vi "GainCurveMeasurement.vi"() -> ()   [LabVIEW 2020]
doc: "Main VI for FLS imaging system."
uses:
  <userlib>/_OpenG.lib/file/file.llb/openg_file.lvlib
  <vilib>/event_ctls.llb/usereventprio.ctl
  <instrlib>/niScope/Acquire/Fetch/niScope Multi Fetch Binary 16.vi
  <instrlib>/niScope/Controls/niScope trigger source.ctl
  <userlib>/_OpenG.lib/time/time.llb/openg_time.lvlib
  <vilib>/Utility/file.llb/Write Delimited Spreadsheet (DBL).vi
  LaguerreDeconLib/DeconEngineClass/LaguerreDeconEngineClass.lvclass
  SubVI/GlobalVariables.vi
  SubVI/LabJack/LJ Pin Setting.ctl
  <vilib>/Utility/error.llb/DialogType.ctl
  <vilib>/Analysis/NI_AALBase.lvlib
  <vilib>/Utility/miscctls.llb/LVMinMaxIncTypeDef.ctl
  <vilib>/Analysis/baseanly.llb/Mean (DBL).vi
  <vilib>/Utility/miscctls.llb/LVPointTypeDef.ctl
  <vilib>/Instr/_visa.llb/VISA Configure Serial Port (Instr).vi
  SubVI/DigitizerConfiguration/FLImDAQ.ctl
panel:
  out "Record Backlog":i32
  out "Fetch Record #":i32
  out "error out 2":errorcluster caption="error out"
  out "error out":errorcluster
  out "Sync Success?":bool
  out "Disclamer":picture
  out "Calibration #":i8
  out "BG #":i8
  in  "TCP Connect":bool
  out "Help":string
  in  "355nm Laser toggle":bool caption="355nm 750Hz"
  in  "Cali&iRF alignment":bool
  in  "Background":bool
  in  "Aiming beam toggle":bool caption="445nm 15Hz 20mA"
  out "Lifetime 3":dbl
  out "Lifetime 2":dbl
  in  "Auto gain ch3":bool=TRUE
  in  "Auto gain ch2":bool=TRUE
  in  "Auto gain ch1":bool=TRUE
  out "Run #":i8
  in  "StopButton":bool caption="Stop"
  out "Aquisition Status:":bool
  in  "StartButton":bool caption="Start"
  in  "Gain 3":dbl min=0.0 max=4.6 step=0.1
  in  "Gain 2":dbl min=0.0 max=4.6 step=0.1
  out "Lifetime 1":dbl
  in  "Gain 1":dbl min=0.0 max=4.6 step=0.1 format="%#_4g"
  in  "Video Source":enum32{"Camera", "FrameGrabber"}(radio)
  out "Case #":string
  out "System Hardware Connection Status":T1
  out "Channel 3":dbl[][](graph)
  out "Channel 2":dbl[][](graph)
  out "Channel 1":dbl[][](graph)
  in  "Tab Control":T2(tab)
  out "Aq L?":bool
  out "ML?":bool
  out "display loop timing(ms)":u32
  out "Aquisition loop timing(ms)":u32
  in  "sine offset":dbl min=0.0 max=4.8 step=0.01
  in  "sine amplitude":dbl
  out "DisplayLoop":i32
  out "processing loop":i32
  out "processing loop timing(ms)":dbl
  in  "V target(1.5)":dbl=1.3 format="%#_13g"
  out "comm loop(ms)":u32
  out "laser EM lamp V":dbl format="%0.6f"
  in  "Show BG":bool
  in  "start Idx":i32
  in  "length":i32=50
  out "SysConfigCluster":T3
  out "LJ Pinout":T4={"Ch1 Bias"="DAC0", "Ch2 Bias"="DAC1", "Ch3 Bias"="DAC2", "Ch4 Bias"="DAC0", "355 PWM"="FIO0", "AimingBeam PWM"="FIO2", "Laser Ready"="FIO3", "Interlock"="FIO1", "Laser Start/Stop"="FIO1", "Red LED"="FIO1", "Green LED"="DIO3", "Foot Pedal"="DIO15"}
  out "FLImDAQ":T5={"Digitizer 1"="", "Digitizer 2"="", "Channel"=enum."Channel 0", "trigger source"="VAL_EXTERNAL", "trigger level"=0.5, "trigger delay"=1.35e-07, "min sample rate"=12500000000.0, "min record length"=2500, "vertical range"=1.0, "vertical offset"=-0.25, "Waveform to Avg"=2000} caption="FLIm DAQ Configuration" {"trigger delay" format="%^#.4e"; "trigger level" min=0.0 max=3.5 step=0.5 format="%.2f"; "vertical offset" format="%.4f"; "vertical range" format="%.2f"; "min sample rate" format="%#.2p"}
  out "Dig1 Temp":dbl
  out "Dig2 Temp":dbl
  in  "Sys Reconfig":bool
  out "data out(communcation loop)":string
  out "syctimer data out":string
  out "processing Error Out":errorcluster
  out "aquisition loop Error Out":errorcluster
  out "decon error out":errorcluster
  out "V1":dbl[](array[numeric])
  out "V2":dbl[](array[numeric])
  out "V3":dbl[](array[numeric])
  out "V1 Size":i32
  out "V2 Size":i32
  out "V3 Size":i32
  out "data Size":i32[](array[numeric])
  out "State log":string
  in  "Quit":bool
  in  "Radio Buttons":enum32{"No Selection", "Ch1", "Ch2", "Ch3"}(radio)=enum."Ch1" caption="DeCon Chan"
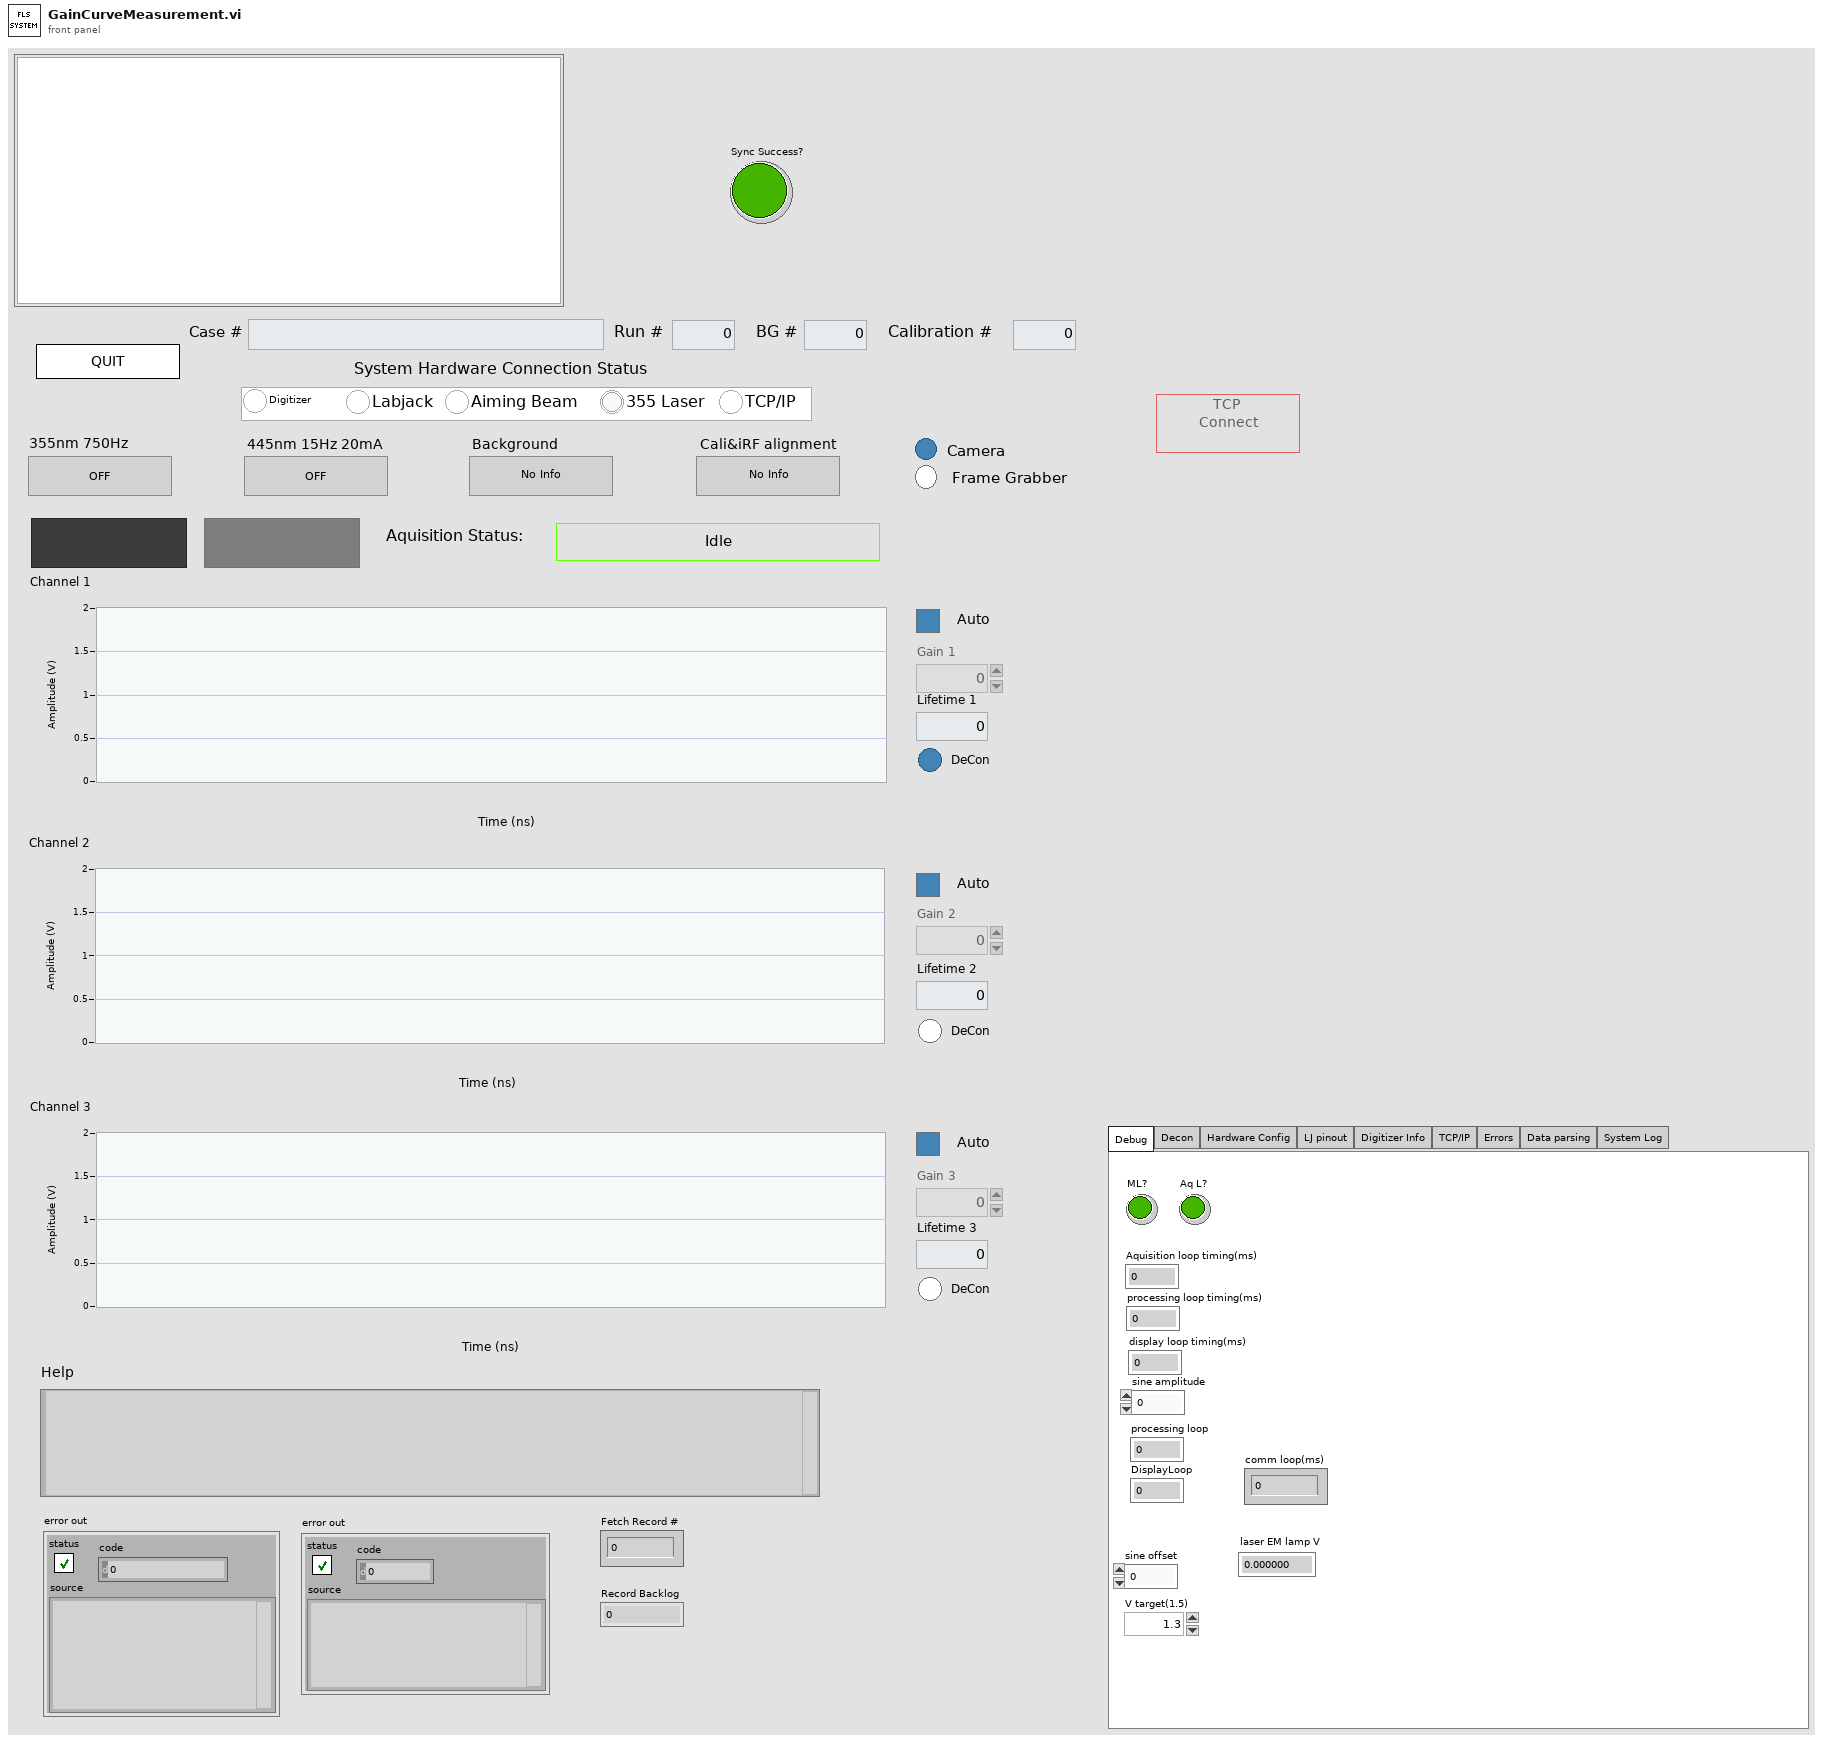
[diagram p1: front panel]
types:
  T1 = cluster{"Digitizer":bool, "Labjack":bool, "Aiming Beam":bool, "355 Laser":bool, "TCP/IP":bool}
  T2 = enum32{"Debug", "Decon", "Hardware Config", "LJ pinout", "Digitizer Info", "TCP/IP", "Errors", "Data parsing", "System Log"}
  T3 = cluster{"Ch1Enable?":bool, "Ch2Enable?":bool, "Ch3Enable?":bool, "Ch1AutoGain?":bool, "Ch2AutoGain?":bool, "Ch3AutoGain?":bool, "AimingBeamEnable?":bool}
  T4 = typedef "LJ Pin Setting.ctl" = cluster{"Ch1 Bias":string, "Ch2 Bias":string, "Ch3 Bias":string, "Ch4 Bias":string, "355 PWM":string, "AimingBeam PWM":string, "Laser Ready":string, "Interlock":string, "Laser Start/Stop":string, "Red LED":string, "Green LED":string, "Foot Pedal":string}
  T5 = typedef "FLImDAQ.ctl" = cluster{"Digitizer 1":refnum<k15>, "Digitizer 2":refnum<k15>, "Channel":enum16{"Channel 0", "Channel 1", "Channel 0&1"}, "trigger source":T6, "trigger level":dbl, "trigger delay":dbl, "min sample rate":dbl, "min record length":i32, "vertical range":dbl, "vertical offset":dbl, "Waveform to Avg":i16}
  T6 = typedef "niScope trigger source.ctl" = string
  T7 = typedef "LVPointTypeDef.ctl" = cluster{"Horizontal":i16, "Vertical":i16}
  T8 = cluster{"CH1":dbl[][], "CH2":dbl[][], "CH3":dbl[][]}
  T9 = cluster{"idx":i32, "CH1&2":dbl[][], "CH3":dbl[][]}
  T10 = enum8{"Enabled", "Disabled", "Disabled and Grayed Out"}
  T11 = enum16{"open", "open or create", "create or replace", "create", "open (read-only)"}
  T12 = enum32{"Invalid", "Standard", "Closed", "Hidden", "Minimized", "Maximized"}
  T13 = enum32{"invalid app kind", "Development System", "Run Time System", "Student Edition", "Embedded LabVIEW", "Evaluation", "Custom"}
  T14 = typedef "usereventprio.ctl" = enum32{"high priority", "normal priority"}
  T15 = enum16{"Standard", "Buffered", "CRLF", "Immediate"}
  T16 = cluster{"Core":cluster{"Current VI Reference":refnum<vi>, "Close Panel on Exit?":bool}, "SysConfigCluster":cluster{"Ch1Enable?":bool, "Ch2Enable?":bool, "Ch3Enable?":bool, "Ch1AutoGain?":bool, "Ch2AutoGain?":bool, "Ch3AutoGain?":bool, "AimingBeamEnable?":bool}, "System Status":cluster{"Digitizer":bool, "Labjack":bool, "Aiming Beam":bool, "355 Laser":bool, "TCP/IP":bool}, "IDs":cluster{"RunID":i8, "BG ID":i8, "Cali ID":i8}, "CaseID":string, "DefaultPath":path, "Pathes":cluster{"DataPath":path, "BG Path":path, "iRFPath":path, "CaliPath":path}, "FLImDAQ":cluster{"resource name":refnum<k15>, "resource name 2":refnum<k15>, "Channel":enum16{"Channel 0", "Channel 1", "Channel 0&1"}, "trigger source":T6, "trigger level":dbl, "trigger delay":dbl, "min sample rate":dbl, "min record length":i32, "vertical range":dbl, "vertical offset":dbl, "Waveform to Avg":i32}, "SysRunning?":bool, "AB Cluster":cluster{"Aiming Beam COM Port":refnum<visa-resource-name>, "Min Current":dbl, "Max Current":dbl, "Default Current":dbl, i32}, "LJ Pinout":T4, "355 PWM setting":cluster{"DIO_EF_CLOCK1_DIVISOR":i16, "DIO_EF_CLOCK1_ROLL_VALUE":i32, "DIO#_EF_INDEX":i16, "DIO#_EF_OPTIONS":i16, "DIO#_EF_CONFIG_A":i32}, "AB PWM setting":cluster{"DIO_EF_CLOCK1_DIVISOR":i16, "DIO_EF_CLOCK1_ROLL_VALUE":i32, "DIO#_EF_INDEX":i16, "DIO#_EF_OPTIONS":i16, "DIO#_EF_CONFIG_A":i32}, "Last Trigger":u32, "niTClk sessions":refnum<k20>[], "Laser start tic":u32, "TCP attempt count":i32, "Ch1Data":dbl[][], "Ch2Data":dbl[][], "Ch3Data":dbl[][], "V1":dbl[], "V2":dbl[], "V3":dbl[], "SlowTimer":u32, "FastTimer":u32, "listener ID":refnum<k5>, "TempPath":path, "LED vi reference":refnum<vi>}
  T17 = typedef "LVCursorListTypeDef.ctl" = cluster{"Name":string, "Color":u32, "Style":u8, "Point Style":u8, "Name Visible":bool, "Allow Drag":bool, "Cursor Mode":u32, "Plot":i32, "Index":i32, "Position":cluster{"X":dbl, "Y":dbl}, "X Scale":u32, "Y Scale":u32, "Watch Plots":i32[], "Watch All Plots":bool, "Plot Area":i32, "Label Offset":cluster{"X":dbl, "Y":dbl}}[]
  T18 = cluster{"Name":string, "Color":u32, "Style":u8, "Point Style":u8, "Name Visible":bool, "Allow Drag":bool, "Cursor Mode":u32, "Plot":i32, "Index":i32, "Position":cluster{"X":dbl, "Y":dbl}, "X Scale":u32, "Y Scale":u32, "Watch Plots":i32[], "Watch All Plots":bool, "Plot Area":i32, "Label Offset":cluster{"X":dbl, "Y":dbl}}
  T19 = cluster{"DataPath":path, "BG Path":path, "iRFPath":path, "CaliPath":path}
  T20 = cluster{"DIO_EF_CLOCK1_DIVISOR":i16, "DIO_EF_CLOCK1_ROLL_VALUE":i32, "DIO#_EF_INDEX":i16, "DIO#_EF_OPTIONS":i16, "DIO#_EF_CONFIG_A":i32}
  T21 = cluster{"Aiming Beam COM Port":refnum<visa-resource-name>, "Min Current":dbl, "Max Current":dbl, "Default Current":dbl, i32}
  T22 = cluster{"resource name":refnum<k15>, "resource name 2":refnum<k15>, "Channel":enum16{"Channel 0", "Channel 1", "Channel 0&1"}, "trigger source":T6, "trigger level":dbl, "trigger delay":dbl, "min sample rate":dbl, "min record length":i32, "vertical range":dbl, "vertical offset":dbl, "Waveform to Avg":i32}
  T23 = cluster{"Current VI Reference":refnum<vi>, "Close Panel on Exit?":bool}
  T24 = cluster{"1D Avg out":dbl[], "1D Avg out":dbl[], "1D Avg out":dbl[]}
  T25 = typedef "DialogType.ctl" = u16
  T26 = cluster{"Ch1 iRF":dbl[], "Ch2 iRF":dbl[], "Ch3 iRF":dbl[], "Ch4 iRF":dbl[]}
  T27 = typedef "LJ PWM Setting.ctl" = cluster{"DIO_EF_CLOCK1_DIVISOR":i16, "DIO_EF_CLOCK1_ROLL_VALUE":i32, "DIO#_EF_INDEX":i16, "DIO#_EF_OPTIONS":i16, "DIO#_EF_CONFIG_A":i32}
  T28 = typedef "AimingBeam.ctl" = cluster{"Aiming Beam COM Port":refnum<visa-resource-name>, "Min Current":dbl, "Max Current":dbl, "Default Current":dbl, "Frequency(Hz)":u32}
  T29 = typedef "LVMinMaxIncTypeDef.ctl" = cluster{"Minimum":dbl, "Maximum":dbl, "Increment":dbl}
  T30 = typedef "LVBoundsTypeDef.ctl" = cluster{"Width":u32, "Height":u32}
  T31 = typedef "imagedata.ctl" = cluster{"image type":i32, "image depth":i32, "image":u8[], "mask":u8[], "colors":u32[], "Rectangle":cluster{"left":i16, "top":i16, "right":i16, "bottom":i16}}
  T32 = enum32{"No Selection", "Ch1", "Ch2", "Ch3", "Ch4"}
  T33 = cluster{"V1 out":dbl, "V2 out":dbl, "V3 out":dbl}
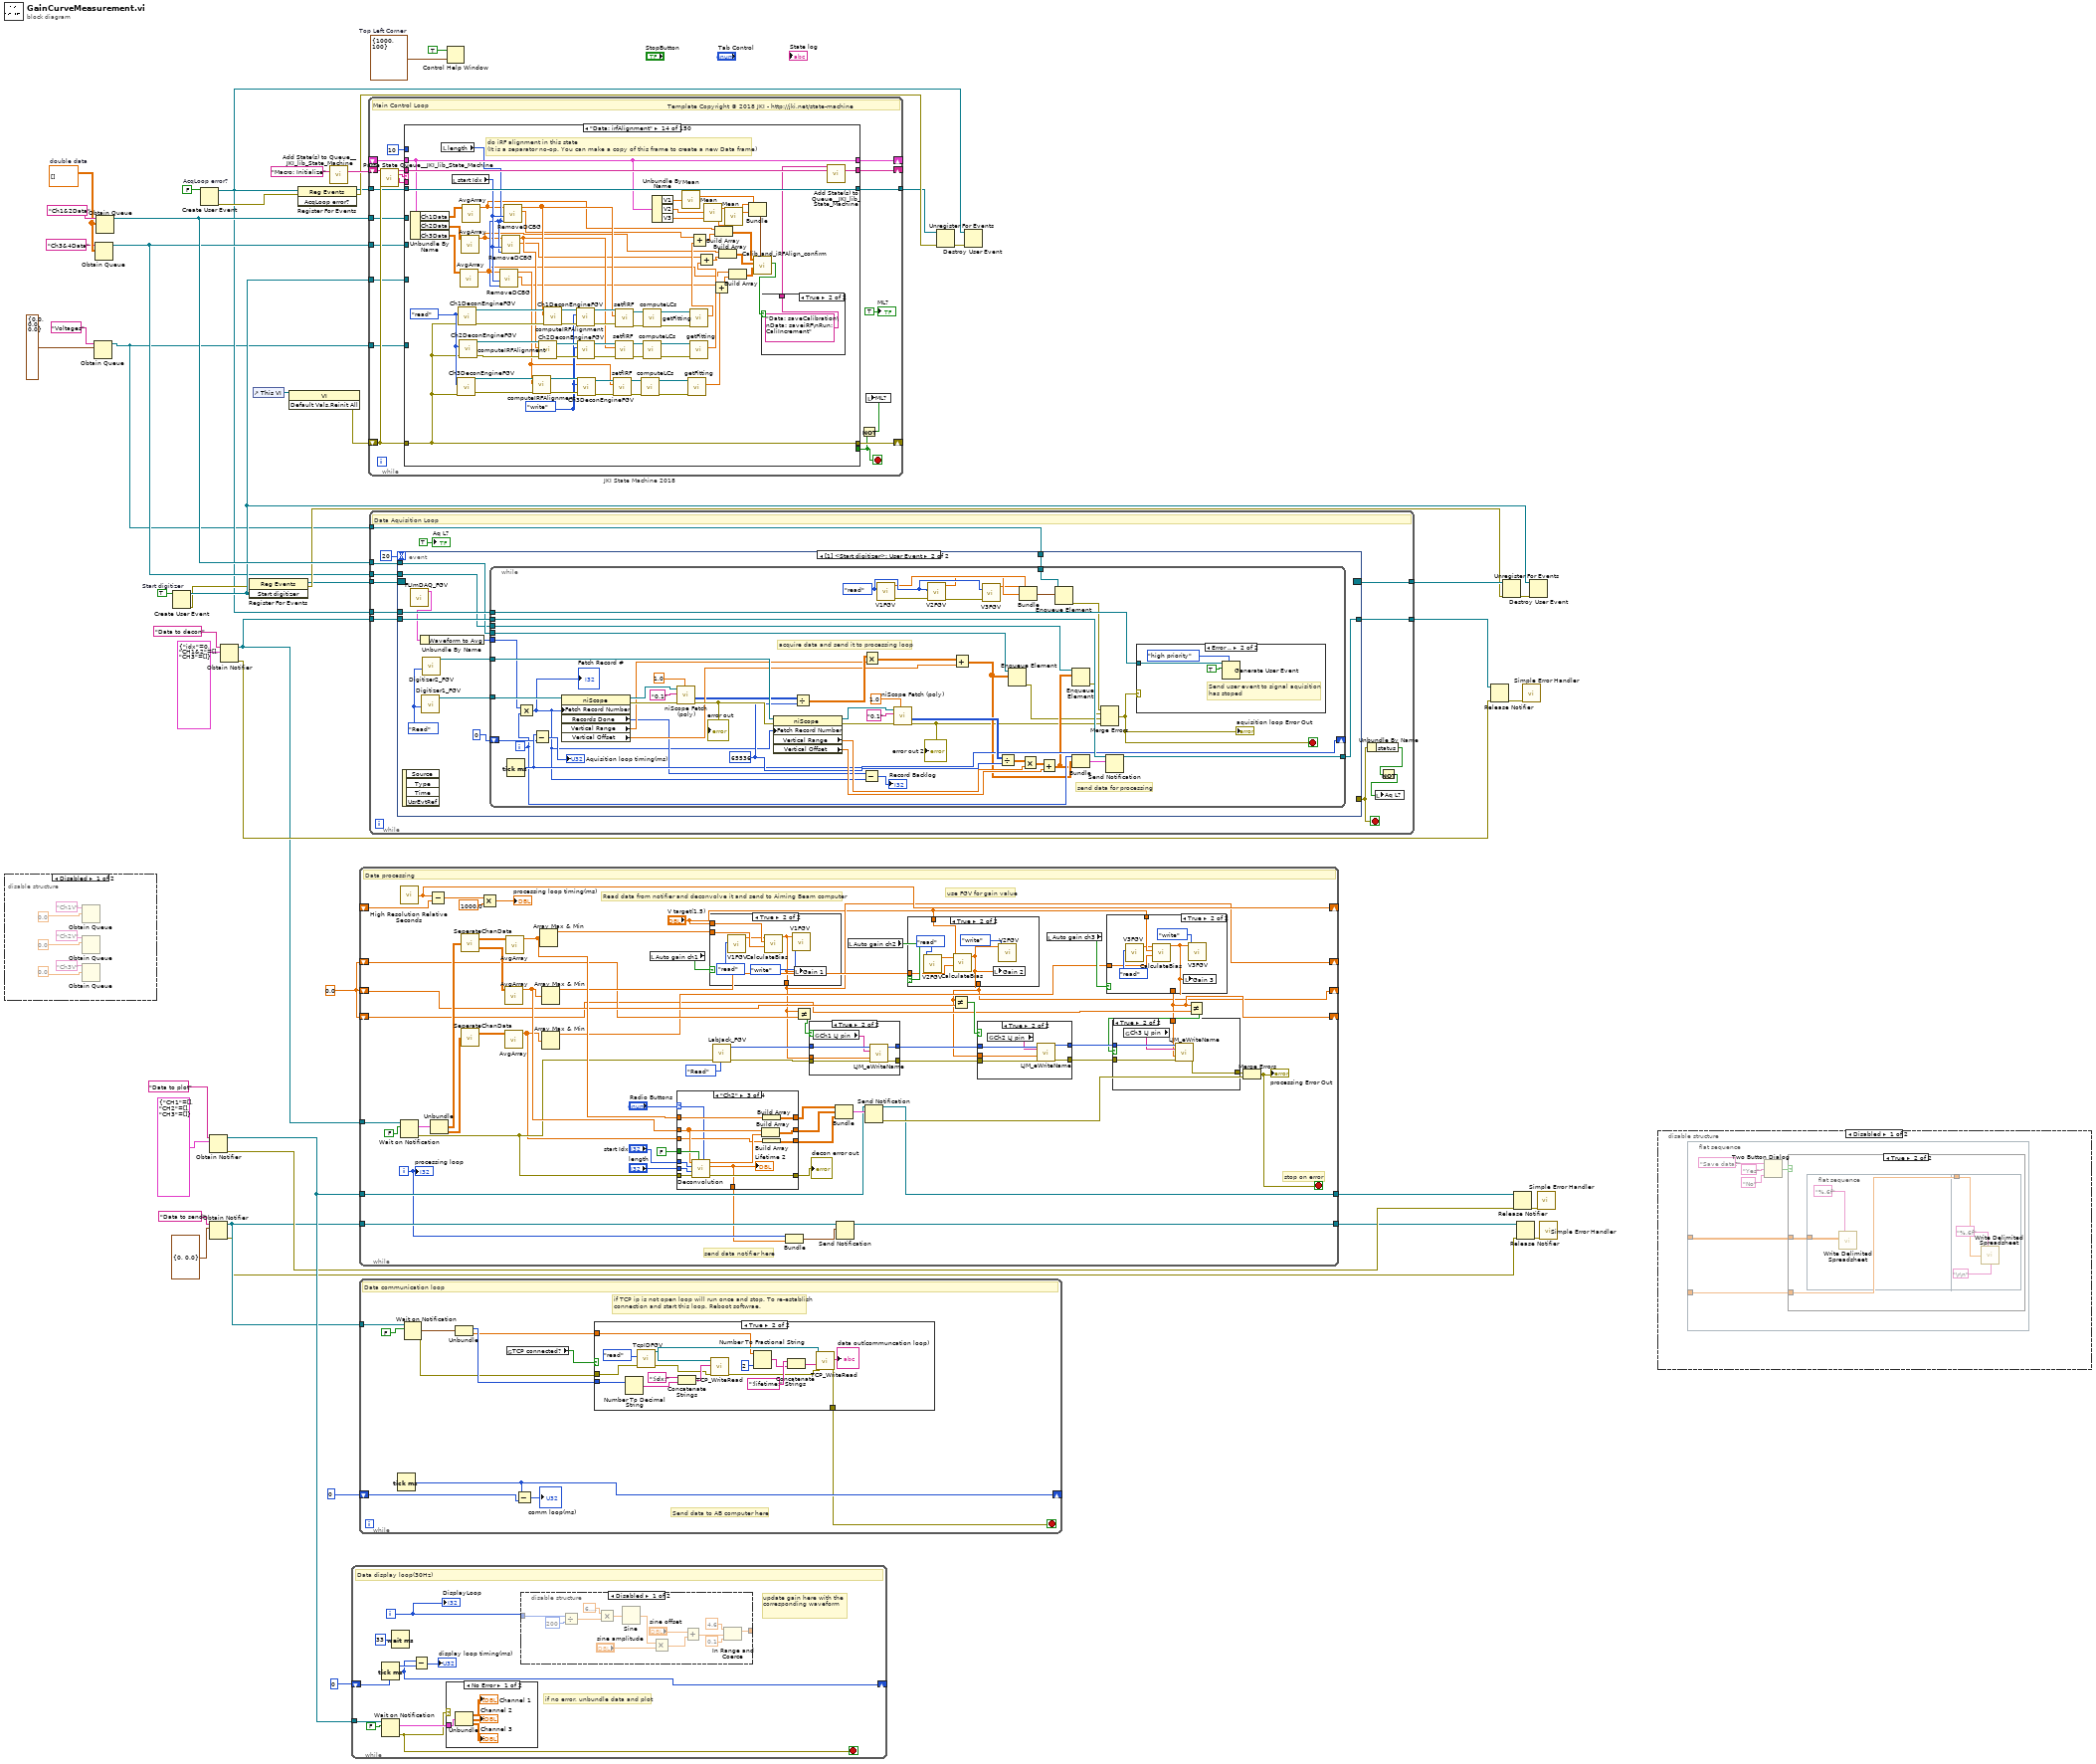
[diagram p0: block diagram]
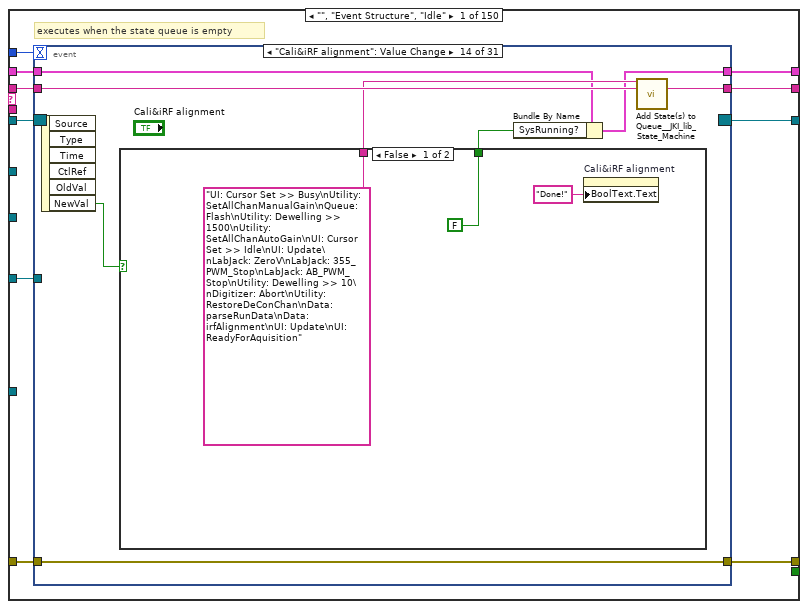
[diagram p3: hidden frame]
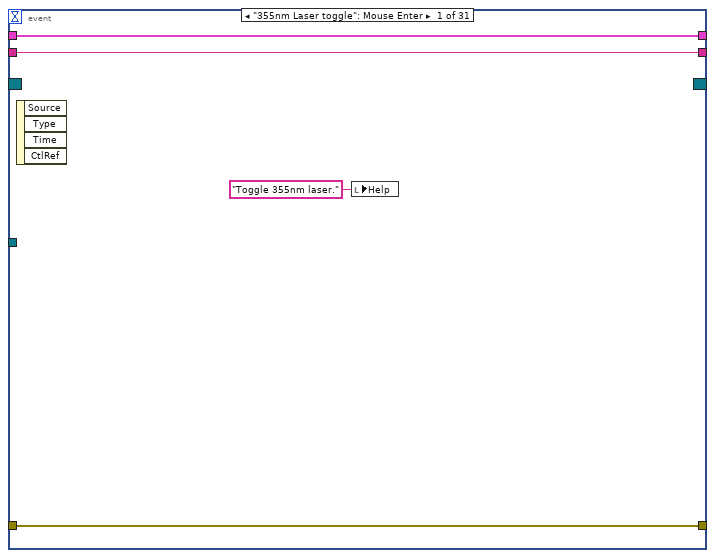
[diagram p4: hidden frame]
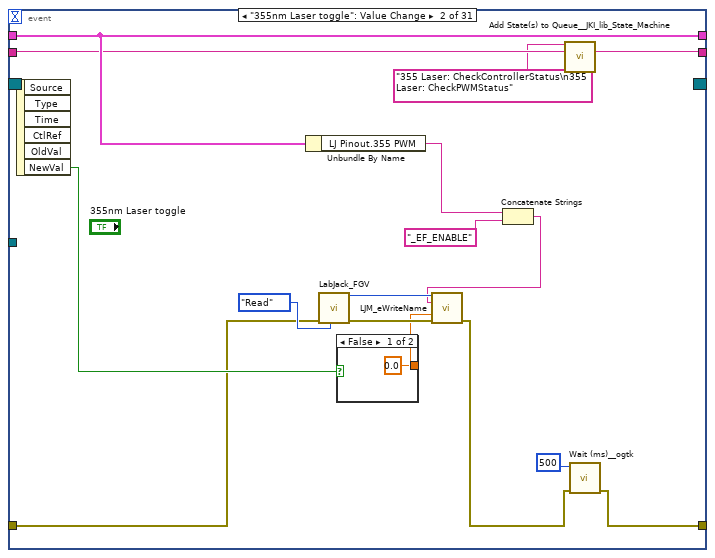
[diagram p5: hidden frame]
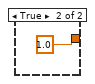
[diagram p6: hidden frame]
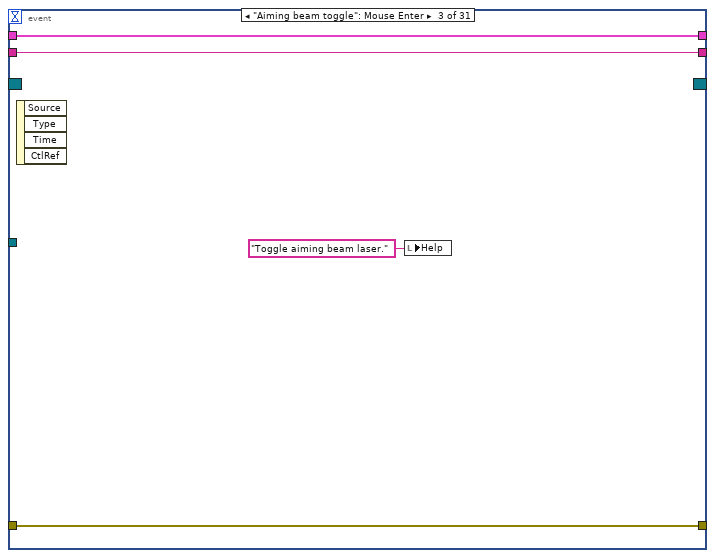
[diagram p7: hidden frame]
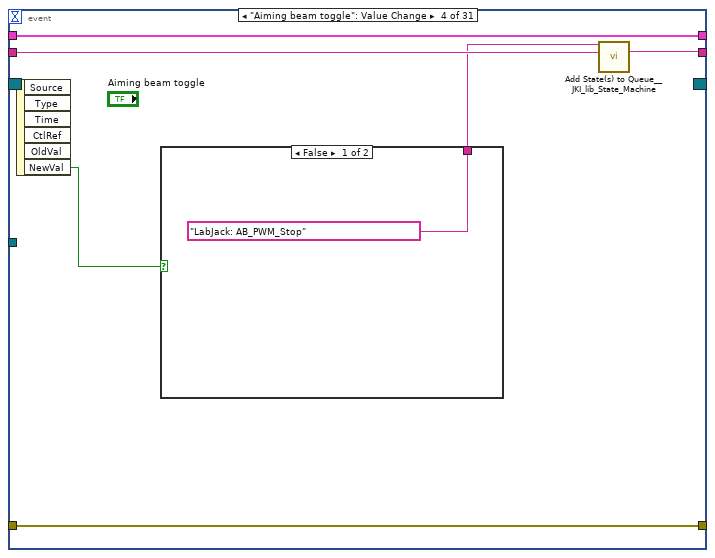
[diagram p8: hidden frame]
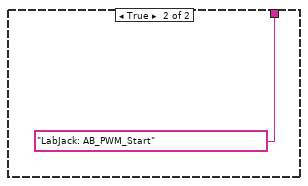
[diagram p9: hidden frame]
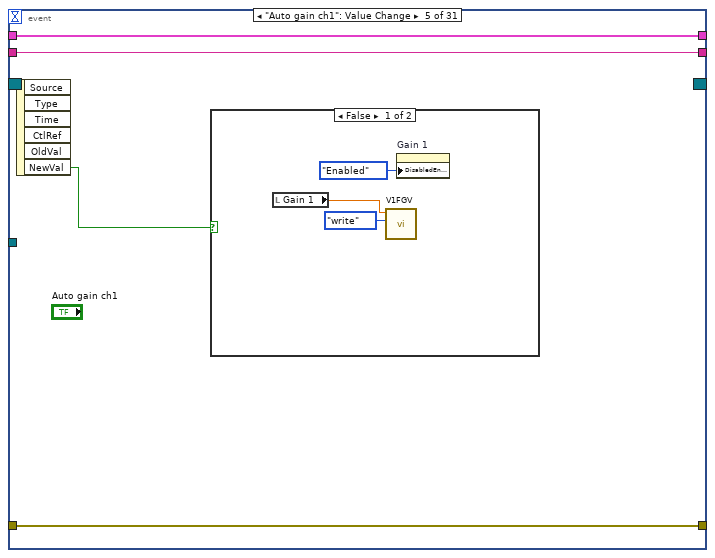
[diagram p10: hidden frame]
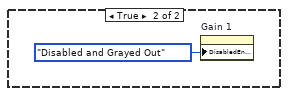
[diagram p11: hidden frame]
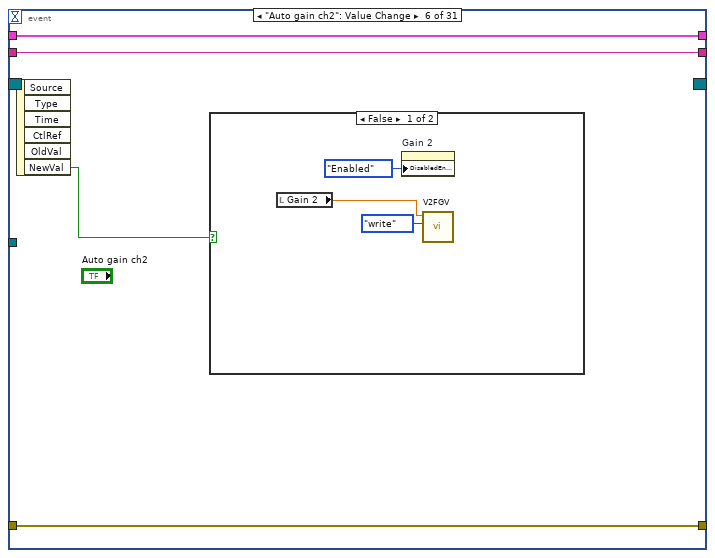
[diagram p12: hidden frame]
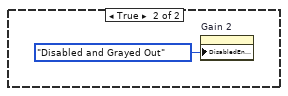
[diagram p13: hidden frame]
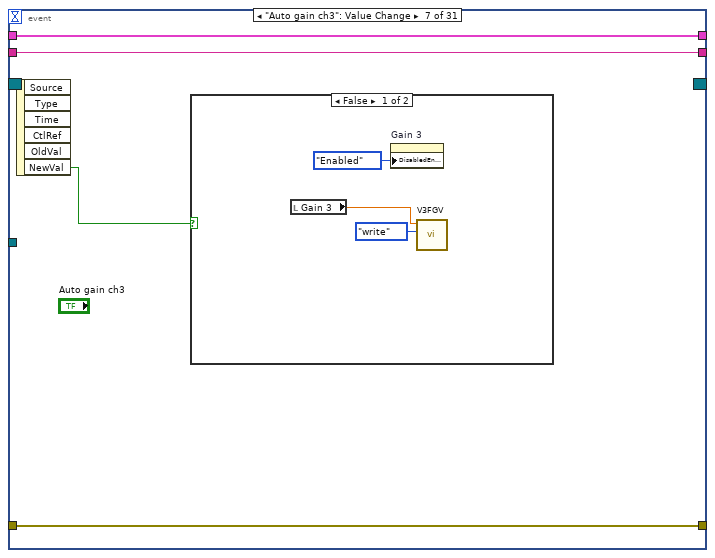
[diagram p14: hidden frame]
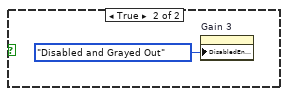
[diagram p15: hidden frame]
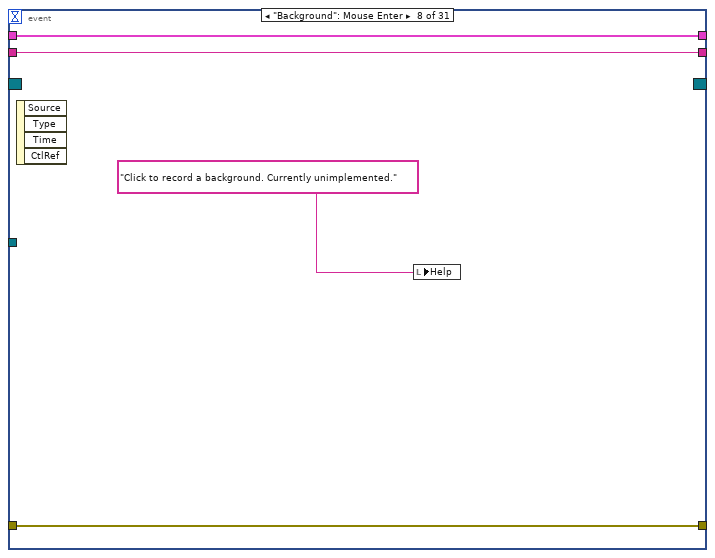
[diagram p16: hidden frame]
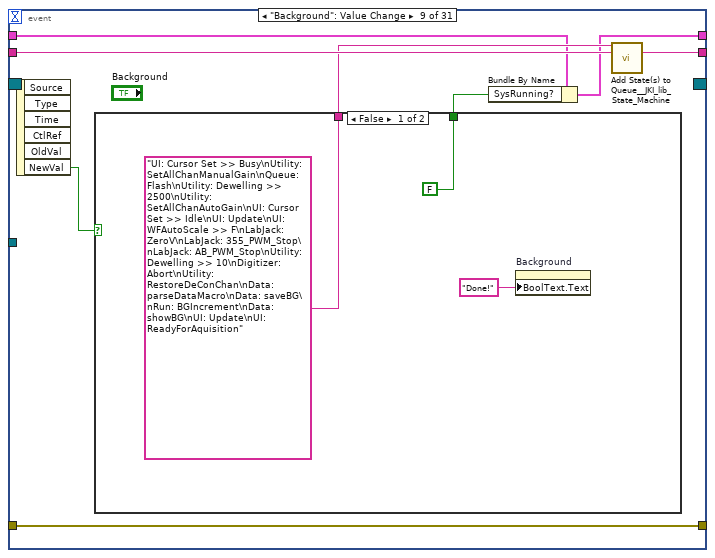
[diagram p17: hidden frame]
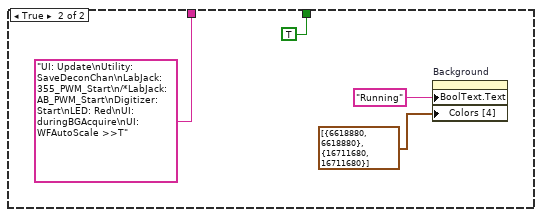
[diagram p18: hidden frame]
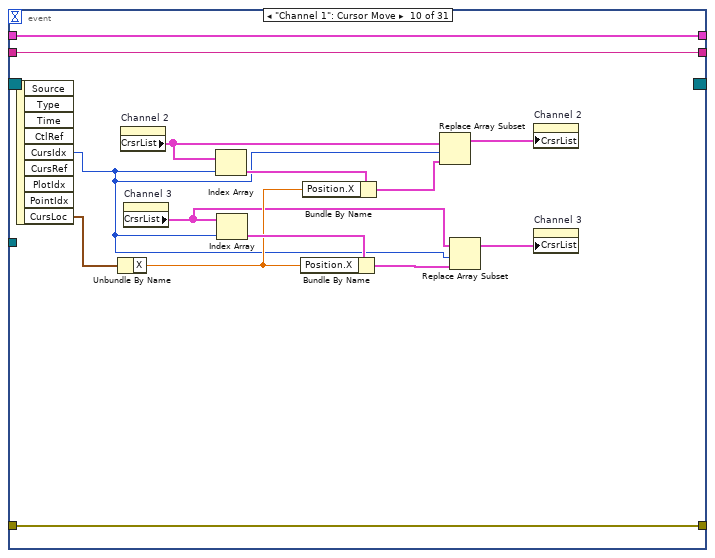
[diagram p19: hidden frame]
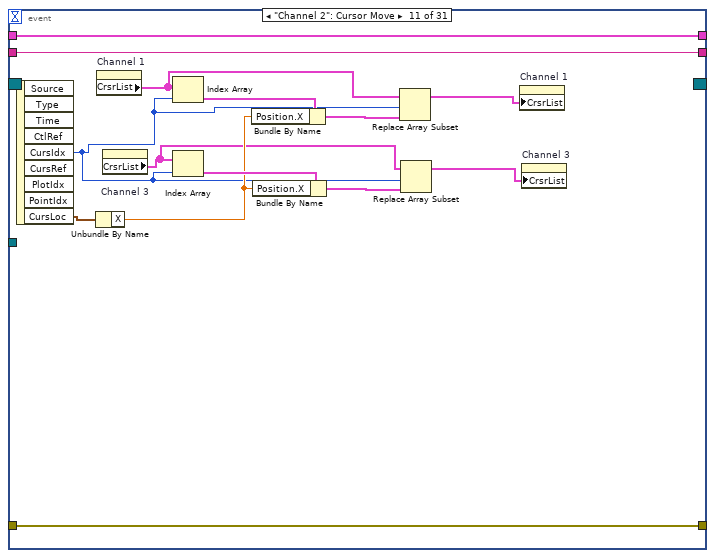
[diagram p20: hidden frame]
diagram:
  w1 = T7 {"Horizontal"=1000, "Vertical"=100}  # Top Left Corner
  w6 = 0.0
  w31 = FALSE  # AcqLoop error?
  w42 = TRUE  # Start digitizer
  w45 = dbl[][] []  # double data
  n1 = disable-structure shown="Disabled" {
    frame Disabled {
      n2 = Obtain Queue(name (unnamed)="Ch1V", element data type=0.0) -> ()  [unwired: 3 in, 3 out]
      n3 = Obtain Queue(name (unnamed)="Ch2V", element data type=0.0) -> ()  [unwired: 3 in, 3 out]
      n4 = Obtain Queue(name (unnamed)="Ch3V", element data type=0.0) -> ()  [unwired: 3 in, 3 out]
    }
    frame Enabled {
    }
  }
  n5 = Obtain Queue(name (unnamed)="Voltages", element data type=cluster{"V1":dbl, "V2":dbl, "V3":dbl} {"V1"=0.0, "V2"=0.0, "V3"=0.0}) -> (queue out=w3:refnum<queue>)  [unwired: 3 in, 2 out]
  n6 = Obtain Queue(name (unnamed)="Ch3&4Data", element data type=w45) -> (queue out=w19:refnum<queue>)  [unwired: 3 in, 2 out]
  n7 = Obtain Queue(name (unnamed)="Ch1&2Data", element data type=w45) -> (queue out=w43:refnum<queue>)  [unwired: 3 in, 2 out]
  n8 = Create User Event(user event datatype=w42) -> (user event=w30:refnum<user-event>, error out=w9:errorcluster)  [unwired: 1 in]
  n9 = Create User Event(user event datatype=w31) -> (user event=w8:refnum<user-event>, error out=w10:errorcluster)  [unwired: 1 in]
  n10 = Obtain Notifier(name (unnamed)="Data to plot", notification data type=T8 {"CH1"=[], "CH2"=[], "CH3"=[]}) -> (notifier out=w23:refnum<notifier>, error out=w20:errorcluster)  [unwired: 2 in, 1 out]
  n11 = Obtain Notifier(name (unnamed)="Data to send", notification data type=cluster{"idx":i32, "lifetime":dbl} {"idx"=0, "lifetime"=0.0}) -> (notifier out=w14:refnum<notifier>, error out=w7:errorcluster)  [unwired: 2 in, 1 out]
  n12 = Obtain Notifier(name (unnamed)="Data to decon", notification data type=T9 {"idx"=0, "CH1&2"=[], "CH3"=[]}) -> (notifier out=w26:refnum<notifier>, error out=w36:errorcluster)  [unwired: 2 in, 1 out]
  n13 = register-events(error in=w9, w30) -> (reference out=w32:refnum<event-registration>, error out=w39:errorcluster)  [unwired: 1 in]
  n14 = control-ref of="This VI"() -> (w47:refnum<vi>)
  n15 = invoke class="VI" method="Default Vals.Reinit All"(reference=w47) -> (error out=w33:errorcluster)  [unwired: 2 in, 2 out]
  n16 = register-events(error in=w10, w8) -> (reference out=w18:refnum<event-registration>, error out=w28:errorcluster)  [unwired: 1 in]
  n17 = call <vilib>:"Add State(s) to Queue__JKI_lib_State_Machine.vi"("State(s) in (\"\")"="Macro: Initialize") -> ("States Out"=w49:string)  [unwired: 14 in]
  n18 = while {
    tunnel: w23 -> [w64]
    shift-right: [w57] -> _
    shift-left: u32 0 ("millisecond timer value") -> [w62]
    i -> [w60]
    stop <- w56 stop-if-true
    # "if no error, unbundle data and plot"
    # "update gain here with the corresponding waveform"
    # "Data display loop(30Hz)"
    n19 = Tick Count (ms)() -> (millisecond timer value=w57:u32)
    n20 = Wait on Notification(notifier=w64, ignore previous (F)=FALSE) -> (notification=w58:T8, error out=w56:errorcluster)  [unwired: 2 in, 2 out]
    n21 = Wait (ms)(milliseconds to wait=u32 33) -> ()  [unwired: 1 out]
    n22 = Subtract(x=w57, y=w62) -> (x-y=→"display loop timing(ms)":u32)
    n23 = case shown="No Error" w56 {
      tunnel: w58 -> [w68 _]
      frame No Error {
        n24 = Unbundle(w68) -> ("CH1"=→"Channel 1":dbl[][], "CH2"=→"Channel 2":dbl[][], "CH3"=→"Channel 3":dbl[][])
      }
      frame Error {
      }
    }
    n25 = disable-structure shown="Disabled" {
      disable-tunnel: w60 -> [w70 _]
      disable-tunnel: [w69 _] -> _
      frame Disabled {
        n26 = Divide(x=w70, y=200) -> (x/y=w80:dbl)
        n27 = Multiply(x=6.283185307179586, y=w80) -> (x*y=w78:dbl)
        n28 = Sine(x=w78) -> (sin(x)=w76:dbl)
        n29 = Multiply(x=w76, y="sine amplitude") -> (x*y=w77:dbl)
        n30 = Add(x="sine offset", y=w77) -> (x+y=w75:dbl)
        n31 = In Range and Coerce(upper limit=4.6, x=w75, lower limit=0.1) -> (coerced(x)=w69:dbl)  [unwired: 1 out]
      }
      frame Enabled {
      }
    }
    "DisplayLoop" <- w60
  }
  n32 = while {
    tunnel: w14 -> [w92]
    shift-right: [w85] -> _
    shift-left: u32 0 -> [w86]
    stop <- w83 stop-if-true
    # "Send data to AB computer here"
    # "if TCP ip is not open loop will run once and stop. To re-establish connection and start this loop. Reboot softwrae."
    # "Data communication loop"
    n33 = Tick Count (ms)() -> (millisecond timer value=w85:u32)
    n34 = Wait on Notification(notifier=w92, ignore previous (F)=FALSE) -> (notification=w90:cluster{"idx":i32, "lifetime":dbl}, error out=w84:errorcluster)  [unwired: 2 in, 2 out]
    n35 = Unbundle(w90) -> ("idx"=w89:i32, "lifetime"=w88:dbl)
    n36 = global read "GlobalVariables.vi" "TCP connected?"() -> (w82:bool)
    n37 = Subtract(x=w85, y=w86) -> (x-y=→"comm loop(ms)":u32)
    n38 = case shown="True" w82 {
      tunnel: w89 -> [_ w101]
      tunnel: w88 -> [_ w100]
      tunnel: w84 -> [w93 w97]
      tunnel: [w93 w94] -> w83
      frame False {
      }
      frame True {
        n39 = Number To Decimal String(number=w101) -> (decimal integer string=w109:string)  [unwired: 1 in]
        n40 = call "TcpIDFGV.vi"("Error In"=w97, "action"=enum16{"write", "read"}."read") -> ("Error Out"=w96:errorcluster, "connection ID out"=w107:refnum<k5>)  [unwired: 8 in]
        n41 = Concatenate Strings("!idx:", w109) -> (w110:string)
        n42 = call "TCP_WriteRead.vi"("error in (no error)"=w96, "data in"=w110, "connectin ID in"=w107) -> ("error out"=w95:errorcluster, "connectin ID out"=w108:refnum<k5>)  [unwired: 4 in, 1 out]
        n43 = Number To Fractional String(number=w100, precision (6)=i16 2) -> (F-format string=w99:string)  [unwired: 2 in]
        n44 = Concatenate Strings("!lifetime:", w99) -> (w106:string)
        n45 = call "TCP_WriteRead.vi"("error in (no error)"=w95, "data in"=w106, "connectin ID in"=w108) -> ("error out"=w94:errorcluster, "data out"=→"data out(communcation loop)":string)  [unwired: 4 in, 1 out]
      }
    }
  }
  n46 = while {
    tunnel: w26 -> [w169]
    shift-right: [w114] -> _
    shift-left: w6 -> [w121]
    tunnel: w23 -> [w161]
    tunnel: [w158] -> w22
    shift-right: [w157] -> _
    shift-left: _ -> [w156]
    shift-right: [w115] -> _
    shift-left: w6 -> [w122]
    shift-right: [w116] -> _
    shift-left: w6 -> [w118]
    tunnel: w14 -> [w134]
    tunnel: [w130] -> w13
    i -> [w133]
    stop <- w129 stop-if-true
    # "use FGV for gain value"
    # "send data notifier here"
    # "stop on error"
    # "Read data from notifier and deconvolve it and send to Aiming Beam computer"
    # "Data processing"
    n47 = call <vilib>:"High Resolution Relative Seconds.vi"() -> ("relative seconds"=w157:dbl)
    n48 = Wait on Notification(notifier=w169, ignore previous (F)=FALSE) -> (notification=w167:T9, error out=w146:errorcluster)  [unwired: 2 in, 2 out]
    n49 = Subtract(x=w157, y=w156) -> (x-y=w155:dbl)
    n50 = Unbundle(w167) -> ("CH1&2"=w136:dbl[][], "CH3"=w135:dbl[][])  [unwired: 1 out]
    n51 = call "SeperateChanData.vi"("Input (Ch1&2)"=w136) -> ("Ch1"=w138:dbl[][], "Ch2"=w143:dbl[][])
    n52 = call "SeperateChanData.vi"("Input (Ch1&2)"=w135) -> ("Ch1"=w166:dbl[][])  [unwired: 1 out]
    n53 = Multiply(x=w155, y=1000.0) -> (x*y=→"processing loop timing(ms)":dbl)
    n54 = call "AvgArray.vi"("2D array in"=w143) -> ("1D Avg out"=w152:dbl[])  [unwired: 10 in]
    n55 = call "AvgArray.vi"("2D array in"=w166) -> ("1D Avg out"=w142:dbl[])  [unwired: 10 in]
    n56 = call "AvgArray.vi"("2D array in"=w138) -> ("1D Avg out"=w159:dbl[])  [unwired: 10 in]
    n57 = Array Max & Min(array=w159) -> (max value=w125:dbl)  [unwired: 3 out]
    n58 = Array Max & Min(array=w152) -> (max value=w123:dbl)  [unwired: 3 out]
    n59 = Array Max & Min(array=w142) -> (max value=w119:dbl)  [unwired: 3 out]
    n60 = local read "Auto gain ch1"() -> (w128:bool)
    n61 = case shown="\"Ch2\"" "Radio Buttons" {
      selector: "Radio Buttons" -> [_ w224 w238 w252]
      tunnel: w159 -> [w223 w232 w244 w257]
      tunnel: w152 -> [w221 w229 w246 w255]
      tunnel: w142 -> [w219 w227 w241 w260]
      tunnel: FALSE -> [_ w237 w251 w265]
      tunnel: w146 -> [w217 w236 w248 w262]
      tunnel: "length" -> [_ w235 w249 w263]
      tunnel: "start Idx" -> [_ w234 w250 w264]
      tunnel: [w217 w233 w247 w261] -> w137
      tunnel: [w222 w230 w242 w256] -> w141
      tunnel: [w220 w228 w243 w254] -> w140
      tunnel: [w218 w226 w240 w258] -> w139
      tunnel: [0.0 ("lifetime (ns)") w225 w239 w253] -> w132
      frame "No Selection", Default {
        n62 = Build Array(w223) -> (w222:dbl[][])
        n63 = Build Array(w221) -> (w220:dbl[][])
        n64 = Build Array(w219) -> (w218:dbl[][])
      }
      frame "Ch1" {
        n65 = call "Deconvolution.vi"("DeconChannel"=w224, "iRF align"=w237, "error in (no error)"=w236, 9:w235, 10:w234, "Waveform"=w232) -> ("error out"=w233:errorcluster, "lifetime (ns)"=w225:dbl, "Fitting"=w231:dbl[])  [unwired: 3 in]
        "Lifetime 1" <- w225
        n66 = Build Array(w232, w231) -> (w230:dbl[][])
        n67 = Build Array(w229) -> (w228:dbl[][])
        n68 = Build Array(w227) -> (w226:dbl[][])
      }
      frame "Ch2" {
        n69 = call "Deconvolution.vi"("DeconChannel"=w238, "iRF align"=w251, "error in (no error)"=w248, 9:w249, 10:w250, "Waveform"=w246) -> ("error out"=w247:errorcluster, "lifetime (ns)"=w239:dbl, "Fitting"=w245:dbl[])  [unwired: 3 in]
        "Lifetime 2" <- w239
        n70 = Build Array(w246, w245) -> (w243:dbl[][])
        n71 = Build Array(w244) -> (w242:dbl[][])
        n72 = Build Array(w241) -> (w240:dbl[][])
      }
      frame "Ch3" {
        n73 = call "Deconvolution.vi"("DeconChannel"=w252, "iRF align"=w265, "error in (no error)"=w262, 9:w263, 10:w264, "Waveform"=w260) -> ("error out"=w261:errorcluster, "lifetime (ns)"=w253:dbl, "Fitting"=w259:dbl[])  [unwired: 3 in]
        "Lifetime 3" <- w253
        n74 = Build Array(w260, w259) -> (w258:dbl[][])
        n75 = Build Array(w257) -> (w256:dbl[][])
        n76 = Build Array(w255) -> (w254:dbl[][])
      }
    }
    "decon error out" <- w137
    n77 = case shown="True" w128 {
      tunnel: [w208 w212] -> w114
      tunnel: w125 -> [_ w214]
      tunnel: "V target(1.5)" -> [_ w213]
      frame False {
        n78 = call "V1FGV.vi"("action (write)"=enum16{"write", "read"}."read" ("action")) -> ("V1 out"=w208:dbl)  [unwired: 9 in, 1 out]
      }
      frame True {
        n79 = call "V1FGV.vi"("action (write)"=enum16{"write", "read"}."read" ("action")) -> ("V1 out"=w210:dbl)  [unwired: 9 in, 1 out]
        n80 = call "CalculateBias.vi"("GainV Last"=w214, "Sig Current(V)"=w213, "GainV current"=w210) -> ("V new"=w212:dbl)  [unwired: 8 in]
        n81 = call "V1FGV.vi"("action (write)"=enum16{"write", "read"}."write" ("action"), "V1 in"=w212) -> ()  [unwired: 8 in, 2 out]
        n82 = local write "Gain 1"(w212) -> ()
      }
    }
    n83 = call "LabJack_FGV.vi"("Operation(Read)"=enum16{"Write", "Read"}."Read" ("Operation"), "error in (no error)"=w146) -> ("error out"=w165:errorcluster, "Read data"=w164:i32)  [unwired: 8 in]
    n84 = Bundle(w133, "lifetime (ns)"=w132) -> (w131:cluster{i32, "lifetime (ns)":dbl})  [unwired: 1 in]
    n85 = Not Equal?(x=w114, y=w121) -> (x != y?=w124:bool)
    n86 = case shown="True" w124 {
      tunnel: w165 -> [w185 w191]
      tunnel: w164 -> [w184 w190]
      tunnel: [w185 w189] -> w151
      tunnel: [w184 w188] -> w148
      tunnel: w114 -> [_ w186]
      frame False {
      }
      frame True {
        n87 = global read "GlobalVariables.vi" "Ch1 LJ pin"() -> (w187:string)
        n88 = call "LJM_eWriteName.vi"("Handle In"=w190, "Name"=w187, "Value"=w186, "error in"=w191) -> ("Handle Out"=w188:i32, "error out"=w189:errorcluster)  [unwired: 10 in]
      }
    }
    n89 = Bundle(w141, w140, w139) -> (w162:cluster{dbl[][], dbl[][], dbl[][]})  [unwired: 1 in]
    n90 = Send Notification(notification=w131, notifier=w134) -> (notifier out=w130:refnum<notifier>)  [unwired: 1 in, 1 out]
    n91 = local read "Auto gain ch2"() -> (w127:bool)
    n92 = Send Notification(notification=w162, notifier=w161) -> (notifier out=w158:refnum<notifier>, error out=w160:errorcluster)  [unwired: 1 in]
    n93 = case shown="True" w127 {
      tunnel: [w200 w202] -> w115
      tunnel: w123 -> [_ w207]
      tunnel: "V target(1.5)" -> [_ w206]
      frame False {
        n94 = call "V2FGV.vi"("action(write)"=enum16{"write", "read"}."read" ("action")) -> ("V2 out"=w200:dbl)  [unwired: 9 in, 1 out]
      }
      frame True {
        n95 = call "V2FGV.vi"("action(write)"=enum16{"write", "read"}."read" ("action")) -> ("V2 out"=w204:dbl)  [unwired: 9 in, 1 out]
        n96 = call "CalculateBias.vi"("GainV Last"=w207, "Sig Current(V)"=w206, "GainV current"=w204) -> ("V new"=w202:dbl)  [unwired: 8 in]
        n97 = local write "Gain 2"(w202) -> ()
        n98 = call "V2FGV.vi"("action(write)"=enum16{"write", "read"}."write" ("action"), "V2 in"=w202) -> ()  [unwired: 8 in, 2 out]
      }
    }
    n99 = Not Equal?(x=w115, y=w122) -> (x != y?=w120:bool)
    n100 = case shown="True" w120 {
      tunnel: w151 -> [w176 w183]
      tunnel: [w176 w182] -> w150
      tunnel: w148 -> [w177 w181]
      tunnel: [w177 w180] -> w147
      tunnel: w115 -> [_ w178]
      frame False {
      }
      frame True {
        n101 = global read "GlobalVariables.vi" "Ch2 LJ pin"() -> (w179:string)
        n102 = call "LJM_eWriteName.vi"("Handle In"=w181, "Name"=w179, "Value"=w178, "error in"=w183) -> ("Handle Out"=w180:i32, "error out"=w182:errorcluster)  [unwired: 10 in]
      }
    }
    n103 = local read "Auto gain ch3"() -> (w126:bool)
    n104 = case shown="True" w126 {
      tunnel: w119 -> [_ w198]
      tunnel: "V target(1.5)" -> [_ w197]
      tunnel: [w192 w194] -> w116
      frame False {
        n105 = call "V3FGV.vi"("action(write)"=enum16{"write", "read"}."read" ("action")) -> ("V3 out"=w192:dbl)  [unwired: 9 in, 1 out]
      }
      frame True {
        n106 = call "V3FGV.vi"("action(write)"=enum16{"write", "read"}."read" ("action")) -> ("V3 out"=w196:dbl)  [unwired: 9 in, 1 out]
        n107 = call "CalculateBias.vi"("GainV Last"=w198, "Sig Current(V)"=w197, "GainV current"=w196) -> ("V new"=w194:dbl)  [unwired: 8 in]
        n108 = local write "Gain 3"(w194) -> ()
        n109 = call "V3FGV.vi"("action(write)"=enum16{"write", "read"}."write" ("action"), "V3 in"=w194) -> ()  [unwired: 8 in, 2 out]
      }
    }
    n110 = Not Equal?(x=w116, y=w118) -> (x != y?=w117:bool)
    n111 = case shown="True" w117 {
      tunnel: w150 -> [w170 w175]
      tunnel: [w170 w174] -> w149
      tunnel: w147 -> [_ w173]
      tunnel: w116 -> [_ w171]
      frame False {
      }
      frame True {
        n112 = global read "GlobalVariables.vi" "Ch3 LJ pin"() -> (w172:string)
        n113 = call "LJM_eWriteName.vi"("Handle In"=w173, "Name"=w172, "Value"=w171, "error in"=w175) -> ("error out"=w174:errorcluster)  [unwired: 10 in, 1 out]
      }
    }
    n114 = Merge Errors(w149, w160) -> (w129:errorcluster)
    "processing Error Out" <- w129
    "processing loop" <- w133
  }
  n115 = while "JKI State Machine 2018" {
    shift-right: [w279] -> _
    shift-left: _ -> [w278]
    shift-right: [w281] -> _
    shift-left: w33 -> [w276]
    shift-right: [w280] -> _
    shift-left: w49 -> [w282]
    tunnel: w43 -> [w275]
    tunnel: w19 -> [w274]
    tunnel: w30 -> [w273]
    tunnel: w18 -> [w272]
    tunnel: [w271] -> w17
    tunnel: w3 -> [w267]
    stop <- w270 stop-if-true
    # "Template Copyright © 2018 JKI - http://jki.net/state-machine"
    # "Main Control Loop"
    n116 = call <vilib>:"Parse State Queue__JKI_lib_State_Machine.vi"("State Queue"=w282, "Error In (no error)"=w276) -> ("Remaining States"=w284:string, "Current State"=w266:string, "Arguments"=w283:string)  [unwired: 11 in]
    n117 = case shown="\"Data: irfAlignment\"" w266 {
      selector: w266 -> [_ _ _ _ _ _ _ _ _ _ _ _ _ _ _ _ _ w954 _ _ _ _ _ _ _ _ _ _ _ _ _ _ _ _ _ _ _ _ _ _ _ _ _ _ _ _ _ _ _ _ _ _ _ _ _ _ _ _ _ _ _ _ _ _ _ _ _ _ _ _ _ _ _ _ _ _ _ _ _ _ _ _ _ _ _ _ _ _ _ _ _ _ _ _ _ _ _ _ _ _ _ _ _ _ _ _ _ _ _ _ _ _ _ _ _ _ _ _ _ _ _ _ _ _ _ _ _ _ _ _ _ _ _ _ _ _ _ _ _ _ _ _ _ _ _ _ _ _ _ _]
      tunnel: w284 -> [w294 w570 w603 w609 w635 w661 w685 w708 w724 w759 w787 w822 w827 w896 w938 w947 w952 w958 w983 w991 w1014 w1019 w1028 w1034 w1057 w1072 w1084 w1093 w1115 w1124 w1146 w1153 w1167 w1187 w1210 w1236 w1274 w1279 w1285 w1311 w1337 w1363 w1368 w1373 w1390 w1439 w1461 w1477 w1489 w1505 w1510 w1522 w1564 w1575 w1613 w1624 w1630 w1641 w1653 w1684 w1715 w1728 w1741 w1755 w1769 w1774 w1783 w1790 w1798 w1823 w1838 w1853 w1868 w1873 w1878 w1887 w1899 w1904 w1912 w1920 w1928 w1936 w1941 w1950 w1967 w1983 w2003 w2024 w2032 w2037 w2045 w2053 w2058 w2084 w2117 w2157 w2173 w2187 w2199 w2209 w2222 w2242 w2252 w2268 w2278 w2288 w2302 w2312 w2322 w2332 w2342 w2352 w2357 w2364 w2371 w2381 w2399 w2417 w2425 w2432 w2440 w2445 w2452 w2458 w2464 w2472 w2485 w2492 w2504 w2574 w2585 w2606 w2614 w2620 w2626 w2641 w2686 w2694 w2700 w2705 w2711 w2716 w2726 w2734 w2742 w2747 w2752 w2757 w2770 w2783]
      tunnel: w283 -> [_ _ _ _ _ _ _ _ _ _ _ _ _ _ _ _ _ _ _ _ _ _ _ _ _ _ _ _ _ w1121 _ _ _ _ _ _ _ _ _ _ _ _ _ _ _ _ _ _ _ _ _ _ _ _ _ _ _ _ w1651 _ _ _ _ _ _ _ _ _ w1791 _ _ _ _ _ _ _ _ _ _ _ _ _ _ _ _ _ _ _ _ _ _ _ _ _ _ _ _ _ _ _ _ _ _ _ _ _ _ _ _ _ _ _ _ _ _ w2372 _ _ _ _ _ _ _ _ _ _ _ w2487 w2498 _ _ _ w2610 _ _ _ _ _ _ _ _ _ w2721 _ _ _ _ _ _ _]
      tunnel: w278 -> [w292 w567 _ w606 w627 w651 w676 w700 w720 w756 w777 w819 w824 w854 w935 w942 w949 w956 w976 w988 w1012 w1016 w1024 w1031 w1054 w1069 w1074 w1087 w1113 w1122 w1133 w1150 w1155 w1174 w1199 w1228 w1270 w1276 w1282 w1289 w1316 w1341 w1365 w1370 w1383 w1429 w1458 w1462 w1486 w1502 w1507 w1511 w1553 w1568 w1592 w1622 w1627 w1634 w1649 w1667 w1698 w1723 w1736 w1747 w1760 w1771 w1778 w1784 w1795 w1811 w1826 w1842 w1857 w1870 w1875 w1885 w1897 w1901 w1906 w1913 w1923 w1931 w1938 w1947 w1952 w1970 w1998 w2006 w2029 w2034 w2038 w2046 w2055 w2064 w2115 w2153 w2163 w2185 w2197 w2207 w2220 w2238 w2244 w2264 w2276 w2286 w2300 w2310 w2320 w2330 w2340 w2350 w2354 w2361 w2368 w2378 w2397 w2414 w2422 w2429 w2437 w2442 w2450 w2456 w2461 w2470 w2482 w2490 w2500 w2571 w2582 w2590 w2611 w2617 w2623 w2634 w2682 w2691 w2697 w2702 w2708 w2713 w2723 w2731 w2739 w2744 w2749 w2754 w2767 w2780]
      tunnel: [w291 w568 w601 w607 w624 w659 w674 w697 w722 w737 w764 w800 w825 w889 w904 w943 w950 w960 w980 errorcluster {"status"=FALSE, "code"=0, "source"=""} ("error out") w1011 w1017 w1026 w1032 w1055 w1070 w1078 w1090 w1105 w1118 w1134 w1151 w1165 w1185 w1208 w1227 w1272 w1277 w1283 w1290 w1317 w1342 w1366 w1371 w1380 w1421 w1452 w1466 w1487 w1493 w1508 w1514 w1544 w1566 w1580 w1616 w1628 w1639 w1643 w1658 w1689 w1718 w1731 w1746 w1759 w1772 w1776 w1786 w1793 w1813 w1828 w1843 w1858 w1871 w1876 w1879 w1894 w1902 w1910 w1918 w1926 w1934 w1939 w1943 w1955 w1978 w1997 w2018 w2027 w2035 w2043 w2051 w2056 w2066 w2112 w2155 w2161 w2175 w2191 w2201 w2210 w2240 w2243 w2258 w2270 w2281 w2293 w2304 w2315 w2324 w2334 w2344 w2355 w2362 w2369 w2379 w2396 w2415 w2423 w2430 w2438 w2443 w2448 w2455 w2462 w2468 w2483 w2488 w2501 w2572 w2581 w2592 w2612 w2618 w2624 w2630 w2676 w2692 w2698 w2703 w2709 w2714 w2724 w2732 w2740 w2745 w2750 w2755 w2768 w2781] -> w281
      tunnel: w276 -> [w290 w568 w601 w607 w625 w659 w674 w697 w722 w725 w773 w789 w825 w889 w906 w944 w950 w959 w980 w984 w1011 w1017 w1026 w1032 w1055 w1070 w1079 w1089 w1101 w1117 w1135 w1151 w1165 w1185 w1208 w1226 w1272 w1277 w1283 w1294 w1321 w1346 w1366 w1371 w1379 w1424 w1451 w1465 w1487 w1495 w1508 w1513 w1547 w1573 w1585 w1615 w1628 w1636 w1646 w1657 w1688 w1717 w1730 w1745 w1758 w1772 w1775 w1787 w1792 w1812 w1827 w1844 w1859 w1871 w1876 w1881 w1889 w1902 w1910 w1918 w1926 w1934 w1939 w1944 w1962 w1977 w1996 w2017 w2026 w2035 w2043 w2051 w2056 w2082 w2112 w2155 w2160 w2174 w2190 w2200 w2215 w2240 w2247 w2257 w2269 w2280 w2292 w2303 w2314 w2323 w2333 w2343 w2355 w2362 w2369 w2379 w2396 w2415 w2423 w2430 w2438 w2443 w2448 w2455 w2462 w2468 w2483 w2489 w2502 w2572 w2581 w2604 w2612 w2618 w2624 w2636 w2675 w2692 w2698 w2703 w2709 w2714 w2724 w2732 w2740 w2745 w2750 w2755 w2768 w2781]
      tunnel: [w293 w569 w602 w608 w634 w660 w684 w707 w723 w758 w786 w821 w826 w895 w937 w946 w951 w957 w982 w990 w1013 w1018 w1027 w1033 w1056 w1071 w1083 w1092 w1114 w1123 w1145 w1152 w1166 w1186 w1209 w1235 w1273 w1278 w1284 w1310 w1336 w1362 w1367 w1372 w1389 w1438 w1460 w1476 w1488 w1504 w1509 w1521 w1563 w1574 w1612 w1623 w1629 w1640 w1652 w1683 w1714 w1727 w1740 w1754 w1768 w1773 w1782 w1789 w1797 w1822 w1837 w1852 w1867 w1872 w1877 w1886 w1898 w1903 w1911 w1919 w1927 w1935 w1940 w1949 w1966 w1982 w2002 w2023 w2031 w2036 w2044 w2052 w2057 w2083 w2116 w2156 w2172 w2186 w2198 w2208 w2221 w2241 w2251 w2267 w2277 w2287 w2301 w2311 w2321 w2331 w2341 w2351 w2356 w2363 w2370 w2380 w2398 w2416 w2424 w2431 w2439 w2444 w2451 w2457 w2463 w2471 w2484 w2491 w2503 w2573 w2584 w2605 w2613 w2619 w2625 w2640 w2685 w2693 w2699 w2704 w2710 w2715 w2725 w2733 w2741 w2746 w2751 w2756 w2769 w2782] -> w280
      tunnel: [_ _ _ _ _ _ _ _ _ _ _ _ _ _ _ _ _ _ _ _ TRUE _ _ _ _ _ _ _ _ _ _ _ _ _ _ _ _ _ _ _ _ _ _ _ _ _ _ _ _ _ _ _ _ _ _ _ _ _ _ _ _ _ _ _ _ _ _ _ _ _ _ _ _ _ _ _ _ _ _ _ _ _ _ _ _ _ _ _ _ _ _ _ _ _ _ _ _ _ _ _ _ _ _ _ _ _ _ _ _ _ _ _ _ _ _ _ _ _ _ _ _ _ _ _ _ _ _ _ _ _ _ _ _ _ _ _ _ _ _ _ _ _ _ _ _ _ _ _ _ _] -> w270
      tunnel: [w289 w567 w575 w606 w628 w651 w676 w700 w720 w756 w777 w819 w824 w854 w935 w942 w949 w956 w981 w988 w1012 w1016 w1024 w1031 w1054 w1069 w1075 w1088 w1113 w1122 w1133 w1150 w1156 w1175 w1200 w1229 w1271 w1276 w1282 w1289 w1316 w1341 w1365 w1370 w1383 w1430 w1458 w1463 w1486 w1503 w1507 w1512 w1553 w1572 w1592 w1622 w1627 w1637 w1649 w1667 w1698 w1723 w1736 w1747 w1760 w1771 w1779 w1784 w1795 w1811 w1826 w1842 w1857 w1870 w1875 w1885 w1897 w1901 w1907 w1914 w1924 w1932 w1938 w1948 w1953 w1976 w1985 w2019 w2030 w2034 w2039 w2047 w2055 w2065 w2115 w2153 w2163 w2185 w2197 w2207 w2220 w2238 w2245 w2264 w2276 w2286 w2300 w2310 w2320 w2330 w2340 w2350 w2354 w2361 w2368 w2378 w2397 w2414 w2422 w2429 w2437 w2442 w2450 w2456 w2461 w2470 w2482 w2490 w2500 w2571 w2582 w2591 w2611 w2617 w2623 w2635 w2682 w2691 w2697 w2702 w2708 w2713 w2723 w2731 w2739 w2744 w2749 w2754 w2767 w2780] -> w279
      tunnel: 10 ("Timeout") -> [w288 _ _ _ _ _ _ _ _ _ _ _ _ _ _ _ _ _ _ _ _ _ _ _ _ _ _ _ _ _ _ _ _ _ _ _ _ _ _ _ _ _ _ _ _ _ _ _ _ _ _ _ _ _ _ _ _ _ _ _ _ _ _ _ _ _ _ _ _ _ _ _ _ _ _ _ _ _ _ _ _ _ _ _ _ _ _ _ _ _ _ _ _ _ _ _ _ _ _ _ _ _ _ _ _ _ _ _ _ _ _ _ _ _ _ _ _ _ _ _ _ _ _ _ _ _ _ _ _ _ _ _ _ _ _ _ _ _ _ _ _ _ _ _ _ _ _ _ _ _]
      tunnel: w275 -> [_ _ _ _ w632 _ _ _ _ _ _ _ _ _ _ _ _ _ _ _ _ _ _ _ _ _ _ _ _ _ _ _ _ _ _ _ _ _ _ _ _ _ _ _ _ _ _ _ _ _ _ _ _ _ _ _ _ _ _ _ _ _ _ _ _ _ _ _ _ _ _ _ _ _ _ w1882 w1893 _ _ _ _ _ _ _ _ _ _ _ _ _ _ _ _ _ _ _ _ _ _ _ _ _ _ _ _ _ _ _ _ _ _ _ _ _ _ _ _ _ _ _ _ _ _ _ _ _ _ _ _ _ _ _ _ _ _ _ _ _ _ _ _ _ _ _ _ _ _ _ _ _]
      tunnel: w274 -> [_ _ _ _ w631 _ _ _ _ _ _ _ _ _ _ _ _ _ _ _ _ _ _ _ _ _ _ _ _ _ _ _ _ _ _ _ _ _ _ _ _ _ _ _ _ _ _ _ _ _ _ _ _ _ _ _ _ _ _ _ _ _ _ _ _ _ _ _ _ _ _ _ _ _ _ w1883 w1892 _ _ _ _ _ _ _ _ _ _ _ _ _ _ _ _ _ _ _ _ _ _ _ _ _ _ _ _ _ _ _ _ _ _ _ _ _ _ _ _ _ _ _ _ _ _ _ _ _ _ _ _ _ _ _ _ _ _ _ _ _ _ _ _ _ _ _ _ _ _ _ _ _]
      tunnel: w273 -> [w287 _ _ _ _ _ _ _ _ _ _ _ _ _ _ _ _ _ _ _ _ _ _ _ _ _ _ _ _ _ _ _ _ _ _ _ _ _ _ _ _ _ _ _ _ _ w1454 _ _ _ _ _ _ _ _ _ _ _ _ _ _ _ _ _ _ _ _ _ _ _ _ _ _ _ _ _ _ _ _ _ _ _ _ _ _ _ _ _ _ _ _ _ _ _ _ _ _ _ _ _ _ _ _ _ _ _ _ _ _ _ _ _ _ _ _ _ _ _ _ _ _ _ _ _ _ _ _ _ _ _ _ _ _ _ _ _ _ _ _ _ _ _ _ _ _ _ _ _ _ _]
      tunnel: w272 -> [w286 w566 w586 w605 w633 w658 w683 w706 w721 w757 w785 w820 w823 w894 w936 w941 w948 w953 w968 w987 w1010 w1015 w1025 w1030 w1046 w1068 w1073 w1085 w1100 w1116 w1144 w1149 w1164 w1184 w1207 w1225 w1269 w1275 w1281 w1288 w1315 w1340 w1364 w1369 w1374 w1401 w1459 w1475 w1485 w1490 w1506 w1520 w1562 w1565 w1611 w1614 w1626 w1633 w1642 w1654 w1685 w1716 w1729 w1744 w1757 w1770 w1781 w1788 w1796 w1821 w1836 w1839 w1854 w1869 w1874 w1884 w1891 w1900 w1909 w1917 w1921 w1929 w1937 w1942 w1951 w1971 w1986 w2007 w2025 w2033 w2041 w2049 w2054 w2062 w2114 w2154 w2171 w2184 w2196 w2206 w2219 w2239 w2246 w2266 w2275 w2285 w2299 w2309 w2319 w2329 w2339 w2349 w2353 w2360 w2367 w2377 w2395 w2413 w2421 w2428 w2433 w2441 w2447 w2454 w2460 w2466 w2477 w2486 w2497 w2570 w2583 w2594 w2607 w2615 w2621 w2633 w2684 w2689 w2695 w2701 w2707 w2712 w2722 w2730 w2738 w2743 w2748 w2753 w2766 w2779]
      tunnel: [w285 w566 w586 w605 w633 w658 w683 w706 w721 w757 w785 w820 w823 w894 w936 w941 w948 w953 w968 w987 w1010 w1015 w1025 w1030 w1046 w1068 w1073 w1085 w1100 w1116 w1144 w1149 w1164 w1184 w1207 w1225 w1269 w1275 w1281 w1288 w1315 w1340 w1364 w1369 w1374 w1401 w1459 w1475 w1485 w1490 w1506 w1520 w1562 w1565 w1611 w1614 w1626 w1633 w1642 w1654 w1685 w1716 w1729 w1744 w1757 w1770 w1781 w1788 w1796 w1821 w1836 w1839 w1854 w1869 w1874 w1884 w1891 w1900 w1909 w1917 w1921 w1929 w1937 w1942 w1951 w1971 w1986 w2007 w2025 w2033 w2041 w2049 w2054 w2062 w2114 w2154 w2171 w2184 w2196 w2206 w2219 w2239 w2246 w2266 w2275 w2285 w2299 w2309 w2319 w2329 w2339 w2349 w2353 w2360 w2367 w2377 w2395 w2413 w2421 w2428 w2433 w2441 w2447 w2454 w2460 w2466 w2477 w2486 w2497 w2570 w2583 w2594 w2607 w2615 w2621 w2633 w2684 w2689 w2695 w2701 w2707 w2712 w2722 w2730 w2738 w2743 w2748 w2753 w2766 w2779] -> w271
      tunnel: w267 -> [_ _ _ _ w626 _ _ _ _ _ _ _ _ _ _ _ _ _ _ _ _ _ _ _ _ _ _ _ _ _ _ _ _ _ _ _ _ _ _ _ _ _ _ _ _ _ _ _ _ _ _ _ _ _ _ _ _ _ _ _ _ _ _ _ _ _ _ _ _ _ _ _ _ _ _ _ w1890 _ _ _ _ _ _ _ _ _ _ _ _ _ _ _ _ _ _ _ _ _ _ _ _ _ _ _ _ _ _ _ _ _ _ _ _ _ _ _ _ _ _ _ _ _ _ _ _ _ _ _ _ _ _ _ _ _ _ _ _ _ _ _ _ _ _ _ _ _ _ _ _ _]
      frame "", "Event Structure", "Idle" {
        # "executes when the state queue is empty"
        n118 = event shown="[13] \"Cali&iRF alignment\": Value Change" {
          selector: w286 -> [_ _ _ _ _ _ _ _ _ _ _ _ _ _ _ _ _ _ _ _ _ _ _ _ _ _ _ _ _ _ _]
          dyn-events: [_ _ _ _ _ _ _ _ _ _ _ _ _ _ _ _ _ _ _ _ _ _ _ _ _ _ _ _ _ _ _] -> w285
          timeout: w288 -> [_ _ _ _ _ _ _ _ _ _ _ _ _ _ _ _ _ _ _ _ _ _ _ _ _ _ _ _ _ _ _]
          tunnel: w294 -> [w298 w304 w320 w323 w332 w338 w346 w356 w363 w385 w399 w413 w417 w424 w437 w442 w447 w452 w455 w461 w471 w478 w486 w502 w514 w521 w525 w529 w536 w544 w560]
          tunnel: [w298 w303 w320 w322 w332 w338 w346 w356 w362 w385 w399 w413 w417 w423 w437 w442 w447 w451 w454 w461 w472 w478 w487 w502 w515 w521 w525 w528 w537 w543 w561] -> w293
          tunnel: w292 -> [w296 w307 w318 w325 w331 w339 w347 w354 w358 w383 w397 w411 w415 w419 w435 w440 w445 w448 w456 w459 w467 w476 w479 w500 w509 w519 w523 w530 w535 w541 w558]
          tunnel: [w297 w300 w319 w326 w330 w337 w345 w355 w364 w384 w398 w412 w416 w425 w436 w441 w446 w450 w457 w460 w468 w477 w485 w501 w510 w520 w524 w531 w538 w542 w559] -> w291
          tunnel: w290 -> [w297 w305 w319 w326 w330 w337 w345 w355 w364 w384 w398 w412 w416 w425 w436 w441 w446 w450 w457 w460 w468 w477 w485 w501 w513 w520 w524 w531 w538 w542 w559]
          tunnel: [w296 w307 w318 w325 w331 w339 w347 w354 w359 w383 w397 w411 w415 w420 w435 w440 w445 w448 w456 w459 w469 w476 w480 w500 w516 w519 w523 w530 w535 w541 w558] -> w289
          tunnel: w287 -> [_ _ _ _ _ _ _ _ _ _ _ _ _ _ _ _ _ _ _ _ _ _ _ _ _ _ _ _ _ _ _]
          event "355nm Laser toggle": Mouse Enter {
            n119 = event-data() -> ()  [unwired: 1 in, 4 out]
            n120 = local write "Help"("Toggle 355nm laser." ("Help")) -> ()
          }
          event "355nm Laser toggle": Value Change {
            n121 = event-data() -> ("NewVal"=w306:bool)  [unwired: 1 in, 5 out]
            n122 = Unbundle By Name(w307) -> ("LJ Pinout.355 PWM"=w311:string)
            n123 = call "LabJack_FGV.vi"("Operation(Read)"=enum16{"Write", "Read"}."Read" ("Operation"), "error in (no error)"=w305) -> ("error out"=w312:errorcluster, "Read data"=w313:i32)  [unwired: 8 in]
            n124 = case shown="False" w306 {
              tunnel: [0.0 ("Value") 1.0 ("Value")] -> w309
              frame False {
              }
              frame True {
              }
            }
            n125 = Concatenate Strings(w311, "_EF_ENABLE" ("string")) -> (w308:string)
            n126 = call "LJM_eWriteName.vi"("Handle In"=w313, "Name"=w308, "Value"=w309, "error in"=w312) -> ("error out"=w301:errorcluster)  [unwired: 10 in, 1 out]
            n127 = call <vilib>:"Add State(s) to Queue__JKI_lib_State_Machine.vi"("State(s) in Front (\"\")"="355 Laser: CheckControllerStatus\n355 Laser: CheckPWMStatus" ("State(s) in Front (\"\")"), "State(s) in (\"\")"=w304) -> ("States Out"=w303:string)  [unwired: 13 in]
            n128 = call <userlib>:"Wait (ms)__ogtk.vi"("error in (no error)"=w301, "milliseconds to wait"=u32 500) -> ("error out"=w300:errorcluster)  [unwired: 8 in, 1 out]
          }
          event "Aiming beam toggle": Mouse Enter {
            n129 = event-data() -> ()  [unwired: 1 in, 4 out]
            n130 = local write "Help"("Toggle aiming beam laser." ("Help")) -> ()
          }
          event "Aiming beam toggle": Value Change {
            n131 = event-data() -> ("NewVal"=w324:bool)  [unwired: 1 in, 5 out]
            n132 = case shown="False" w324 {
              tunnel: ["LabJack: AB_PWM_Stop" ("State(s) in Front (\"\")") "LabJack: AB_PWM_Start" ("State(s) in Front (\"\")")] -> w321
              frame False {
              }
              frame True {
              }
            }
            n133 = call <vilib>:"Add State(s) to Queue__JKI_lib_State_Machine.vi"("State(s) in Front (\"\")"=w321, "State(s) in (\"\")"=w323) -> ("States Out"=w322:string)  [unwired: 13 in]
          }
          event "Auto gain ch1": Value Change {
            n134 = event-data() -> ("NewVal"=w329:bool)  [unwired: 1 in, 5 out]
            n135 = case shown="False" w329 {
              frame False {
                n136 = local read "Gain 1"() -> (w333:dbl)
                n137 = call "V1FGV.vi"("action (write)"=enum16{"write", "read"}."write" ("action"), "V1 in"=w333) -> ()  [unwired: 8 in, 2 out]
                n138 = property on="Gain 1" class="DigNum (strict)"("DisabledEnum"=T10."Enabled" ("Disabled")) -> ()  [unwired: 2 in, 2 out]
              }
              frame True {
                n139 = property on="Gain 1" class="DigNum (strict)"("DisabledEnum"=T10."Disabled and Grayed Out" ("Disabled")) -> ()  [unwired: 2 in, 2 out]
              }
            }
          }
          event "Auto gain ch2": Value Change {
            n140 = event-data() -> ("NewVal"=w340:bool)  [unwired: 1 in, 5 out]
            n141 = case shown="False" w340 {
              frame False {
                n142 = local read "Gain 2"() -> (w341:dbl)
                n143 = property on="Gain 2" class="DigNum (strict)"("DisabledEnum"=T10."Enabled" ("Disabled")) -> ()  [unwired: 2 in, 2 out]
                n144 = call "V2FGV.vi"("action(write)"=enum16{"write", "read"}."write" ("action"), "V2 in"=w341) -> ()  [unwired: 8 in, 2 out]
              }
              frame True {
                n145 = property on="Gain 2" class="DigNum (strict)"("DisabledEnum"=T10."Disabled and Grayed Out" ("Disabled")) -> ()  [unwired: 2 in, 2 out]
              }
            }
          }
          event "Auto gain ch3": Value Change {
            n146 = event-data() -> ("NewVal"=w348:bool)  [unwired: 1 in, 5 out]
            n147 = case shown="False" w348 {
              frame False {
                n148 = local read "Gain 3"() -> (w349:dbl)
                n149 = property on="Gain 3" class="DigNum (strict)"("DisabledEnum"=T10."Enabled" ("Disabled")) -> ()  [unwired: 2 in, 2 out]
                n150 = call "V3FGV.vi"("action(write)"=enum16{"write", "read"}."write" ("action"), "V3 in"=w349) -> ()  [unwired: 8 in, 2 out]
              }
              frame True {
                n151 = property on="Gain 3" class="DigNum (strict)"("DisabledEnum"=T10."Disabled and Grayed Out" ("Disabled")) -> ()  [unwired: 2 in, 2 out]
              }
            }
          }
          event "Background": Mouse Enter {
            n152 = event-data() -> ()  [unwired: 1 in, 4 out]
            n153 = local write "Help"("Click to record a background. Currently unimplemented." ("Help")) -> ()
          }
          event "Background": Value Change {
            n154 = event-data() -> ("NewVal"=w360:bool)  [unwired: 1 in, 5 out]
            n155 = case shown="False" w360 {
              tunnel: ["UI: Cursor Set >> Busy\nUtility: SetAllChanManualGain\nQueue: Flash\nUtility: Dewelling >> 2500\nUtility: SetAllChanAutoGain\nUI: Cursor Set >> Idle\nUI: Update\nUI: WFAutoScale >> F\nLabJack: ZeroV\nLabJack: 355_PWM_Stop\nLabJack: AB_PWM_Stop\nUtility: Dewelling >> 10\nDigitizer: Abort\nUtility: RestoreDeConChan\nData: parseDataMacro\nData: saveBG\nRun: BGIncrement\nData: showBG\nUI: Update\nUI: ReadyForAquisition" "UI: Update\nUtility: SaveDeconChan\nLabJack: 355_PWM_Start\n/*LabJack: AB_PWM_Start\nDigitizer: Start\nLED: Red\nUI: duringBGAcquire\nUI: WFAutoScale >>T"] -> w361
              tunnel: [FALSE TRUE] -> w357
              frame False {
                n156 = property on="Background" class="Bool (strict)"("BoolText.Text"="Done!" ("Boolean Text.Text")) -> ()  [unwired: 2 in, 2 out]
              }
              frame True {
                n157 = property on="Background" class="Bool (strict)"("BoolText.Text"="Running" ("Boolean Text.Text"), "Colors [4]"=cluster{u32, u32}[] [{6618880, 6618880}, {16711680, 16711680}]) -> ()  [unwired: 2 in, 2 out]
              }
            }
            n158 = Bundle By Name(cluster=w358, "SysRunning?"=w357) -> (w359:T16)
            n159 = call <vilib>:"Add State(s) to Queue__JKI_lib_State_Machine.vi"("State(s) in Front (\"\")"=w361, "State(s) in (\"\")"=w363) -> ("States Out"=w362:string)  [unwired: 13 in]
          }
          event "Channel 1": Cursor Move {
            n160 = event-data() -> ("CursIdx"=w374:i32, "CursLoc"=w381:cluster{"X":dbl, "Y":dbl})  [unwired: 1 in, 7 out]
            n161 = Unbundle By Name(w381) -> ("X"=w379:dbl)
            n162 = property on="Channel 2" class="WFGraph (strict)"() -> ("CrsrList"=w378:T17)  [unwired: 2 in, 2 out]
            n163 = property on="Channel 3" class="WFGraph (strict)"() -> ("CrsrList"=w375:T17)  [unwired: 2 in, 2 out]
            n164 = Index Array(array=w378, index=w374) -> (element=w382:T18)
            n165 = Index Array(array=w375, index=w374) -> (element=w380:T18)
            n166 = Bundle By Name(cluster=w380, "Position.X"=w379) -> (w373:T18)
            n167 = Bundle By Name(cluster=w382, "Position.X"=w379) -> (w377:T18)
            n168 = Replace Array Subset(array=w378, new element=w377, index=w374) -> (w376:T17)
            n169 = Replace Array Subset(array=w375, new element=w373, index=w374) -> (w372:T17)
            n170 = property on="Channel 2" class="WFGraph (strict)"("CrsrList"=w376) -> ()  [unwired: 2 in, 2 out]
            n171 = property on="Channel 3" class="WFGraph (strict)"("CrsrList"=w372) -> ()  [unwired: 2 in, 2 out]
          }
          event "Channel 2": Cursor Move {
            n172 = event-data() -> ("CursIdx"=w390:i32, "CursLoc"=w396:cluster{"X":dbl, "Y":dbl})  [unwired: 1 in, 7 out]
            n173 = Unbundle By Name(w396) -> ("X"=w393:dbl)
            n174 = property on="Channel 1" class="WFGraph (strict)"() -> ("CrsrList"=w388:T17)  [unwired: 2 in, 2 out]
            n175 = property on="Channel 3" class="WFGraph (strict)"() -> ("CrsrList"=w391:T17)  [unwired: 2 in, 2 out]
            n176 = Index Array(array=w388, index=w390) -> (element=w395:T18)
            n177 = Index Array(array=w391, index=w390) -> (element=w394:T18)
            n178 = Bundle By Name(cluster=w395, "Position.X"=w393) -> (w392:T18)
            n179 = Bundle By Name(cluster=w394, "Position.X"=w393) -> (w389:T18)
            n180 = Replace Array Subset(array=w388, new element=w392, index=w390) -> (w387:T17)
            n181 = Replace Array Subset(array=w391, new element=w389, index=w390) -> (w386:T17)
            n182 = property on="Channel 1" class="WFGraph (strict)"("CrsrList"=w387) -> ()  [unwired: 2 in, 2 out]
            n183 = property on="Channel 3" class="WFGraph (strict)"("CrsrList"=w386) -> ()  [unwired: 2 in, 2 out]
          }
          event "Channel 3": Cursor Move {
            n184 = event-data() -> ("CursIdx"=w403:i32, "CursLoc"=w410:cluster{"X":dbl, "Y":dbl})  [unwired: 1 in, 7 out]
            n185 = Unbundle By Name(w410) -> ("X"=w407:dbl)
            n186 = property on="Channel 1" class="WFGraph (strict)"() -> ("CrsrList"=w406:T17)  [unwired: 2 in, 2 out]
            n187 = property on="Channel 2" class="WFGraph (strict)"() -> ("CrsrList"=w404:T17)  [unwired: 2 in, 2 out]
            n188 = Index Array(array=w406, index=w403) -> (element=w409:T18)
            n189 = Index Array(array=w404, index=w403) -> (element=w408:T18)
            n190 = Bundle By Name(cluster=w409, "Position.X"=w407) -> (w405:T18)
            n191 = Bundle By Name(cluster=w408, "Position.X"=w407) -> (w402:T18)
            n192 = Replace Array Subset(array=w406, new element=w405, index=w403) -> (w401:T17)
            n193 = Replace Array Subset(array=w404, new element=w402, index=w403) -> (w400:T17)
            n194 = property on="Channel 1" class="WFGraph (strict)"("CrsrList"=w401) -> ()  [unwired: 2 in, 2 out]
            n195 = property on="Channel 2" class="WFGraph (strict)"("CrsrList"=w400) -> ()  [unwired: 2 in, 2 out]
          }
          event "Cali&iRF alignment": Mouse Enter {
            n196 = event-data() -> ()  [unwired: 1 in, 4 out]
            n197 = local write "Help"("Click to run system intensity calibration and irf alignment" ("Help")) -> ()
          }
          event "Cali&iRF alignment": Value Change {
            n198 = event-data() -> ("NewVal"=w421:bool)  [unwired: 1 in, 5 out]
            n199 = case shown="False" w421 {
              tunnel: ["UI: Cursor Set >> Busy\nUtility: SetAllChanManualGain\nQueue: Flash\nUtility: Dewelling >> 1500\nUtility: SetAllChanAutoGain\nUI: Cursor Set >> Idle\nUI: Update\nLabJack: ZeroV\nLabJack: 355_PWM_Stop\nLabJack: AB_PWM_Stop\nUtility: Dewelling >> 10\nDigitizer: Abort\nUtility: RestoreDeConChan\nData: parseRunData\nData: irfAlignment\nUI: Update\nUI: ReadyForAquisition" "UI: Update\nUtility: SaveDeconChan\nLabJack: 355_PWM_Start\n/*LabJack: AB_PWM_Start\nDigitizer: Start\nLED: Red\nUI: duringIRFAlign"] -> w422
              tunnel: [FALSE TRUE] -> w418
              frame False {
                n200 = property on="Cali&iRF alignment" class="Bool (strict)"("BoolText.Text"="Done!" ("Boolean Text.Text")) -> ()  [unwired: 2 in, 2 out]
              }
              frame True {
                n201 = property on="Cali&iRF alignment" class="Bool (strict)"("BoolText.Text"="Running" ("Boolean Text.Text"), "Colors [4]"=cluster{u32, u32}[] [{6618880, 6618880}, {16711680, 16711680}]) -> ()  [unwired: 2 in, 2 out]
              }
            }
            n202 = Bundle By Name(cluster=w419, "SysRunning?"=w418) -> (w420:T16)
            n203 = call <vilib>:"Add State(s) to Queue__JKI_lib_State_Machine.vi"("State(s) in Front (\"\")"=w422, "State(s) in (\"\")"=w424) -> ("States Out"=w423:string)  [unwired: 13 in]
          }
          event "Gain 1": Value Change {
            n204 = event-data() -> ()  [unwired: 1 in, 6 out]
            n205 = call "V1FGV.vi"("action (write)"=enum16{"write", "read"}."write" ("action"), "V1 in"="Gain 1") -> ()  [unwired: 8 in, 2 out]
          }
          event "Gain 2": Value Change {
            n206 = event-data() -> ()  [unwired: 1 in, 6 out]
            n207 = call "V2FGV.vi"("action(write)"=enum16{"write", "read"}."write" ("action"), "V2 in"="Gain 2") -> ()  [unwired: 8 in, 2 out]
          }
          event "Gain 3": Value Change {
            n208 = event-data() -> ()  [unwired: 1 in, 6 out]
            n209 = call "V3FGV.vi"("action(write)"=enum16{"write", "read"}."write" ("action"), "V3 in"="Gain 3") -> ()  [unwired: 8 in, 2 out]
          }
          event "Quit": Value Change {
            # "Exit Button Value Change (pressed) Event\n(when pressed.  quite)"
            n210 = event-data() -> ()  [unwired: 1 in, 1 out]
            n211 = call <vilib>:"Add State(s) to Queue__JKI_lib_State_Machine.vi"("State(s) in Front (\"\")"="LED: Off\nMacro: Exit", "State(s) in (\"\")"=w452) -> ("States Out"=w451:string)  [unwired: 13 in]
          }
          event "Show BG": Value Change {
            n212 = event-data() -> ()  [unwired: 1 in, 6 out]
            n213 = call <vilib>:"Add State(s) to Queue__JKI_lib_State_Machine.vi"("State(s) in Front (\"\")"="Data: showBG" ("State(s) in Front (\"\")"), "State(s) in (\"\")"=w455) -> ("States Out"=w454:string)  [unwired: 13 in]
          }
          event "StartButton": Mouse Enter {
            n214 = event-data() -> ()  [unwired: 1 in, 4 out]
            n215 = local write "Help"("Press to start aquisition." ("Help")) -> ()
          }
          event "StartButton": Value Change {
            # "start PWM before acquisition"
            # "Initialize both digitizer aquisition and\n send user event to trigger aquisition loop"
            n216 = event-data() -> ()  [unwired: 1 in, 6 out]
            n217 = Unbundle By Name(w467) -> ("System Status.TCP/IP"=w466:bool)
            n218 = case shown="True" w466 {
              tunnel: ["" "TCP: sendRunNum\nTCP: sendVideoSource\nTCP: startRun"] -> w464
              frame False {
              }
              frame True {
              }
            }
            n219 = local write "StartButton"(FALSE ("StartButton")) -> ()
            n220 = Bundle By Name(cluster=w467, "SysRunning?"=TRUE) -> (w469:T16)
            n221 = call <vilib>:"Add State(s) to Queue__JKI_lib_State_Machine.vi"("State(s) in Front (\"\")"="UI: Update\nLabJack: 355_PWM_Start\nLabJack: AB_PWM_Start\nDigitizer: Start\nUI: DuringAquisition\nLED: Red", "State(s) in (\"\")"=w464) -> ("States Out"=w463:string)  [unwired: 13 in]
            n222 = call <vilib>:"Add State(s) to Queue__JKI_lib_State_Machine.vi"("State(s) in Front (\"\")"=w463, "State(s) in (\"\")"=w471) -> ("States Out"=w472:string)  [unwired: 13 in]
          }
          event "StopButton": Mouse Enter {
            n223 = event-data() -> ()  [unwired: 1 in, 4 out]
            n224 = local write "Help"("Press to stop data aquisition." ("Help")) -> ()
          }
          event "StopButton": Value Change {
            # "if system is running, send stop command, if not do nothing."
            # "stop aquisition\nupdate UI"
            n225 = event-data() -> ()  [unwired: 1 in, 6 out]
            n226 = Unbundle By Name(w479) -> ("SysRunning?"=w481:bool, "System Status.TCP/IP"=w484:bool)
            n227 = case shown="True" w481 {
              tunnel: w484 -> [_ w496]
              tunnel: ["" w495] -> w483
              tunnel: w479 -> [w488 w492]
              tunnel: [w488 w491] -> w480
              frame False {
              }
              frame True {
                n228 = case shown="True" w496 {
                  tunnel: ["" "TCP: stopRun"] -> w494
                  frame False {
                  }
                  frame True {
                  }
                }
                n229 = Bundle By Name(cluster=w492, "SysRunning?"=FALSE) -> (w491:T16)
                n230 = call <vilib>:"Add State(s) to Queue__JKI_lib_State_Machine.vi"("State(s) in Front (\"\")"=w494, "State(s) in (\"\")"="UI: Cursor Set >> Busy\nUI: Update\nUI: ReadyForAquisition\nLabJack: 355_PWM_Stop\nLabJack: AB_PWM_Stop\nDigitizer: Abort\nData: parseDataMacro\nData: saveRunData\nUI: Cursor Set>>Idle") -> ("States Out"=w495:string)  [unwired: 13 in]
              }
            }
            n231 = local write "StopButton"(FALSE ("StopButton")) -> ()
            n232 = call <vilib>:"Add State(s) to Queue__JKI_lib_State_Machine.vi"("State(s) in Front (\"\")"=w483, "State(s) in (\"\")"=w486) -> ("States Out"=w487:string)  [unwired: 13 in]
          }
          event "Sys Reconfig": Mouse Enter {
            n233 = event-data() -> ()  [unwired: 1 in, 4 out]
            n234 = local write "Help"("Click to reconfig digitizer settings." ("Help")) -> ()
          }
          event "Sys Reconfig": Value Change {
            # "everytime the user change data aquisition setting, need to reinitilize decon engine and realign iRF.\ncheck whether data length has changed, if changed, reinitialize Decon engine\nreset BG ready, need a new BG"
            # "update DAQ FGV"
            n235 = event-data() -> ()  [unwired: 1 in, 6 out]
            n236 = call "SystemConfigEditorV6.vi"("error in"=w513) -> ("error out"=w511:errorcluster, "FLImDAQ out"=w506:T5)  [unwired: 1 in]
            n237 = Unbundle By Name(w509) -> ("FLImDAQ.min record length"=w508:i32)
            n238 = Unbundle By Name(w506) -> ("min record length"=w507:i32)
            n239 = call "FLImDAQ_FGV.vi"(6:enum16{"Write", "Read"}."Write" ("Operation"), "error in (no error)"=w511, "Write data"=w506) -> ("error out"=w510:errorcluster, "Read data"=w505:T5)  [unwired: 7 in]
            n240 = Equal?(x=w508, y=w507) -> (x = y?=w504:bool)
            n241 = case shown="False" w504 {
              tunnel: ["UI: Cursor Set >> Busy\nDigitizer: Config\nDeconEngine: InitializeCh1\nDeconEngine: InitializeCh2\nDeconEngine: InitializeCh3\nUI: CaliAndiRFNotReady\n/*UI iRF not ready\nUI: Update\nUI: Cursor Set >> Idle" "UI: Cursor Set >> Busy\nDigitizer: Config\nUI: Update\nUI: Cursor Set >> Idle"] -> w503
              frame False {
              }
              frame True {
              }
            }
            n242 = Bundle By Name(cluster=w509, "FLImDAQ"=w505) -> (w516:T16)
            n243 = call <vilib>:"Add State(s) to Queue__JKI_lib_State_Machine.vi"("State(s) in Front (\"\")"=w503, "State(s) in (\"\")"=w514) -> ("States Out"=w515:string)  [unwired: 13 in]
          }
          event "System Hardware Connection Status", "StartButton", "StopButton", "355nm Laser toggle", "Aiming beam toggle", "Cali&iRF alignment", "Background", "Sys Reconfig": Mouse Leave {
            n244 = event-data() -> ()  [unwired: 1 in, 4 out]
            n245 = invoke on="Help" class="Str" method="Reinit To Default"() -> ()  [unwired: 3 in, 3 out]
          }
          event "System Hardware Connection Status.Digitizer": Mouse Enter {
            n246 = event-data() -> ()  [unwired: 1 in, 4 out]
            n247 = local write "Help"("Status of hardware connections. TCP/IP is optional." ("Help")) -> ()
          }
          event "TCP Connect": Value Change {
            n248 = event-data() -> ("NewVal"=w526:bool)  [unwired: 1 in, 5 out]
            n249 = case shown="False" w526 {
              tunnel: ["TCP: Close\nUI: Update" ("State(s) in Front (\"\")") "TCP: Initialize\nTCP: SendSettingMacro\nUI: Update" ("State(s) in Front (\"\")")] -> w527
              frame False {
              }
              frame True {
              }
            }
            n250 = call <vilib>:"Add State(s) to Queue__JKI_lib_State_Machine.vi"("State(s) in Front (\"\")"=w527, "State(s) in (\"\")"=w529) -> ("States Out"=w528:string)  [unwired: 13 in]
          }
          event User Event {
            # "if aquisition loop is error out. Stop digitizer, update front panel indicator, stop both laser and parse and save data"
            n251 = event-data() -> ()  [unwired: 1 in, 5 out]
            n252 = property on="StopButton" class="Bool (strict)"("Val(Sgnl)"=TRUE ("Value (Signaling)")) -> ()  [unwired: 2 in, 2 out]
            n253 = call <vilib>:"Add State(s) to Queue__JKI_lib_State_Machine.vi"("State(s) in (\"\")"=w536) -> ("States Out"=w537:string)  [unwired: 14 in]
          }
          event Panel Close? {
            # "Discard the event because we'll close the front panel ourselves in Macro: Exit"
            # "Close Panel button (pressed) Event\n(this executes Macro: Exit to terminate the VI)"
            n254 = event-data() -> ()  [unwired: 1 in, 1 out]
            n255 = event-data("Discard?"=TRUE) -> ()  [unwired: 1 in, 1 out]
            n256 = call <vilib>:"Add State(s) to Queue__JKI_lib_State_Machine.vi"("State(s) in Front (\"\")"="Macro: Exit", "State(s) in (\"\")"=w544) -> ("States Out"=w543:string)  [unwired: 13 in]
          }
          event Timeout {
            # "check system status every 2s"
            n257 = event-data() -> ()  [unwired: 1 in, 1 out]
            n258 = Unbundle By Name(w558) -> ("SlowTimer"=w557:u32, "FastTimer"=w545:u32)
            n259 = Tick Count (ms)() -> (millisecond timer value=w546:u32)
            n260 = Subtract(x=w546, y=w557) -> (x-y=w551:u32)
            n261 = Subtract(x=w546, y=w545) -> (x-y=w547:u32)
            n262 = Greater?(x=w551, y=u32 2000) -> (0:w552:bool)
            n263 = Greater?(x=w547, y=u32 100) -> (0:w549:bool)
            n264 = case shown="True" w552 {
              tunnel: ["" "SystemStatus: SlowSysStatusMacro" ("State(s) in Front (\"\")")] -> w553
              frame False {
              }
              frame True {
              }
            }
            n265 = case shown="True" w549 {
              tunnel: ["" "SystemStatus: FastSysStatusMacro" ("State(s) in Front (\"\")")] -> w548
              frame False {
              }
              frame True {
              }
            }
            n266 = call <vilib>:"Add State(s) to Queue__JKI_lib_State_Machine.vi"("State(s) in Front (\"\")"="LabJack: checkPedal" ("State(s) in Front (\"\")"), "State(s) in (\"\")"=w553, "State(s) at Back (\"\")"=w548) -> ("States Out"=w555:string)  [unwired: 12 in]
            n267 = call <vilib>:"Add State(s) to Queue__JKI_lib_State_Machine.vi"("State(s) in Front (\"\")"=w555, "State(s) in (\"\")"=w560) -> ("States Out"=w561:string)  [unwired: 13 in]
          }
        }
      }
      frame "---------- Data ----------" {
        # "Do not put any code in this frame.\n(It is a separator no-op. You can make a copy of this frame to create a new Data frame)"
        n268 = call <vilib>:"Add State(s) to Queue__JKI_lib_State_Machine.vi"("State(s) in (\"\")"=w570) -> ("States Out"=w569:string)  [unwired: 14 in]
      }
      frame "Data: Initialize" {
        w571 = cluster{"RunID":i8, "BG ID":i8, "Cali ID":i8} {"RunID"=1, "BG ID"=1, "Cali ID"=1}  # IDs
        w572 = refnum<vi> refnum  # LED vi reference
        w573 = path ""  # TempPath
        w574 = T19 {"DataPath"=path "", "BG Path"=path "", "iRFPath"=path "", "CaliPath"=path ""}  # Pathes
        w576 = dbl[] []  # V3
        w577 = dbl[] []  # V2
        w578 = dbl[] []  # V1
        w580 = u32 0  # FastTimer
        w581 = u32 0  # SlowTimer
        w582 = dbl[][] []  # Ch3Data
        w583 = dbl[][] []  # Ch2Data
        w584 = dbl[][] []  # Ch1Data
        w587 = T1 {"Digitizer"=FALSE, "Labjack"=FALSE, "Aiming Beam"=FALSE, "355 Laser"=FALSE, "TCP/IP"=FALSE}  # System Status
        w588 = T20 {"DIO_EF_CLOCK1_DIVISOR"=16, "DIO_EF_CLOCK1_ROLL_VALUE"=25000, "DIO#_EF_INDEX"=0, "DIO#_EF_OPTIONS"=1, "DIO#_EF_CONFIG_A"=6250}  # AB PWM setting
        w589 = T4 {"Ch1 Bias"="TDA11", "Ch2 Bias"="DAC10", "Ch3 Bias"="DAC0", "Ch4 Bias"="DAC0", "355 PWM"="FIO0", "AimingBeam PWM"="FIO2", "Laser Ready"="FIO3", "Interlock"="FIO1", "Laser Start/Stop"="FIO1", "Red LED"="FIO1", "Green LED"="FIO1", "Foot Pedal"="DIO15"}  # LJ Pinout
        w590 = 0  # TCP attempt count
        w591 = u32 0  # Laser start tic
        w592 = refnum<k20>[] []  # niTClk sessions
        w593 = u32 0  # Last Trigger
        w594 = T20 {"DIO_EF_CLOCK1_DIVISOR"=16, "DIO_EF_CLOCK1_ROLL_VALUE"=25000, "DIO#_EF_INDEX"=0, "DIO#_EF_OPTIONS"=1, "DIO#_EF_CONFIG_A"=6250}  # 355 PWM setting
        w595 = T21 {"Aiming Beam COM Port"="COM3", "Min Current"=0.0, "Max Current"=63.0, "Default Current"=20.0, 0}  # AB Cluster
        w596 = T22 {"resource name"="", "resource name 2"="", "Channel"=enum."Channel 0", "trigger source"="VAL_EXTERNAL", "trigger level"=0.5, "trigger delay"=1.35e-07, "min sample rate"=12500000000.0, "min record length"=2500, "vertical range"=1.0, "vertical offset"=-0.25, "Waveform to Avg"=2000}  # FLImDAQ
        w597 = FALSE  # SysRunning?
        w585 = path ""  # DefaultPath
        w598 = ""  # CaseID
        w599 = T3 {"Ch1Enable?"=FALSE, "Ch2Enable?"=FALSE, "Ch3Enable?"=FALSE, "Ch1AutoGain?"=FALSE, "Ch2AutoGain?"=FALSE, "Ch3AutoGain?"=FALSE, "AimingBeamEnable?"=FALSE}  # SysConfigCluster
        w600 = T23 {"Current VI Reference"=refnum, "Close Panel on Exit?"=FALSE}  # Core
        # "Initialize the shift-register data, here.\n(data names are defined by what you wire into the bundle function)"
        n269 = Bundle("Core"=w600, "SysConfigCluster"=w599, "System Status"=w587, "IDs"=w571, "CaseID"=w598, "DefaultPath"=w585, "Pathes"=w574, "FLImDAQ"=w596, "SysRunning?"=w597, "AB Cluster"=w595, "LJ Pinout"=w589, "355 PWM setting"=w594, "AB PWM setting"=w588, "Last Trigger"=w593, "niTClk sessions"=w592, "Laser start tic"=w591, "TCP attempt count"=w590, "Ch1Data"=w584, "Ch2Data"=w583, "Ch3Data"=w582, "V1"=w578, "V2"=w577, "V3"=w576, "SlowTimer"=w581, "FastTimer"=w580, "listener ID"=refnum<k5> refnum, "TempPath"=w573, "LED vi reference"=w572) -> (w575:T16)  [unwired: 1 in]
        n270 = call <vilib>:"Add State(s) to Queue__JKI_lib_State_Machine.vi"("State(s) in (\"\")"=w603) -> ("States Out"=w602:string)  [unwired: 14 in]
      }
      frame "Data: parseDataMacro" {
        # "Sometimes it takes some time to parse run data"
        # "Parse data macro.\n(Set curse busy, parse data, then set cursor idle)"
        n271 = call <vilib>:"Add State(s) to Queue__JKI_lib_State_Machine.vi"("State(s) in Front (\"\")"="UI: Cursor Set >> Busy\nData: parseRunData\nUI: Cursor Set >> Idle" ("State(s) in Front (\"\")"), "State(s) in (\"\")"=w609) -> ("States Out"=w608:string)  [unwired: 13 in]
      }
      frame "Data: parseRunData" {
        # "flash queue"
        # "Ch3&4"
        # "Ch1&2"
        # "Flash data from queue and save it in structure\n()"
        n272 = Flush Queue(queue=w632, error in (no error)=w625) -> (remaining elements=w630:cluster{"double data":dbl[][]}[], error out=w623:errorcluster)  [unwired: 1 out]
        n273 = Flush Queue(queue=w626, error in (no error)=w625) -> (remaining elements=w620:cluster{"V1":dbl, "V2":dbl, "V3":dbl}[], error out=w621:errorcluster)  [unwired: 1 out]
        n274 = Flush Queue(queue=w631, error in (no error)=w625) -> (remaining elements=w629:cluster{"double data":dbl[][]}[], error out=w622:errorcluster)  [unwired: 1 out]
        n275 = for {
          tunnel: w629 -> [w642] mode=indexing
          tunnel: [w641] -> w610 mode=concatenating
          n276 = Unbundle By Name(w642) -> ("double data"=w640:dbl[][])
          n277 = call "SeperateChanData.vi"("Input (Ch1&2)"=w640) -> ("Ch1"=w641:dbl[][])  [unwired: 1 out]
        }
        n278 = for {
          tunnel: w620 -> [w639] mode=indexing
          tunnel: [w638] -> w615 mode=indexing
          tunnel: [w637] -> w614 mode=indexing
          tunnel: [w636] -> w613 mode=indexing
          n279 = Unbundle By Name(w639) -> ("V1"=w638:dbl, "V2"=w637:dbl, "V3"=w636:dbl)
        }
        "V1" <- w615
        "V2" <- w614
        "V3" <- w613
        n280 = for {
          tunnel: w630 -> [w646] mode=indexing
          tunnel: [w644] -> w612 mode=concatenating
          tunnel: [w643] -> w611 mode=concatenating
          n281 = Unbundle By Name(w646) -> ("double data"=w645:dbl[][])
          n282 = call "SeperateChanData.vi"("Input (Ch1&2)"=w645) -> ("Ch1"=w644:dbl[][], "Ch2"=w643:dbl[][])
        }
        n283 = Array Size(array=w615) -> (size(s)=→"V1 Size":i32)
        n284 = Array Size(array=w614) -> (size(s)=→"V2 Size":i32)
        n285 = Array Size(array=w613) -> (size(s)=→"V3 Size":i32)
        n286 = Bundle By Name(cluster=w627, "Ch1Data"=w612, "Ch2Data"=w611, "Ch3Data"=w610, "V1"=w615, "V2"=w614, "V3"=w613) -> (w628:T16)
        n287 = Array Size(array=w610) -> (size(s)=→"data Size":i32[])
        n288 = Merge Errors(w623, w622, w621) -> (w624:errorcluster)
        n289 = call <vilib>:"Add State(s) to Queue__JKI_lib_State_Machine.vi"("State(s) in (\"\")"=w635) -> ("States Out"=w634:string)  [unwired: 14 in]
      }
      frame "Data: loadLastUseiRF" {
        # "Load last use iRF.\n()"
        n290 = Unbundle By Name(w651) -> ("TempPath"=w650:path)
        n291 = Build Path(base path=w650, name or relative path="iRF.tdms") -> (appended path=w656:path)
        n292 = TDMS Open(11:w656) -> (0:w654:errorcluster, 3:w655:refnum<k34>)  [unwired: 6 in]
        n293 = TDMS Read(0:w655, 11:w654, 12:dbl[][] []) -> (4:w648:refnum<k34>, 10:w652:dbl[][], 15:w647:errorcluster)  [unwired: 5 in, 3 out]
        n294 = case shown="No Error" w647 {
          tunnel: w652 -> [w664 _]
          tunnel: ["UI: CaliAndiRFLoaded" ("State(s) in Front (\"\")") ""] -> w649
          frame No Error {
            n295 = Index Array(array=w664, index (row)=0) -> (element=w667:dbl[])  [unwired: 1 in]
            n296 = Index Array(array=w664, index (row)=1) -> (element=w666:dbl[])  [unwired: 1 in]
            n297 = Index Array(array=w664, index (row)=2) -> (element=w665:dbl[])  [unwired: 1 in]
            n298 = Bundle(w667, w666, w665) -> (w663:cluster{dbl[], dbl[], dbl[]})  [unwired: 1 in]
            n299 = global write "GlobalVariables.vi" "LastUseiRF"(w663) -> ()
          }
          frame Error {
          }
        }
        n300 = TDMS Close(8:w647, 11:w648) -> ()  [unwired: 2 out]
        n301 = call <vilib>:"Add State(s) to Queue__JKI_lib_State_Machine.vi"("State(s) in Front (\"\")"=w649, "State(s) in (\"\")"=w661) -> ("States Out"=w660:string)  [unwired: 13 in]
      }
      frame "Data: loadLastUseCali" {
        # "Load last use calibration.\n()"
        n302 = Unbundle By Name(w676) -> ("TempPath"=w675:path)
        n303 = Build Path(base path=w675, name or relative path="Calibration.tdms") -> (appended path=w681:path)
        n304 = TDMS Open(11:w681) -> (0:w679:errorcluster, 3:w680:refnum<k34>)  [unwired: 6 in]
        n305 = TDMS Read(0:w680, 11:w679, 12:dbl[][] []) -> (4:w672:refnum<k34>, 10:w677:dbl[][], 15:w673:errorcluster)  [unwired: 5 in, 3 out]
        n306 = TDMS Close(8:w673, 11:w672) -> ()  [unwired: 2 out]
        n307 = case shown="Error .." w673 {
          tunnel: w677 -> [w690 _]
          frame No Error {
            n308 = Index Array(array=w690, index (row)=0) -> (element=w689:dbl[])  [unwired: 1 in]
            n309 = Index Array(array=w690, index (row)=1) -> (element=w688:dbl[])  [unwired: 1 in]
            n310 = Index Array(array=w690, index (row)=2) -> (element=w686:dbl[])  [unwired: 1 in]
            n311 = Bundle(w689, w688, w686) -> (w687:cluster{dbl[], dbl[], dbl[]})  [unwired: 1 in]
            n312 = global write "GlobalVariables.vi" "LastUseCaliData"(w687) -> ()
          }
          frame Error {
          }
        }
        n313 = call <vilib>:"Add State(s) to Queue__JKI_lib_State_Machine.vi"("State(s) in (\"\")"=w685) -> ("States Out"=w684:string)  [unwired: 14 in]
      }
      frame "Data: loadLastUseBG" {
        # "check data size here. If not the same as current setting, return error."
        # "Load last use BG.\n()"
        n314 = Unbundle By Name(w700) -> ("TempPath"=w699:path)
        n315 = Build Path(base path=w699, name or relative path="Background.tdms") -> (appended path=w704:path)
        n316 = TDMS Open(11:w704) -> (0:w702:errorcluster, 3:w703:refnum<k34>)  [unwired: 6 in]
        n317 = TDMS Read(0:w703, 11:w702, 12:dbl[][] []) -> (4:w695:refnum<k34>, 10:w698:dbl[][], 15:w694:errorcluster)  [unwired: 5 in, 3 out]
        n318 = TDMS Close(8:w694, 11:w695) -> ()  [unwired: 2 out]
        n319 = case shown="Error .." w694 {
          tunnel: w698 -> [w710 _]
          tunnel: ["UI: BGLoaded" ("State(s) in Front (\"\")") ""] -> w696
          frame No Error {
            w711 = enum16{"write", "read"}."write" ("action")
            # "If no error, check size match"
            n320 = Index Array(array=w710, index (row)=0) -> (element=w714:dbl[])  [unwired: 1 in]
            n321 = Index Array(array=w710, index (row)=1) -> (element=w713:dbl[])  [unwired: 1 in]
            n322 = Index Array(array=w710, index (row)=2) -> (element=w712:dbl[])  [unwired: 1 in]
            n323 = call "BG3FGV.vi"("action"=w711, "BG3 in"=w712) -> ()  [unwired: 8 in, 2 out]
            n324 = call "BG1FGV.vi"("action"=w711, "BG1 in"=w714) -> ()  [unwired: 8 in, 2 out]
            n325 = call "BG2FGV.vi"("action"=w711, "BG2 in"=w713) -> ()  [unwired: 8 in, 2 out]
          }
          frame Error {
            # "If error set BG all 0, update UI"
          }
        }
        n326 = call <vilib>:"Add State(s) to Queue__JKI_lib_State_Machine.vi"("State(s) in Front (\"\")"=w696, "State(s) in (\"\")"=w708) -> ("States Out"=w707:string)  [unwired: 13 in]
      }
      frame "Data: loadLastUseMacro" {
        # "Load last use BG and Cali and iRF.\n(It is a separator no-op. You can make a copy of this frame to create a new Data frame)"
        n327 = call <vilib>:"Add State(s) to Queue__JKI_lib_State_Machine.vi"("State(s) in Front (\"\")"="Data: loadLastUseBG\nData: loadLastUseCali\nData: loadLastUseiRF" ("State(s) in Front (\"\")"), "State(s) in (\"\")"=w724) -> ("States Out"=w723:string)  [unwired: 13 in]
      }
      frame "Data: saveCalibration" {
        w736 = T11."create or replace" ("operation (0:open)")
        w741 = string[] ["Ch1", "Ch2", "Ch3"] ("channel name(s) in (Untitled)")
        w740 = "Calibration" ("group name in (Untitled)")
        w726 = "Calibration" ("default name")
        # "Average data and save calibration file\n(It is a separator no-op. You can make a copy of this frame to create a new Data frame)"
        n328 = Unbundle By Name(w756) -> ("Ch1Data"=w755:dbl[][], "Ch2Data"=w754:dbl[][], "Ch3Data"=w753:dbl[][], "Pathes.CaliPath"=w728:path, "TempPath"=w748:path, "IDs.Cali ID"=w727:i8)
        n329 = Build Path(base path=w748, name or relative path=w726) -> (appended path=w745:path)
        n330 = Format Value(string ("")=w726, format string="%02d", value (0)=w727) -> (output string=w731:string)
        n331 = call "AvgArray.vi"("2D array in"=w755) -> ("1D Avg out"=w735:dbl[])  [unwired: 10 in]
        n332 = call "AvgArray.vi"("2D array in"=w754) -> ("1D Avg out"=w734:dbl[])  [unwired: 10 in]
        n333 = call "AvgArray.vi"("2D array in"=w753) -> ("1D Avg out"=w733:dbl[])  [unwired: 10 in]
        n334 = Build Path(base path=w728, name or relative path=w731) -> (appended path=w729:path)
        n335 = TDMS Open(8:w725, 10:w736, 11:w745) -> (0:w747:errorcluster, 3:w744:refnum<k34>)  [unwired: 4 in]
        n336 = TDMS Open(8:w725, 10:w736, 11:w729) -> (0:w751:errorcluster, 3:w752:refnum<k34>)  [unwired: 4 in]
        n337 = Build Array(w735, w734, w733) -> (w742:dbl[][])
        n338 = Bundle("1D Avg out"=w735, "1D Avg out"=w734, "1D Avg out"=w733) -> (w732:T24)  [unwired: 1 in]
        n339 = TDMS Write(0:w744, 5:w740, 7:w741, 9:w742, 11:w747) -> (4:w743:refnum<k34>, 15:w746:errorcluster)  [unwired: 1 in, 2 out]
        n340 = TDMS Write(0:w752, 5:w740, 7:w741, 9:w742, 11:w751) -> (4:w750:refnum<k34>, 15:w749:errorcluster)  [unwired: 1 in, 2 out]
        n341 = global write "GlobalVariables.vi" "LastUseCaliData"(w732) -> ()
        n342 = TDMS Close(8:w746, 11:w743) -> (0:w738:errorcluster)  [unwired: 1 out]
        n343 = TDMS Close(8:w749, 11:w750) -> (0:w739:errorcluster)  [unwired: 1 out]
        n344 = Merge Errors(w739, w738) -> (w737:errorcluster)
        n345 = call <vilib>:"Add State(s) to Queue__JKI_lib_State_Machine.vi"("State(s) in (\"\")"=w759) -> ("States Out"=w758:string)  [unwired: 14 in]
      }
      frame "Data: saveiRF" {
        w784 = enum16{"write", "read"}."read" ("action")
        # "Get iRF from decon stracture and save it on disk.\n(It is a separator no-op. You can make a copy of this frame to create a new Data frame)"
        n346 = Unbundle By Name(w777) -> ("TempPath"=w776:path)
        n347 = call "Ch1DeconEngineFGV.vi"("action(read)"=w784) -> ("Error Out"=w782:errorcluster, "Ch1DeconEngine out"=w783:refnum<class "LaguerreDeconEngineClass.lvclass">)  [unwired: 9 in]
        n348 = call "Ch2DeconEngineFGV.vi"("action(read)"=w784) -> ("Error Out"=w780:errorcluster, "Ch2DeconEngine out"=w781:refnum<class "LaguerreDeconEngineClass.lvclass">)  [unwired: 9 in]
        n349 = call "Ch3DeconEngineFGV.vi"("action(read)"=w784) -> ("Error Out"=w778:errorcluster, "Ch3DeconEngine out"=w779:refnum<class "LaguerreDeconEngineClass.lvclass">)  [unwired: 9 in]
        n350 = Build Path(base path=w776, name or relative path="iRF" ("default name")) -> (appended path=w774:path)
        n351 = call "getIRF.vi"("error in (no error)"=w782, "LaguerreDeconEngineClass in"=w783) -> ("iRF"=w763:dbl[])  [unwired: 7 in, 2 out]
        n352 = call "getIRF.vi"("error in (no error)"=w780, "LaguerreDeconEngineClass in"=w781) -> ("iRF"=w762:dbl[])  [unwired: 7 in, 2 out]
        n353 = call "getIRF.vi"("error in (no error)"=w778, "LaguerreDeconEngineClass in"=w779) -> ("iRF"=w761:dbl[])  [unwired: 7 in, 2 out]
        n354 = Build Array(w763, w762, w761) -> (w769:dbl[][])
        n355 = TDMS Open(8:w773, 10:T11."create or replace" ("operation (0:open)"), 11:w774) -> (0:w770:errorcluster, 3:w771:refnum<k34>)  [unwired: 4 in]
        n356 = Bundle("iRF"=w763, "iRF"=w762, "iRF"=w761) -> (w760:cluster{"iRF":dbl[], "iRF":dbl[], "iRF":dbl[]})  [unwired: 1 in]
        n357 = global write "GlobalVariables.vi" "LastUseiRF"(w760) -> ()
        n358 = TDMS Write(0:w771, 5:"iRF" ("group name in (Untitled)"), 7:string[] ["Ch1", "Ch2", "Ch3"] ("channel name(s) in (Untitled)"), 9:w769, 11:w770) -> (4:w766:refnum<k34>, 15:w765:errorcluster)  [unwired: 1 in, 2 out]
        n359 = TDMS Close(8:w765, 11:w766) -> (0:w764:errorcluster)  [unwired: 1 out]
        n360 = call <vilib>:"Add State(s) to Queue__JKI_lib_State_Machine.vi"("State(s) in (\"\")"=w787) -> ("States Out"=w786:string)  [unwired: 14 in]
      }
      frame "Data: saveBG" {
        w793 = "Background" ("name or relative path")
        w803 = T11."create or replace" ("operation (0:open)")
        w798 = string[] ["Ch1", "Ch2", "Ch3"] ("channel name(s) in (Untitled)")
        w796 = "Background" ("group name in (Untitled)")
        w816 = enum16{"write", "read"}."write" ("action")
        # "Save BG and pass it to FGV.\n(save BG to disk and set it to FGV)"
        n361 = Unbundle By Name(w819) -> ("Ch1Data"=w818:dbl[][], "Ch2Data"=w817:dbl[][], "Ch3Data"=w815:dbl[][], "Pathes.BG Path"=w788:path, "TempPath"=w791:path, "IDs.BG ID"=w794:i8)
        n362 = Format Value(string ("")=w793, format string="%02d", value (0)=w794) -> (output string=w792:string)
        n363 = Build Path(base path=w788, name or relative path=w792) -> (appended path=w790:path)
        n364 = Build Path(base path=w791, name or relative path=w793) -> (appended path=w799:path)
        n365 = call "AvgArray.vi"("2D array in"=w818) -> ("1D Avg out"=w812:dbl[])  [unwired: 10 in]
        n366 = call "AvgArray.vi"("2D array in"=w817) -> ("1D Avg out"=w811:dbl[])  [unwired: 10 in]
        n367 = call "AvgArray.vi"("2D array in"=w815) -> ("1D Avg out"=w810:dbl[])  [unwired: 10 in]
        n368 = TDMS Open(8:w789, 10:w803, 11:w790) -> (0:w813:errorcluster, 3:w814:refnum<k34>)  [unwired: 4 in]
        n369 = call "BG1FGV.vi"("action"=w816, "BG1 in"=w812) -> ()  [unwired: 8 in, 2 out]
        n370 = call "BG2FGV.vi"("action"=w816, "BG2 in"=w811) -> ()  [unwired: 8 in, 2 out]
        n371 = call "BG3FGV.vi"("action"=w816, "BG3 in"=w810) -> ()  [unwired: 8 in, 2 out]
        n372 = TDMS Open(8:w789, 10:w803, 11:w799) -> (0:w806:errorcluster, 3:w807:refnum<k34>)  [unwired: 4 in]
        n373 = Build Array(w812, w811, w810) -> (w797:dbl[][])
        n374 = TDMS Write(0:w814, 5:w796, 7:w798, 9:w797, 11:w813) -> (4:w809:refnum<k34>, 15:w808:errorcluster)  [unwired: 1 in, 2 out]
        n375 = TDMS Write(0:w807, 5:w796, 7:w798, 9:w797, 11:w806) -> (4:w805:refnum<k34>, 15:w804:errorcluster)  [unwired: 1 in, 2 out]
        n376 = TDMS Close(8:w808, 11:w809) -> (0:w802:errorcluster)  [unwired: 1 out]
        n377 = TDMS Close(8:w804, 11:w805) -> (0:w801:errorcluster)  [unwired: 1 out]
        n378 = Merge Errors(w802, w801) -> (w800:errorcluster)
        n379 = call <vilib>:"Add State(s) to Queue__JKI_lib_State_Machine.vi"("State(s) in (\"\")"=w822) -> ("States Out"=w821:string)  [unwired: 14 in]
      }
      frame "Data: showBG" {
        # "Show BG in seperate window.\n()"
        n380 = call "showBG.vi"() -> ()  [unwired: 12 in]
        n381 = call <vilib>:"Add State(s) to Queue__JKI_lib_State_Machine.vi"("State(s) in (\"\")"=w827) -> ("States Out"=w826:string)  [unwired: 14 in]
      }
      frame "Data: irfAlignment" {
        w876 = enum16{"write", "read"}."write" ("action")
        w890 = enum16{"write", "read"}."read" ("action")
        # "do iRF alignment in this state\n(It is a separator no-op. You can make a copy of this frame to create a new Data frame)"
        n382 = Unbundle By Name(w854) -> ("Ch1Data"=w893:dbl[][], "Ch2Data"=w892:dbl[][], "Ch3Data"=w891:dbl[][])
        n383 = local read "length"() -> (w840:i32)
        n384 = local read "start Idx"() -> (w841:i32)
        n385 = call "Ch3DeconEngineFGV.vi"("Error In"=w889, "action(read)"=w890) -> ("Error Out"=w883:errorcluster, "Ch3DeconEngine out"=w884:refnum<class "LaguerreDeconEngineClass.lvclass">)  [unwired: 8 in]
        n386 = call "Ch1DeconEngineFGV.vi"("Error In"=w889, "action(read)"=w890) -> ("Error Out"=w887:errorcluster, "Ch1DeconEngine out"=w888:refnum<class "LaguerreDeconEngineClass.lvclass">)  [unwired: 8 in]
        n387 = call "Ch2DeconEngineFGV.vi"("Error In"=w889, "action(read)"=w890) -> ("Error Out"=w885:errorcluster, "Ch2DeconEngine out"=w886:refnum<class "LaguerreDeconEngineClass.lvclass">)  [unwired: 8 in]
        n388 = call "AvgArray.vi"("2D array in"=w891) -> ("1D Avg out"=w828:dbl[])  [unwired: 10 in]
        n389 = call "AvgArray.vi"("2D array in"=w892) -> ("1D Avg out"=w829:dbl[])  [unwired: 10 in]
        n390 = call "AvgArray.vi"("2D array in"=w893) -> ("1D Avg out"=w830:dbl[])  [unwired: 10 in]
        n391 = call "RemoveDCBG.vi"(8:w840, "Channel"=w841, "WF in"=w828) -> ("DC"=w833:dbl, "WF out"=w842:dbl[])  [unwired: 6 in, 1 out]
        n392 = call "RemoveDCBG.vi"(8:w840, "Channel"=w841, "WF in"=w829) -> ("DC"=w835:dbl, "WF out"=w843:dbl[])  [unwired: 6 in, 1 out]
        n393 = call "RemoveDCBG.vi"(8:w840, "Channel"=w841, "WF in"=w830) -> ("DC"=w838:dbl, "WF out"=w844:dbl[])  [unwired: 6 in, 1 out]
        n394 = call "computeIRFAlignment.vi"("error in (no error)"=w883, "fIRF temp"=w842, "LaguerreDeconEngineClass in"=w884) -> ("error out"=w881:errorcluster, "LaguerreDeconEngineClass out"=w882:refnum<class "LaguerreDeconEngineClass.lvclass">)  [unwired: 6 in, 1 out]
        n395 = call "computeIRFAlignment.vi"("error in (no error)"=w885, "fIRF temp"=w843, "LaguerreDeconEngineClass in"=w886) -> ("error out"=w877:errorcluster, "LaguerreDeconEngineClass out"=w878:refnum<class "LaguerreDeconEngineClass.lvclass">)  [unwired: 6 in, 1 out]
        n396 = call "computeIRFAlignment.vi"("error in (no error)"=w887, "fIRF temp"=w844, "LaguerreDeconEngineClass in"=w888) -> ("error out"=w879:errorcluster, "LaguerreDeconEngineClass out"=w880:refnum<class "LaguerreDeconEngineClass.lvclass">)  [unwired: 6 in, 1 out]
        n397 = call "Ch1DeconEngineFGV.vi"("Error In"=w879, "action(read)"=w876, "Ch1DeconEngine in"=w880) -> ("Error Out"=w874:errorcluster, "Ch1DeconEngine out"=w875:refnum<class "LaguerreDeconEngineClass.lvclass">)  [unwired: 7 in]
        n398 = call "Ch2DeconEngineFGV.vi"("Error In"=w877, "action(read)"=w876, "Ch2DeconEngine in"=w878) -> ("Error Out"=w864:errorcluster, "Ch2DeconEngine out"=w865:refnum<class "LaguerreDeconEngineClass.lvclass">)  [unwired: 7 in]
        n399 = call "Ch3DeconEngineFGV.vi"("Error In"=w881, "action(read)"=w876, "Ch3DeconEngine in"=w882) -> ("Error Out"=w858:errorcluster, "Ch3DeconEngine out"=w859:refnum<class "LaguerreDeconEngineClass.lvclass">)  [unwired: 7 in]
        n400 = call "setfIRF.vi"("error in (no error)"=w858, "fIRF"=w842, "LaguerreDeconEngineClass in"=w859) -> ("error out"=w862:errorcluster, "LaguerreDeconEngineClass out"=w863:refnum<class "LaguerreDeconEngineClass.lvclass">)  [unwired: 7 in]
        n401 = call "setfIRF.vi"("error in (no error)"=w864, "fIRF"=w843, "LaguerreDeconEngineClass in"=w865) -> ("error out"=w868:errorcluster, "LaguerreDeconEngineClass out"=w869:refnum<class "LaguerreDeconEngineClass.lvclass">)  [unwired: 7 in]
        n402 = call "setfIRF.vi"("error in (no error)"=w874, "fIRF"=w844, "LaguerreDeconEngineClass in"=w875) -> ("error out"=w872:errorcluster, "LaguerreDeconEngineClass out"=w873:refnum<class "LaguerreDeconEngineClass.lvclass">)  [unwired: 7 in]
        n403 = call "computeLCs.vi"("error in (no error)"=w862, "LaguerreDeconClass in"=w863) -> ("error out"=w860:errorcluster, "LaguerreDeconClass out"=w861:refnum<class "LaguerreDeconEngineClass.lvclass">)  [unwired: 8 in]
        n404 = call "computeLCs.vi"("error in (no error)"=w868, "LaguerreDeconClass in"=w869) -> ("error out"=w866:errorcluster, "LaguerreDeconClass out"=w867:refnum<class "LaguerreDeconEngineClass.lvclass">)  [unwired: 8 in]
        n405 = call "computeLCs.vi"("error in (no error)"=w872, "LaguerreDeconClass in"=w873) -> ("error out"=w870:errorcluster, "LaguerreDeconClass out"=w871:refnum<class "LaguerreDeconEngineClass.lvclass">)  [unwired: 8 in]
        n406 = Unbundle By Name(w854) -> ("V1"=w853:dbl[], "V2"=w852:dbl[], "V3"=w851:dbl[])
        n407 = call-poly <vilib>:"Mean.vi"("X"=w853) -> ("mean"=w850:dbl)  [unwired: 1 out]
        n408 = call "getFitting.vi"("error in (no error)"=w860, "LaguerreDeconEngineClass in"=w861) -> ("Fitting"=w831:dbl[])  [unwired: 7 in, 2 out]
        n409 = call "getFitting.vi"("error in (no error)"=w866, "LaguerreDeconEngineClass in"=w867) -> ("Fitting"=w834:dbl[])  [unwired: 7 in, 2 out]
        n410 = call "getFitting.vi"("error in (no error)"=w870, "LaguerreDeconEngineClass in"=w871) -> ("Fitting"=w837:dbl[])  [unwired: 7 in, 2 out]
        n411 = Add(x=w838, y=w837) -> (x+y=w839:dbl[])
        n412 = Add(x=w835, y=w834) -> (x+y=w836:dbl[])
        n413 = call-poly <vilib>:"Mean.vi"("X"=w852) -> ("mean"=w849:dbl)  [unwired: 1 out]
        n414 = Add(x=w833, y=w831) -> (x+y=w832:dbl[])
        n415 = Build Array(w830, w839) -> (w857:dbl[][])
        n416 = Build Array(w829, w836) -> (w856:dbl[][])
        n417 = call-poly <vilib>:"Mean.vi"("X"=w851) -> ("mean"=w848:dbl)  [unwired: 1 out]
        n418 = Build Array(w828, w832) -> (w855:dbl[][])
        n419 = Bundle("mean"=w850, "mean"=w849, "mean"=w848) -> (w847:cluster{"mean":dbl, "mean":dbl, "mean":dbl})  [unwired: 1 in]
        n420 = call "Calib_and_iRFAlign_confirm.vi"("Ch4 Data"=w847, "Ch3 Data"=w855, "Ch2 Data"=w856, "Ch1 Data"=w857) -> ("Save?"=w846:bool)  [unwired: 7 in]
        n421 = case shown="True" w846 {
          tunnel: ["" "Data: saveCalibration\nData: saveiRF\nRun: CaliIncrement"] -> w845
          frame False {
          }
          frame True {
          }
        }
        n422 = call <vilib>:"Add State(s) to Queue__JKI_lib_State_Machine.vi"("State(s) in Front (\"\")"=w845, "State(s) in (\"\")"=w896) -> ("States Out"=w895:string)  [unwired: 13 in]
      }
      frame "Data: saveRunData" {
        (unwired) i16 0 ("width (-)")
        # "Save FLIm data to disk.\n(Save to LV tdms file format)"
        n423 = Unbundle By Name(w935) -> ("Pathes.DataPath"=w934:path, "CaseID"=w902:string, "IDs.RunID"=w901:i8, "Ch1Data"=w928:dbl[][], "Ch2Data"=w924:dbl[][], "Ch3Data"=w920:dbl[][], "V1"=w916:dbl[], "V2"=w913:dbl[], "V3"=w911:dbl[])
        n424 = Format Value(string ("")=w902, format string="%02d", value (0)=w901) -> (output string=w899:string)
        n425 = Build Path(base path=w934, name or relative path=w899) -> (appended path=w933:path)
        n426 = TDMS Open(8:w906, 10:T11."open or create" ("operation (0:open)"), 11:w933) -> (0:w930:errorcluster, 3:w931:refnum<k34>)  [unwired: 4 in]
        n427 = TDMS Write(0:w931, 5:"CH1Data" ("group name in (Untitled)"), 9:w928, 11:w930) -> (4:w927:refnum<k34>, 15:w926:errorcluster)  [unwired: 2 in, 2 out]
        n428 = TDMS Write(0:w927, 5:"Ch2Data" ("group name in (Untitled)"), 9:w924, 11:w926) -> (4:w922:refnum<k34>, 15:w921:errorcluster)  [unwired: 2 in, 2 out]
        n429 = TDMS Write(0:w922, 5:"Ch3Data" ("group name in (Untitled)"), 9:w920, 11:w921) -> (4:w919:refnum<k34>, 15:w918:errorcluster)  [unwired: 2 in, 2 out]
        n430 = TDMS Write(0:w919, 5:"Ch1V" ("group name in (Untitled)"), 9:w916, 11:w918) -> (4:w905:refnum<k34>, 15:w915:errorcluster)  [unwired: 2 in, 2 out]
        n431 = TDMS Write(0:w905, 5:"Ch2V" ("group name in (Untitled)"), 9:w913, 11:w915) -> (4:w910:refnum<k34>, 15:w909:errorcluster)  [unwired: 2 in, 2 out]
        n432 = TDMS Write(0:w910, 5:"Ch3V" ("group name in (Untitled)"), 9:w911, 11:w909) -> (4:w908:refnum<k34>, 15:w907:errorcluster)  [unwired: 2 in, 2 out]
        n433 = TDMS Close(8:w907, 11:w908) -> (0:w904:errorcluster)  [unwired: 1 out]
        n434 = case shown="No Error" w904 {
          tunnel: [w939 ""] -> w903
          frame No Error {
            w939 = "Run: Increment"  # Run: Increment
          }
          frame Error {
          }
        }
        n435 = call <vilib>:"Add State(s) to Queue__JKI_lib_State_Machine.vi"("State(s) in Front (\"\")"=w903, "State(s) in (\"\")"=w938) -> ("States Out"=w937:string)  [unwired: 13 in]
      }
      frame "Data: Cleanup" {
        # "Cleanup any data and references, here.\n(this is called automatically, by the Macro: Exit)"
        n436 = Unbundle By Name(w942) -> ("Core.Current VI Reference"=w945:refnum<vi>)
        n437 = Close Reference(reference=w945, error in (no error)=w944) -> (error out=w943:errorcluster)
        n438 = call <vilib>:"Add State(s) to Queue__JKI_lib_State_Machine.vi"("State(s) in (\"\")"=w947) -> ("States Out"=w946:string)  [unwired: 14 in]
      }
      frame "---------- Core ----------" {
        # "Do not put any code in this frame.\n(it is a separator no-op)"
        n439 = call <vilib>:"Add State(s) to Queue__JKI_lib_State_Machine.vi"("State(s) in (\"\")"=w952) -> ("States Out"=w951:string)  [unwired: 14 in]
      }
      frame Default {
        w963 = 42 items=["No error", "Argument error", "Memory is full", "Out of zone", "End of file", "File already open", "Generic file I/O error", "File not found", "File permission error", "Disk is full", "Duplicate path", "Too many files open", "System feature not enabled", "Resource file not found", "Cannot add resource", "Resource not found", "Image not found", "Image memory error", "Pen does not exist", "Config type invalid", "Config token not found", "Config parse error", "Config memory error", "Bad external code format", "Bad external code offset", "External code not present", "Null window", "Destroy window error", "Null menu", "Print aborted", "Bad print record", "Print driver error", "Windows error during printing", "Memory error during printing", "Print dialog error", "Generic print error", "Invalid device refnum", "Device not found", "Device parameter error", "Device unit error", "Cannot open device", "Device call aborted", "Generic error", "Cancelled by user", "Object ID too low", "Object ID too high", "Object not in heap", "Unknown heap", "Unknown object (invalid DefProc)", "Unknown object (DefProc not in table)", "Message out of range", "Invalid (null) method", "Unknown message", "Manager call not supported", "Bad address", "Network operation in progress", "Network operation timed out", "Connection is busy", "Network attribute not supported", "Network error", "Address in use", "System out of memory", "Connection aborted", "Connection refused", "Not connected", "Already connected", "Connection closed", "Initialization error (interapplication manager)", "Bad occurrence", "Wait on unbound occurrence handler", "Occurrence queue overflow", "Datalog type conflict", "Unused", "Unrecognized type (interapplication manager)", "Memory corrupt", "Failed to make temporary DLL", "Old CIN version", "Drag socket not found", "Failed to load drop-object", "Failed to register OLE object", "Failed to release OLE object", "Format specifier type mismatch", "Unknown format specifier", "Too few format specifiers", "Too many format specifiers", "Scan failed", "Newer CIN version", "Error converting to variant", "Runtime menu error", "Password tampered", "Variant attribute not found", "Incompatible variant data type", "Event data is not available", "Event Store is not present", "Occurrence is not found", "Event Queue is not created", "Event info is not available", "Refnum passed is NULL", "Error retrieving Class GUID", "Error retrieving CoClass GUID", "Error retrieving TypeLib GUID.", "Bad built application magic bytes.", "Specific driver is different from the specific driver associated with the Logical Name.", "There is no session opened to the class driver.", "Max Error", "MAX - Error with config objects", "MAX - Error loading configuration", "MAX - Group not supported"]
        # "Current State"
        # "Do not delete, rename, or modify this frame.\n(this is used to capture unhandled states and typos)"
        # "Handle mistyped state name (developer tool)"
        n440 = Format Into String(format string="Software Exception: Unhandled State \"%s\"." ("message"), error in=w959, w954) -> (resulting string=w962:string, error out=w961:errorcluster)  [unwired: 1 in]
        n441 = call <vilib>:"Error Cluster From Error Code.vi"("show call chain? (False)"=TRUE, "error in (no error)"=w961, "error message (\"\")"=w962, "error code (0)"=w963) -> ("error out"=w960:errorcluster)  [unwired: 5 in]
        n442 = call <vilib>:"Add State(s) to Queue__JKI_lib_State_Machine.vi"("State(s) in (\"\")"=w958) -> ("States Out"=w957:string)  [unwired: 14 in]
      }
      frame "Initialize Core Data" {
        # "Build default path based on the location of project"
        # "Do not delete, rename, or modify this frame.\n(this is used to determine panel behavior on exit)"
        # "originally closed?"
        # "exe?"
        # "If panel starts closed or is an EXE, then close it when we exit"
        n443 = call <vilib>:"Application Directory.vi"() -> ("Application Directory"=w965:path)
        n444 = property class="App"() -> ("App.Kind"=w979:T13)  [unwired: 2 in, 2 out]
        n445 = property class="VI"() -> ("FP.State"=w973:T12)  [unwired: 2 in, 2 out]
        n446 = control-ref of="Current VI Reference"() -> (w974:refnum<vi>)
        n447 = Equal?(x=w973, y=T12."Closed" ("Front Panel Window:State")) -> (x = y?=w971:bool)
        n448 = Equal?(x=w979, y=T13."Run Time System" ("Application:Kind")) -> (x = y?=w977:bool)
        n449 = Build Path(base path=w965, name or relative path="Data") -> (appended path=w969:path)
        n450 = Build Path(base path=w965, name or relative path="SystemTemp") -> (appended path=w966:path)
        n451 = Or(x=w971, y=w977) -> (x .or. y?=w975:bool)
        n452 = Bundle By Name(cluster=w976, "Core.Current VI Reference"=w974, "Core.Close Panel on Exit?"=w975, "DefaultPath"=w969, "TempPath"=w966) -> (w981:T16)
        n453 = call <vilib>:"Add State(s) to Queue__JKI_lib_State_Machine.vi"("State(s) in (\"\")"=w983) -> ("States Out"=w982:string)  [unwired: 14 in]
      }
      frame "Error Handler" {
        # "Unhandled Error -- Display it"
        # "Handle any errors here.\nYou can also output any states to clean-up after errors occur"
        # "Clear error"
        n454 = Unbundle By Name(w984) -> ("code"=w986:i32)
        n455 = case shown="5002" w986 {
          tunnel: ["Macro: Exit" w996 w1002] -> w985
          tunnel: w984 -> [w992 _ _]
          frame Default {
            w994 = T25 2 items=["no dialog", "OK message", "continue or stop message", "OK message + warnings", "continue/stop + warnings"] ("type of dialog (OK msg:1)")
            n456 = call <vilib>:"General Error Handler.vi"("type of dialog (OK msg:1)"=w994, "error in (no error)"=w992) -> ()  [unwired: 9 in, 5 out]
          }
          frame 5002 {
            n457 = Two Button Dialog(message="Laser interlock open! Please close interlock and try again! ", 1:"Safely Shutdown" ("F button name (\"Cancel\")"), 2:"OK" ("T button name (\"OK\")")) -> (T button?=w997:bool)
            n458 = case shown="False" w997 {
              tunnel: ["Macro: Exit" "355 Laser: CheckControllerStatus"] -> w996
              frame False {
              }
              frame True {
              }
            }
          }
          frame 5001 {
            n459 = Two Button Dialog(message="Unable to connect to imaging computer, do you want to run data aquisiton along? ", 1:"No" ("F button name (\"Cancel\")"), 2:"Yes" ("T button name (\"OK\")")) -> (T button?=w1003:bool)
            n460 = case shown="True" w1003 {
              tunnel: ["Macro: Exit" ""] -> w1002
              frame False {
              }
              frame True {
              }
            }
          }
        }
        n461 = call <vilib>:"Add State(s) to Queue__JKI_lib_State_Machine.vi"("State(s) in Front (\"\")"=w985, "State(s) in (\"\")"=w991) -> ("States Out"=w990:string)  [unwired: 13 in]
      }
      frame "Exit" {
        # "Do not put any code in this frame.\n(No errors that occur here will be handled.)"
        n462 = call <vilib>:"Add State(s) to Queue__JKI_lib_State_Machine.vi"("State(s) in (\"\")"=w1014) -> ("States Out"=w1013:string)  [unwired: 14 in]
      }
      frame "---------- Macro ----------" {
        # "Do not put any code in this frame.\n(It is a separator no-op. You can make a copy of this frame to create a new Macro frame)"
        n463 = call <vilib>:"Add State(s) to Queue__JKI_lib_State_Machine.vi"("State(s) in (\"\")"=w1019) -> ("States Out"=w1018:string)  [unwired: 14 in]
      }
      frame "Macro: Initialize" {
        # "load Labjack setting 1st as it contaisn laser pin infortmation"
        # "start laser 1st, need 7.5s for laser to get ready"
        # "Initialization Macro\n(This is called once, when the VI starts)"
        n464 = call <vilib>:"Add State(s) to Queue__JKI_lib_State_Machine.vi"("State(s) in Front (\"\")"="UI: showDisclaimer\nUI: Cursor Set >> Busy\nGraph: AddCursors\nData: Initialize\nInitialize Core Data\nUI: Initialize\nUI: Front Panel State >> Open\nUI: Update\nMacro: LoadSysConfig\nLabJack: Open\nLabJack: SetDefaultSub\nLED: Yellow\nLED: OpenVIRef\nLED: Breath >> True\nUI: Update\n355 Laser: Laser enable/disable\n355 Laser: Dewelling>>500\n355 Laser: CheckControllerStatus\nUI: Update\nLabJack: 355_PWM_Config\nLabJack: AB_PWM_Config\nTCP: Initialize\nTCP: SyncTime\nUI: Update\n", "State(s) in (\"\")"="Digitizer: Initialize\nDigitizer: Config\nUI: Update\nAimingBeam: Initialize\nAimingBeam: Set Status>>Enable\nAimingBeam: Set Current\nUI: Update\n355 Laser: Check Dewelling\nUI: Cursor Set >> Idle\nCase: GetID\nUI: Update\nTCP: SendSettingMacro\nCase: CreatFileStruct\nUI: Update\nData: loadLastUseMacro\nDeconEngine: InitilizeMacro\nUI: ReadyForAquisition\nLED: Breath >> False") -> ("States Out"=w1020:string)  [unwired: 13 in]
        n465 = call <vilib>:"Add State(s) to Queue__JKI_lib_State_Machine.vi"("State(s) in Front (\"\")"=w1020, "State(s) in (\"\")"=w1028) -> ("States Out"=w1027:string)  [unwired: 13 in]
        "Help" <- "Hover over controls to see help!" ("Help")
      }
      frame "Macro: LoadSysConfig" {
        # "System configuration Macro\n(Load configurations for different component of the system)"
        n466 = call <vilib>:"Add State(s) to Queue__JKI_lib_State_Machine.vi"("State(s) in Front (\"\")"="SysConfig: Load Sys Config\nSysConfig: Load Digitizer Setting\nSysConfig: Load AB setting\nSysConfig: Load LJ Pinout\nSysConfig: Load 355 PWM\nSysConfig: Load AB PWM", "State(s) in (\"\")"=w1034) -> ("States Out"=w1033:string)  [unwired: 13 in]
      }
      frame "Macro: Exit" {
        # "close LJ last"
        # "check whether hardware is initilized, if so close, if not do nothing"
        # "Exit Macro, close all hardware\n(This is called once, when the VI exits)"
        n467 = Unbundle By Name(w1054) -> ("System Status.TCP/IP"=w1042:bool, "System Status.Digitizer"=w1050:bool, "System Status.Aiming Beam"=w1049:bool, "System Status.355 Laser"=w1048:bool, "System Status.Labjack"=w1038:bool, "Core.Close Panel on Exit?"=w1043:bool)
        n468 = case shown="True" w1050 {
          tunnel: ["" "Digitizer: Close"] -> w1045
          frame False {
          }
          frame True {
          }
        }
        n469 = case shown="True" w1042 {
          tunnel: ["" "TCP: Close"] -> w1044
          frame False {
          }
          frame True {
          }
        }
        n470 = case shown="True" w1038 {
          tunnel: ["" "LabJack: SetDefaultAndClose"] -> w1035
          frame False {
          }
          frame True {
          }
        }
        n471 = case shown="True" w1049 {
          tunnel: ["" "AimingBeam: Set Status >> Disable\nAimingBeam: Close"] -> w1037
          frame False {
          }
          frame True {
          }
        }
        n472 = case shown="True" w1048 {
          tunnel: ["" "355 Laser: Close\n355 Laser: CheckControllerStatus"] -> w1036
          frame False {
          }
          frame True {
          }
        }
        n473 = Select(t="UI: Front Panel State >> Close", s=w1043, f="") -> (s? t:f=w1039:string)
        n474 = call <vilib>:"Add State(s) to Queue__JKI_lib_State_Machine.vi"("State(s) in Front (\"\")"=w1044, "State(s) in (\"\")"=w1045, "State(s) at Back (\"\")"=w1037) -> ("States Out"=w1047:string)  [unwired: 12 in]
        n475 = call <vilib>:"Add State(s) to Queue__JKI_lib_State_Machine.vi"("State(s) in Front (\"\")"=w1047, "State(s) in (\"\")"=w1036, "State(s) at Back (\"\")"=w1035) -> ("States Out"=w1041:string)  [unwired: 12 in]
        n476 = call <vilib>:"Add State(s) to Queue__JKI_lib_State_Machine.vi"("State(s) in Front (\"\")"=w1041, "State(s) in (\"\")"="UI: Update\nUI: Reset\nLED: CloseVIRef\nQueue: Destory\nData: Cleanup\nExit", "State(s) at Back (\"\")"=w1039) -> ("States Out"=w1051:string)  [unwired: 12 in]
        n477 = call <vilib>:"Add State(s) to Queue__JKI_lib_State_Machine.vi"("State(s) in Front (\"\")"=w1051, "State(s) in (\"\")"=w1057) -> ("States Out"=w1056:string)  [unwired: 13 in]
      }
      frame "---------- AimingBeam ----------" {
        # "Template Separator\n(You can make a copy of, or modify, this frame)"
        n478 = call <vilib>:"Add State(s) to Queue__JKI_lib_State_Machine.vi"("State(s) in (\"\")"=w1072) -> ("States Out"=w1071:string)  [unwired: 14 in]
      }
      frame "AimingBeam: Initialize" {
        # "set aiming beam button color"
        # "Open COM port for Aiming Beam\n(Require USB connection)"
        n479 = Unbundle By Name(w1074) -> ("AB Cluster.Aiming Beam COM Port"=w1082:refnum<visa-resource-name>)
        n480 = call-poly "VISA Configure Serial Port"("VISA resource name"=w1082, "Enable Termination\nChar (T)"=TRUE ("Enable Termination\nChar (T)"), "baud rate (9600)"=u32 9600, "error in (no error)"=w1079) -> ("error out"=w1078:errorcluster)  [unwired: 10 in, 1 out]
        n481 = Unbundle By Name(w1078) -> ("status"=w1077:bool)
        n482 = Not(x=w1077) -> (.not. x?=w1076:bool)
        n483 = Bundle By Name(cluster=w1074, "System Status.Aiming Beam"=w1076) -> (w1075:T16)
        n484 = call <vilib>:"Add State(s) to Queue__JKI_lib_State_Machine.vi"("State(s) in (\"\")"=w1084) -> ("States Out"=w1083:string)  [unwired: 14 in]
      }
      frame "AimingBeam: Close" {
        # "Close Aiming Beam COM port\n(Require USB connection to Aiming Beam Laser)"
        n485 = Unbundle By Name(w1087) -> ("AB Cluster.Aiming Beam COM Port"=w1091:refnum<visa-resource-name>)
        n486 = VISA Close(VISA resource name=w1091, error in (no error)=w1089) -> (error out=w1090:errorcluster)
        n487 = Bundle By Name(cluster=w1087, "System Status.Aiming Beam"=FALSE) -> (w1088:T16)
        n488 = call <vilib>:"Add State(s) to Queue__JKI_lib_State_Machine.vi"("State(s) in (\"\")"=w1093) -> ("States Out"=w1092:string)  [unwired: 14 in]
      }
      frame "AimingBeam: Set Current" {
        # "Set Aiming Beam Current\n(You can make a copy of, or modify, this frame)"
        n489 = Unbundle By Name(w1113) -> ("AB Cluster.Aiming Beam COM Port"=w1106:refnum<visa-resource-name>, "AB Cluster.Max Current"=w1102:dbl, "AB Cluster.Default Current"=w1104:dbl, "AB Cluster.Min Current"=w1103:dbl)
        n490 = In Range and Coerce(upper limit=w1102, x=w1104, lower limit=w1103) -> (coerced(x)=w1099:dbl)  [unwired: 1 out]
        n491 = property on="Aiming beam toggle" class="Bool (strict)"() -> ("Caption.Text"=w1094:string)  [unwired: 2 in, 2 out]
        n492 = Number To Fractional String(number=w1099, precision (6)=i16 2) -> (F-format string=w1107:string)  [unwired: 2 in]
        n493 = Concatenate Strings("slc:", w1107, "\r", "\n") -> (w1110:string)
        n494 = Number To Decimal String(number=w1099, width (-)=i16 2) -> (decimal integer string=w1098:string)
        n495 = VISA Write(VISA resource name=w1106, write buffer=w1110, error in (no error)=w1101) -> (error out=w1105:errorcluster)  [unwired: 2 out]
        n496 = Concatenate Strings(w1094, w1098, "mA" ("string")) -> (w1096:string)
        n497 = property on="Aiming beam toggle" class="Bool (strict)"("Caption.Text"=w1096) -> ()  [unwired: 2 in, 2 out]
        n498 = call <vilib>:"Add State(s) to Queue__JKI_lib_State_Machine.vi"("State(s) in (\"\")"=w1115) -> ("States Out"=w1114:string)  [unwired: 14 in]
      }
      frame "AimingBeam: Set Status" {
        # "Enable Aiming Beam\n(Usage: \"AimingBeam: Set >> Enable|Disable\")"
        n499 = Unbundle By Name(w1122) -> ("AB Cluster.Aiming Beam COM Port"=w1119:refnum<visa-resource-name>)
        n500 = case shown="\"Enable\"" w1121 {
          tunnel: [w1125 w1129] -> w1120
          frame "Disable", Default {
            n501 = Concatenate Strings("cof", "\r", "\n") -> (w1125:string)
          }
          frame "Enable" {
            n502 = Concatenate Strings("con", "\r", "\n") -> (w1129:string)
          }
        }
        n503 = VISA Write(VISA resource name=w1119, write buffer=w1120, error in (no error)=w1117) -> (error out=w1118:errorcluster)  [unwired: 2 out]
        n504 = call <vilib>:"Add State(s) to Queue__JKI_lib_State_Machine.vi"("State(s) in (\"\")"=w1124) -> ("States Out"=w1123:string)  [unwired: 14 in]
      }
      frame "AimingBeam: GetPWMStatus" {
        # "Get aiming beam PWM status\n()"
        n505 = Unbundle By Name(w1133) -> ("LJ Pinout.AimingBeam PWM"=w1142:string)
        n506 = call "LabJack_FGV.vi"("Operation(Read)"=enum16{"Write", "Read"}."Read" ("Operation"), "error in (no error)"=w1135) -> ("error out"=w1139:errorcluster, "Read data"=w1140:i32)  [unwired: 8 in]
        n507 = Concatenate Strings(w1142, "_EF_ENABLE" ("string")) -> (w1138:string)
        n508 = call "LJM_eReadName.vi"("Handle In"=w1140, "Name"=w1138, "error in"=w1139) -> ("Value"=w1137:dbl, "error out"=w1134:errorcluster)  [unwired: 10 in, 1 out]
        n509 = Greater Than 0?(x=w1137) -> (x > 0?=w1136:bool)
        n510 = case shown="False" w1136 {
          frame False {
            # "PWM is off\nset color to dark green"
            n511 = local write "Aiming beam toggle"(FALSE ("Aimging beam")) -> ()
          }
          frame True {
            # "PWM is on\nset color to light green"
            n512 = local write "Aiming beam toggle"(TRUE ("Aimging beam")) -> ()
          }
        }
        n513 = call <vilib>:"Add State(s) to Queue__JKI_lib_State_Machine.vi"("State(s) in (\"\")"=w1146) -> ("States Out"=w1145:string)  [unwired: 14 in]
      }
      frame "---------- Case ----------" {
        # "Template Separator\n(You can make a copy of, or modify, this frame)"
        n514 = call <vilib>:"Add State(s) to Queue__JKI_lib_State_Machine.vi"("State(s) in (\"\")"=w1153) -> ("States Out"=w1152:string)  [unwired: 14 in]
      }
      frame "Case: getCaliID" {
        # "Get Calibration file #\n(You can make a copy of, or modify, this frame)"
        n515 = Unbundle By Name(w1155) -> ("Pathes.CaliPath"=w1158:path)
        n516 = call <vilib>:"Recursive File List.vi"("pattern"="*.tdms", "Treat LLBs as Folders?"=FALSE, "Folder Path"=w1158) -> ("All Files in Dir"=w1163:path[])  [unwired: 4 in, 4 out]
        n517 = for {
          tunnel: w1163 -> [w1173] mode=indexing
          tunnel: [w1172] -> w1162 mode=indexing
          tunnel: "Calibration" -> [w1169]
          n518 = Strip Path(path=w1173) -> (name=w1170:string)  [unwired: 1 out]
          n519 = Search and Replace String(input string=w1170, search string=w1169) -> (result string=w1168:string)  [unwired: 6 in, 3 out]
          n520 = Scan From String(format string="%d" ("string"), input string=w1168) -> (output 1=w1172:i32)  [unwired: 3 in, 3 out]
        }
        n521 = Array Max & Min(array=w1162) -> (max value=w1161:i32)  [unwired: 3 out]
        n522 = Increment(x=w1161) -> (x+1=w1154:i32)
        n523 = Bundle By Name(cluster=w1155, "IDs.Cali ID"=w1154) -> (w1156:T16)
        n524 = call <vilib>:"Add State(s) to Queue__JKI_lib_State_Machine.vi"("State(s) in (\"\")"=w1167) -> ("States Out"=w1166:string)  [unwired: 14 in]
      }
      frame "Case: getBGID" {
        # "Get background #\n(You can make a copy of, or modify, this frame)"
        n525 = Unbundle By Name(w1174) -> ("Pathes.BG Path"=w1182:path)
        n526 = call <vilib>:"Recursive File List.vi"("pattern"="*.tdms", "Treat LLBs as Folders?"=FALSE, "Folder Path"=w1182) -> ("All Files in Dir"=w1178:path[])  [unwired: 4 in, 4 out]
        n527 = for {
          tunnel: w1178 -> [w1193] mode=indexing
          tunnel: [w1192] -> w1179 mode=indexing
          tunnel: "Background" ("name or relative path") -> [w1189]
          n528 = Strip Path(path=w1193) -> (name=w1190:string)  [unwired: 1 out]
          n529 = Search and Replace String(input string=w1190, search string=w1189) -> (result string=w1188:string)  [unwired: 6 in, 3 out]
          n530 = Scan From String(format string="%d" ("string"), input string=w1188) -> (output 1=w1192:i32)  [unwired: 3 in, 3 out]
        }
        n531 = Array Max & Min(array=w1179) -> (max value=w1180:i32)  [unwired: 3 out]
        n532 = Increment(x=w1180) -> (x+1=w1176:i32)
        n533 = Bundle By Name(cluster=w1174, "IDs.BG ID"=w1176) -> (w1175:T16)
        n534 = call <vilib>:"Add State(s) to Queue__JKI_lib_State_Machine.vi"("State(s) in (\"\")"=w1187) -> ("States Out"=w1186:string)  [unwired: 14 in]
      }
      frame "Case: getRunID" {
        # "Check folder for run ID\n(You can make a copy of, or modify, this frame)"
        n535 = Unbundle By Name(w1199) -> ("Pathes.DataPath"=w1198:path, "CaseID"=w1194:string)
        n536 = Build Array("Background" ("name or relative path"), "Calibration") -> (w1206:string[])
        n537 = call <vilib>:"Recursive File List.vi"("Folders to Exclude"=w1206, "pattern"="*.tdms", "Treat LLBs as Folders?"=FALSE, "Folder Path"=w1198) -> ("All Files in Dir"=w1195:path[])  [unwired: 3 in, 4 out]
        n538 = for {
          tunnel: w1195 -> [w1216] mode=indexing
          tunnel: [w1215] -> w1202 mode=indexing
          tunnel: w1194 -> [w1212]
          n539 = Strip Path(path=w1216) -> (name=w1213:string)  [unwired: 1 out]
          n540 = Search and Replace String(input string=w1213, search string=w1212) -> (result string=w1211:string)  [unwired: 6 in, 3 out]
          n541 = Scan From String(format string="%d" ("string"), input string=w1211) -> (output 1=w1215:i32)  [unwired: 3 in, 3 out]
        }
        n542 = Array Max & Min(array=w1202) -> (max value=w1203:i32)  [unwired: 3 out]
        n543 = Increment(x=w1203) -> (x+1=w1201:i32)
        n544 = Bundle By Name(cluster=w1199, "IDs.RunID"=w1201) -> (w1200:T16)
        n545 = call <vilib>:"Add State(s) to Queue__JKI_lib_State_Machine.vi"("State(s) in (\"\")"=w1210) -> ("States Out"=w1209:string)  [unwired: 14 in]
      }
      frame "Case: CreatFileStruct" {
        # "Creat case file structure"
        n546 = Unbundle By Name(w1228) -> ("DefaultPath"=w1234:path, "CaseID"=w1219:string)
        n547 = Build Path(base path=w1234, name or relative path=w1219) -> (appended path=w1233:path)
        n548 = call <vilib>:"Check if File or Folder Exists.vi"("error in (no error)"=w1226, "path"=w1233) -> ("error out"=w1230:errorcluster, "file or folder exists?"=w1232:bool, "dup path"=w1231:path)  [unwired: 7 in]
        n549 = case shown="True" w1232 {
          tunnel: w1231 -> [w1251 w1259]
          tunnel: w1230 -> [w1249 w1254]
          tunnel: [w1243 w1259] -> w1224
          tunnel: [w1247 w1261] -> w1227
          tunnel: [u32 1 u32 0] -> w1218
          tunnel: [w1245 w1264] -> w1223
          tunnel: "Background" ("name or relative path") -> [w1244 w1256]
          tunnel: "Calibration" -> [w1242 w1255]
          tunnel: [w1238 w1257] -> w1220
          tunnel: w1219 -> [_ _]
          tunnel: ["" "Case: getRunID\nCase: getBGID\nCase: getCaliID"] -> w1217
          frame False {
            # "Folder not exist. Creat folders."
            n550 = Create Folder(path (use dialog)=w1251, error in=w1249) -> (created path=w1243:path, error out=w1240:errorcluster)  [unwired: 1 in, 1 out]
            n551 = Build Path(base path=w1243, name or relative path=w1242) -> (appended path=w1241:path)
            n552 = Build Path(base path=w1243, name or relative path=w1244) -> (appended path=w1250:path)
            n553 = Create Folder(path (use dialog)=w1250, error in=w1240) -> (created path=w1245:path, error out=w1246:errorcluster)  [unwired: 1 in, 1 out]
            n554 = Create Folder(path (use dialog)=w1241, error in=w1240) -> (created path=w1238:path, error out=w1239:errorcluster)  [unwired: 1 in, 1 out]
            n555 = Merge Errors(w1246, w1239) -> (w1247:errorcluster)
          }
          frame True {
            # "Folder exsit, check file #"
            n556 = Build Path(base path=w1259, name or relative path=w1255) -> (appended path=w1260:path)
            n557 = Build Path(base path=w1259, name or relative path=w1256) -> (appended path=w1265:path)
            n558 = call <vilib>:"Check if File or Folder Exists.vi"("path"=w1260) -> ("file or folder exists?"=w1258:bool, "dup path"=w1257:path)  [unwired: 8 in, 1 out]
            n559 = call <vilib>:"Check if File or Folder Exists.vi"("path"=w1265) -> ("file or folder exists?"=w1263:bool, "dup path"=w1264:path)  [unwired: 8 in, 1 out]
            n560 = And(x=w1263, y=w1258) -> (x .and. y?=w1262:bool)
            n561 = case shown="False" w1262 {
              tunnel: w1254 -> [_ w1267]
              tunnel: [errorcluster {"status"=TRUE, "code"=5003, "source"="File structure error."} ("error out") w1267] -> w1261
              frame False {
              }
              frame True {
              }
            }
          }
        }
        n562 = Bundle By Name(cluster=w1228, "Pathes.DataPath"=w1224, "Pathes.BG Path"=w1223, "Pathes.CaliPath"=w1220, "IDs.RunID"=w1218, "IDs.BG ID"=w1218, "IDs.Cali ID"=w1218) -> (w1229:T16)
        n563 = call <vilib>:"Add State(s) to Queue__JKI_lib_State_Machine.vi"("State(s) in Front (\"\")"=w1217, "State(s) in (\"\")"=w1236) -> ("States Out"=w1235:string)  [unwired: 13 in]
      }
      frame "Case: GetID" {
        # "Template Separator\n(You can make a copy of, or modify, this frame)"
        n564 = call "set_subjectID.vi"() -> ("subject_id"=w1268:string)  [unwired: 10 in]
        n565 = Bundle By Name(cluster=w1270, "CaseID"=w1268) -> (w1271:T16)
        n566 = call <vilib>:"Add State(s) to Queue__JKI_lib_State_Machine.vi"("State(s) in (\"\")"=w1274) -> ("States Out"=w1273:string)  [unwired: 14 in]
      }
      frame "---------- DeconEngine ----------" {
        # "start data aquisition and then set irfAligh to ture and decon channel to 1,2 and 3."
        # "Template Separator\n(You can make a copy of, or modify, this frame)"
        n567 = call <vilib>:"Add State(s) to Queue__JKI_lib_State_Machine.vi"("State(s) in (\"\")"=w1279) -> ("States Out"=w1278:string)  [unwired: 14 in]
      }
      frame "DeconEngine: InitilizeMacro" {
        # "start data aquisition and then set irfAligh to ture and decon channel to 1,2 and 3."
        # "Initilize Decon Engine for all channel\n(You can make a copy of, or modify, this frame)"
        n568 = call <vilib>:"Add State(s) to Queue__JKI_lib_State_Machine.vi"("State(s) in Front (\"\")"="DeconEngine: InitializeCh1\nDeconEngine: InitializeCh2\nDeconEngine: InitializeCh3" ("State(s) in Front (\"\")"), "State(s) in (\"\")"=w1285) -> ("States Out"=w1284:string)  [unwired: 13 in]
      }
      frame "DeconEngine: InitializeCh1" {
        w1309 = refnum<class "LaguerreDeconEngineClass.lvclass"> refnum  # Ch1DeconObj
        # "Initilize Laguerre Deconvolution engine Object\n(You can make a copy of, or modify, this frame)"
        n569 = global read "GlobalVariables.vi" "LastUseiRF"() -> (w1287:T26)
        n570 = call "FLImDAQ_FGV.vi"("error in (no error)"=w1294) -> ("error out"=w1305:errorcluster, "Read data"=w1304:T5)  [unwired: 9 in]
        n571 = call "setLaguerreOrder.vi"("error in (no error)"=w1305, "LaguerreOrder"=u32 12, "LaguerreDeconClass in"=w1309) -> ("error out"=w1306:errorcluster, "LaguerreDeconClass out"=w1307:refnum<class "LaguerreDeconEngineClass.lvclass">)  [unwired: 7 in]
        n572 = Unbundle By Name(w1304) -> ("min record length"=w1303:i32)
        n573 = Unbundle By Name(w1287) -> ("Ch1 iRF"=w1286:dbl[])
        n574 = call "setDataLength.vi"("error in (no error)"=w1306, "dataLength"=w1303, "LaguerreDeconClass in"=w1307) -> ("error out"=w1302:errorcluster, "LaguerreDeconClass out"=w1301:refnum<class "LaguerreDeconEngineClass.lvclass">)  [unwired: 7 in]
        n575 = call "setIRF.vi"("error in (no error)"=w1302, "iRF"=w1286, "LaguerreDeconClass in"=w1301) -> ("error out"=w1299:errorcluster, "LaguerreDeconClass out"=w1300:refnum<class "LaguerreDeconEngineClass.lvclass">)  [unwired: 7 in]
        n576 = call "computeAlpha.vi"("error in (no error)"=w1299, "LaguerreDeconClass in"=w1300) -> ("error out"=w1297:errorcluster, "LaguerreDeconClass out"=w1298:refnum<class "LaguerreDeconEngineClass.lvclass">)  [unwired: 8 in]
        n577 = call "dataInitilize.vi"("error in (no error)"=w1297, "LaguerreDeconClass in"=w1298) -> ("error out"=w1295:errorcluster, "LaguerreDeconClass out"=w1296:refnum<class "LaguerreDeconEngineClass.lvclass">)  [unwired: 8 in]
        n578 = call "computeDeconMatrix.vi"("error in (no error)"=w1295, "LaguerreDeconClass in"=w1296) -> ("error out"=w1291:errorcluster, "LaguerreDeconClass out"=w1293:refnum<class "LaguerreDeconEngineClass.lvclass">)  [unwired: 8 in]
        n579 = call "Ch1DeconEngineFGV.vi"("Error In"=w1291, "action(read)"=enum16{"write", "read"}."write" ("action"), "Ch1DeconEngine in"=w1293) -> ("Error Out"=w1290:errorcluster)  [unwired: 7 in, 1 out]
        n580 = call <vilib>:"Add State(s) to Queue__JKI_lib_State_Machine.vi"("State(s) in (\"\")"=w1311) -> ("States Out"=w1310:string)  [unwired: 14 in]
      }
      frame "DeconEngine: InitializeCh2" {
        w1335 = refnum<class "LaguerreDeconEngineClass.lvclass"> refnum  # Ch2DeconObj
        # "Initilize Laguerre Deconvolution engine Object\n(You can make a copy of, or modify, this frame)"
        n581 = global read "GlobalVariables.vi" "LastUseiRF"() -> (w1313:T26)
        n582 = call "FLImDAQ_FGV.vi"("error in (no error)"=w1321) -> ("error out"=w1314:errorcluster, "Read data"=w1331:T5)  [unwired: 9 in]
        n583 = call "setLaguerreOrder.vi"("error in (no error)"=w1314, "LaguerreOrder"=u32 12, "LaguerreDeconClass in"=w1335) -> ("error out"=w1332:errorcluster, "LaguerreDeconClass out"=w1333:refnum<class "LaguerreDeconEngineClass.lvclass">)  [unwired: 7 in]
        n584 = Unbundle By Name(w1331) -> ("min record length"=w1330:i32)
        n585 = Unbundle By Name(w1313) -> ("Ch2 iRF"=w1312:dbl[])
        n586 = call "setDataLength.vi"("error in (no error)"=w1332, "dataLength"=w1330, "LaguerreDeconClass in"=w1333) -> ("error out"=w1329:errorcluster, "LaguerreDeconClass out"=w1328:refnum<class "LaguerreDeconEngineClass.lvclass">)  [unwired: 7 in]
        n587 = call "setIRF.vi"("error in (no error)"=w1329, "iRF"=w1312, "LaguerreDeconClass in"=w1328) -> ("error out"=w1326:errorcluster, "LaguerreDeconClass out"=w1327:refnum<class "LaguerreDeconEngineClass.lvclass">)  [unwired: 7 in]
        n588 = call "computeAlpha.vi"("error in (no error)"=w1326, "LaguerreDeconClass in"=w1327) -> ("error out"=w1324:errorcluster, "LaguerreDeconClass out"=w1325:refnum<class "LaguerreDeconEngineClass.lvclass">)  [unwired: 8 in]
        n589 = call "dataInitilize.vi"("error in (no error)"=w1324, "LaguerreDeconClass in"=w1325) -> ("error out"=w1322:errorcluster, "LaguerreDeconClass out"=w1323:refnum<class "LaguerreDeconEngineClass.lvclass">)  [unwired: 8 in]
        n590 = call "computeDeconMatrix.vi"("error in (no error)"=w1322, "LaguerreDeconClass in"=w1323) -> ("error out"=w1318:errorcluster, "LaguerreDeconClass out"=w1320:refnum<class "LaguerreDeconEngineClass.lvclass">)  [unwired: 8 in]
        n591 = call "Ch2DeconEngineFGV.vi"("Error In"=w1318, "action(read)"=enum16{"write", "read"}."write" ("action"), "Ch2DeconEngine in"=w1320) -> ("Error Out"=w1317:errorcluster)  [unwired: 7 in, 1 out]
        n592 = call <vilib>:"Add State(s) to Queue__JKI_lib_State_Machine.vi"("State(s) in (\"\")"=w1337) -> ("States Out"=w1336:string)  [unwired: 14 in]
      }
      frame "DeconEngine: InitializeCh3" {
        w1361 = refnum<class "LaguerreDeconEngineClass.lvclass"> refnum  # Ch3DeconObj
        # "Initilize Laguerre Deconvolution engine Object\n(You can make a copy of, or modify, this frame)"
        n593 = call "FLImDAQ_FGV.vi"("error in (no error)"=w1346) -> ("error out"=w1357:errorcluster, "Read data"=w1356:T5)  [unwired: 9 in]
        n594 = global read "GlobalVariables.vi" "LastUseiRF"() -> (w1339:T26)
        n595 = call "setLaguerreOrder.vi"("error in (no error)"=w1357, "LaguerreOrder"=u32 12, "LaguerreDeconClass in"=w1361) -> ("error out"=w1358:errorcluster, "LaguerreDeconClass out"=w1359:refnum<class "LaguerreDeconEngineClass.lvclass">)  [unwired: 7 in]
        n596 = Unbundle By Name(w1356) -> ("min record length"=w1355:i32)
        n597 = Unbundle By Name(w1339) -> ("Ch3 iRF"=w1338:dbl[])
        n598 = call "setDataLength.vi"("error in (no error)"=w1358, "dataLength"=w1355, "LaguerreDeconClass in"=w1359) -> ("error out"=w1354:errorcluster, "LaguerreDeconClass out"=w1353:refnum<class "LaguerreDeconEngineClass.lvclass">)  [unwired: 7 in]
        n599 = call "setIRF.vi"("error in (no error)"=w1354, "iRF"=w1338, "LaguerreDeconClass in"=w1353) -> ("error out"=w1351:errorcluster, "LaguerreDeconClass out"=w1352:refnum<class "LaguerreDeconEngineClass.lvclass">)  [unwired: 7 in]
        n600 = call "computeAlpha.vi"("error in (no error)"=w1351, "LaguerreDeconClass in"=w1352) -> ("error out"=w1349:errorcluster, "LaguerreDeconClass out"=w1350:refnum<class "LaguerreDeconEngineClass.lvclass">)  [unwired: 8 in]
        n601 = call "dataInitilize.vi"("error in (no error)"=w1349, "LaguerreDeconClass in"=w1350) -> ("error out"=w1347:errorcluster, "LaguerreDeconClass out"=w1348:refnum<class "LaguerreDeconEngineClass.lvclass">)  [unwired: 8 in]
        n602 = call "computeDeconMatrix.vi"("error in (no error)"=w1347, "LaguerreDeconClass in"=w1348) -> ("error out"=w1343:errorcluster, "LaguerreDeconClass out"=w1345:refnum<class "LaguerreDeconEngineClass.lvclass">)  [unwired: 8 in]
        n603 = call "Ch3DeconEngineFGV.vi"("Error In"=w1343, "action(read)"=enum16{"write", "read"}."write" ("action"), "Ch3DeconEngine in"=w1345) -> ("Error Out"=w1342:errorcluster)  [unwired: 7 in, 1 out]
        n604 = call <vilib>:"Add State(s) to Queue__JKI_lib_State_Machine.vi"("State(s) in (\"\")"=w1363) -> ("States Out"=w1362:string)  [unwired: 14 in]
      }
      frame "DeconEngine: iRFAlign" {
        # "Template Separator\n(You can make a copy of, or modify, this frame)"
        n605 = call <vilib>:"Add State(s) to Queue__JKI_lib_State_Machine.vi"("State(s) in (\"\")"=w1368) -> ("States Out"=w1367:string)  [unwired: 14 in]
      }
      frame "---------- Digitizer ----------" {
        # "Template Separator\n(You can make a copy of, or modify, this frame)"
        n606 = call <vilib>:"Add State(s) to Queue__JKI_lib_State_Machine.vi"("State(s) in (\"\")"=w1373) -> ("States Out"=w1372:string)  [unwired: 14 in]
      }
      frame "Digitizer: Initialize" {
        # "Initialize digitizer.\nInitialize both digitizer and update status."
        n607 = Unbundle By Name(w1383) -> ("SysConfigCluster.Ch1Enable?"=w1388:bool, "SysConfigCluster.Ch2Enable?"=w1387:bool, "SysConfigCluster.Ch3Enable?"=w1385:bool)
        n608 = call "FLImDAQ_FGV.vi"("error in (no error)"=w1379) -> ("error out"=w1378:errorcluster, "Read data"=w1377:T5)  [unwired: 9 in]
        n609 = property on="Digitizer" class="Bool (strict)"("Blinking"=TRUE) -> ()  [unwired: 2 in, 2 out]
        n610 = Unbundle By Name(w1377) -> ("Digitizer 1"=w1376:refnum<k15>, "Digitizer 2"=w1375:refnum<k15>)
        n611 = Or(x=w1388, y=w1387) -> (x .or. y?=w1386:bool)
        n612 = case shown="True" w1385 {
          tunnel: w1378 -> [w1391 w1393]
          tunnel: [w1391 w1395] -> w1381
          tunnel: w1375 -> [_ w1394]
          frame False {
          }
          frame True {
            n613 = call <instrlib>:"niScope Initialize.vi"("resource name"=w1394, "reset device"=TRUE, "error in"=w1393) -> ("error out"=w1395:errorcluster)  [unwired: 11 in, 1 out]
          }
        }
        n614 = case shown="True" w1386 {
          tunnel: w1378 -> [w1396 w1398]
          tunnel: [w1396 w1400] -> w1382
          tunnel: w1376 -> [_ w1399]
          frame False {
          }
          frame True {
            n615 = call <instrlib>:"niScope Initialize.vi"("resource name"=w1399, "reset device"=TRUE, "error in"=w1398) -> ("error out"=w1400:errorcluster)  [unwired: 11 in, 1 out]
          }
        }
        n616 = Merge Errors(w1382, w1381) -> (w1380:errorcluster)
        n617 = call <vilib>:"Add State(s) to Queue__JKI_lib_State_Machine.vi"("State(s) in (\"\")"=w1390) -> ("States Out"=w1389:string)  [unwired: 14 in]
      }
      frame "Digitizer: Config" {
        # "Synchronize is taking time ~3s."
        # "Config  digitizer\nCall subVi to config digitizer"
        n618 = Unbundle By Name(w1429) -> ("SysConfigCluster.Ch1Enable?"=w1437:bool, "SysConfigCluster.Ch2Enable?"=w1436:bool, "SysConfigCluster.Ch3Enable?"=w1434:bool, "FLImDAQ"=w1431:T22)
        n619 = call "FLImDAQ_FGV.vi"() -> ("Read data"=w1420:T5)  [unwired: 10 in, 1 out]
        n620 = Unbundle By Name(w1420) -> ("Digitizer 1"=w1423:refnum<k15>, "Digitizer 2"=w1422:refnum<k15>)
        n621 = property on="Digitizer" class="Bool (strict)"(error in=w1424, "Blinking"=TRUE) -> (error out=w1425:errorcluster)  [unwired: 1 in, 1 out]
        n622 = Or(x=w1437, y=w1436) -> (x .or. y?=w1435:bool)
        n623 = case shown="True" w1435 {
          tunnel: w1431 -> [_ w1450]
          tunnel: w1425 -> [w1446 w1449]
          tunnel: [w1446 w1448] -> w1432
          tunnel: w1423 -> [_ w1447]
          frame False {
          }
          frame True {
            n624 = call "DigitizerConfig.vi"("error in (no error)"=w1449, "FLImDAQ"=w1450, "IVI Refnum in"=w1447) -> ("error out"=w1448:errorcluster)  [unwired: 7 in, 1 out]
          }
        }
        n625 = case shown="True" w1434 {
          tunnel: w1431 -> [_ w1445]
          tunnel: w1432 -> [w1440 w1444]
          tunnel: [w1440 w1443] -> w1406
          tunnel: w1422 -> [_ w1441]
          frame False {
          }
          frame True {
            n626 = call "DigitizerConfig.vi"("Config Trigger? (T)"=FALSE ("Config Trigge(T)r:"), "error in (no error)"=w1444, "FLImDAQ"=w1445, "IVI Refnum in"=w1441) -> ("error out"=w1443:errorcluster)  [unwired: 6 in, 1 out]
          }
        }
        n627 = call "Digitizer1_FGV.vi"("error in (no error)"=w1406, "Operation (Read)"=enum16{"Write", "Read"}."Read" ("Operation")) -> ("error out"=w1417:errorcluster, "Read data"=w1418:refnum<k15>)  [unwired: 8 in]
        n628 = call <instrlib>:"niScope Get Session Reference.vi"("instrument handle"=w1418, "error in"=w1417) -> ("session reference"=w1410:refnum<k20>, "error out"=w1408:errorcluster)  [unwired: 11 in, 1 out]
        n629 = call "Digitizer2_FGV.vi"("error in (no error)"=w1408, "Operation (Read)"=enum16{"Write", "Read"}."Read" ("Operation")) -> ("error out"=w1414:errorcluster, "Read data"=w1415:refnum<k15>)  [unwired: 8 in]
        n630 = call <instrlib>:"niScope Get Session Reference.vi"("instrument handle"=w1415, "error in"=w1414) -> ("session reference"=w1409:refnum<k20>, "error out"=w1407:errorcluster)  [unwired: 11 in, 1 out]
        n631 = Build Array(w1410, w1409) -> (w1413:refnum<k20>[])
        n632 = call <instrlib>:"niTClk Configure For Homogeneous Triggers.vi"("error in (no error)"=w1407, "sessions"=w1413) -> ("error out"=w1412:errorcluster, "sessions out"=w1411:refnum<k20>[])  [unwired: 8 in]
        n633 = call <instrlib>:"niTClk Synchronize.vi"("error in (no error)"=w1412, "sessions"=w1411) -> ("error out"=w1405:errorcluster, "sessions out"=w1402:refnum<k20>[])  [unwired: 8 in]
        n634 = call <userlib>:"Wait (ms)__ogtk.vi"("error in (no error)"=w1405, "milliseconds to wait"=u32 1500) -> ("error out"=w1404:errorcluster)  [unwired: 8 in, 1 out]
        n635 = Unbundle By Name(w1404) -> ("status"=w1428:bool)
        n636 = Not(x=w1428) -> (.not. x?=w1427:bool)
        n637 = Bundle By Name(cluster=w1429, "System Status.Digitizer"=w1427, "niTClk sessions"=w1402) -> (w1430:T16)
        n638 = property on="Digitizer" class="Bool (strict)"(error in=w1404, "Blinking"=FALSE) -> (error out=w1421:errorcluster)  [unwired: 1 in, 1 out]
        n639 = call <vilib>:"Add State(s) to Queue__JKI_lib_State_Machine.vi"("State(s) in (\"\")"=w1439) -> ("States Out"=w1438:string)  [unwired: 14 in]
      }
      frame "Digitizer: Start" {
        # "send trigger to start acquisition loop"
        # "initilize aquisition"
        # "Template Separator\n(You can make a copy of, or modify, this frame)"
        n640 = Unbundle By Name(w1458) -> ("niTClk sessions"=w1457:refnum<k20>[])
        n641 = call <instrlib>:"niTClk Initiate.vi"("error in (no error)"=w1451, "sessions"=w1457) -> ("error out"=w1453:errorcluster)  [unwired: 8 in, 1 out]
        n642 = Generate User Event(priority (normal)=usereventprio."high priority", user event=w1454, event data cluster=TRUE ("event data"), error in=w1453) -> (error out=w1452:errorcluster)  [unwired: 1 out]
        n643 = call <vilib>:"Add State(s) to Queue__JKI_lib_State_Machine.vi"("State(s) in (\"\")"=w1461) -> ("States Out"=w1460:string)  [unwired: 14 in]
      }
      frame "Digitizer: Abort" {
        # "Template Separator\n(You can make a copy of, or modify, this frame)"
        n644 = call "Digitizer1_FGV.vi"("error in (no error)"=w1465, "Operation (Read)"=enum16{"Write", "Read"}."Read" ("Operation")) -> ("error out"=w1472:errorcluster, "Read data"=w1469:refnum<k15>)  [unwired: 8 in]
        n645 = call "Digitizer2_FGV.vi"("error in (no error)"=w1465, "Operation (Read)"=enum16{"Write", "Read"}."Read" ("Operation")) -> ("error out"=w1468:errorcluster, "Read data"=w1470:refnum<k15>)  [unwired: 8 in]
        n646 = Bundle By Name(cluster=w1462, "SysRunning?"=FALSE ("System Status")) -> (w1463:T16)
        n647 = call <instrlib>:"niScope Abort.vi"("instrument handle"=w1469, "error in"=w1472) -> ("error out"=w1474:errorcluster)  [unwired: 12 in, 1 out]
        n648 = call <instrlib>:"niScope Abort.vi"("instrument handle"=w1470, "error in"=w1468) -> ("error out"=w1473:errorcluster)  [unwired: 12 in, 1 out]
        n649 = Merge Errors(w1474, w1473) -> (w1466:errorcluster)
        n650 = call <vilib>:"Add State(s) to Queue__JKI_lib_State_Machine.vi"("State(s) in (\"\")"=w1477) -> ("States Out"=w1476:string)  [unwired: 14 in]
      }
      frame "Digitizer: checkTemp" {
        w1481 = enum16{"Write", "Read"}."Read" ("Operation")
        # "Template Separator\n(You can make a copy of, or modify, this frame)"
        n651 = call "Digitizer1_FGV.vi"("Operation (Read)"=w1481) -> ("error out"=w1483:errorcluster, "Read data"=w1484:refnum<k15>)  [unwired: 9 in]
        n652 = call "Digitizer2_FGV.vi"("Operation (Read)"=w1481) -> ("error out"=w1479:errorcluster, "Read data"=w1480:refnum<k15>)  [unwired: 9 in]
        n653 = property class="niScope"(reference=w1484, error in=w1483) -> ("Device Temperature"=→"Dig1 Temp":dbl)  [unwired: 2 out]
        n654 = property class="niScope"(reference=w1480, error in=w1479) -> ("Device Temperature"=→"Dig2 Temp":dbl)  [unwired: 2 out]
        n655 = call <vilib>:"Add State(s) to Queue__JKI_lib_State_Machine.vi"("State(s) in (\"\")"=w1489) -> ("States Out"=w1488:string)  [unwired: 14 in]
      }
      frame "Digitizer: Close" {
        # "Close Digitizer"
        n656 = call "Digitizer1_FGV.vi"("error in (no error)"=w1495, "Operation (Read)"=enum16{"Write", "Read"}."Read" ("Operation")) -> ("error out"=w1497:errorcluster, "Read data"=w1501:refnum<k15>)  [unwired: 8 in]
        n657 = call "Digitizer2_FGV.vi"("error in (no error)"=w1495, "Operation (Read)"=enum16{"Write", "Read"}."Read" ("Operation")) -> ("error out"=w1496:errorcluster, "Read data"=w1499:refnum<k15>)  [unwired: 8 in]
        n658 = call <instrlib>:"niScope Close.vi"("instrument handle"=w1501, "error in"=w1497) -> ("error out"=w1494:errorcluster)  [unwired: 13 in]
        n659 = call <instrlib>:"niScope Close.vi"("instrument handle"=w1499, "error in"=w1496) -> ("error out"=w1493:errorcluster)  [unwired: 13 in]
        n660 = Merge Errors(w1494, w1493) -> (w1492:errorcluster)
        n661 = Unbundle By Name(w1492) -> ("status"=w1491:bool)
        n662 = Bundle By Name(cluster=w1502, "System Status.Digitizer"=w1491) -> (w1503:T16)
        n663 = call <vilib>:"Add State(s) to Queue__JKI_lib_State_Machine.vi"("State(s) in (\"\")"=w1505) -> ("States Out"=w1504:string)  [unwired: 14 in]
      }
      frame "---------- LabJack ----------" {
        # "Template Separator\n(You can make a copy of, or modify, this frame)"
        n664 = call <vilib>:"Add State(s) to Queue__JKI_lib_State_Machine.vi"("State(s) in (\"\")"=w1510) -> ("States Out"=w1509:string)  [unwired: 14 in]
      }
      frame "LabJack: checkPedal" {
        # "Template Separator\n(You can make a copy of, or modify, this frame)"
        n665 = Unbundle By Name(w1511) -> ("LJ Pinout.Foot Pedal"=w1515:string)
        n666 = call "LabJack_FGV.vi"("Operation(Read)"=enum16{"Write", "Read"}."Read" ("Operation"), "error in (no error)"=w1513) -> ("error out"=w1517:errorcluster, "Read data"=w1518:i32)  [unwired: 8 in]
        n667 = call "LJM_eReadName.vi"("Handle In"=w1518, "Name"=w1515, "error in"=w1517) -> ("Value"=w1516:dbl, "error out"=w1514:errorcluster)  [unwired: 10 in, 1 out]
        n668 = case shown="1" w1516 {
          tunnel: w1511 -> [w1523 w1526]
          tunnel: [w1523 w1524] -> w1512
          frame 0, Default {
          }
          frame 1 {
            # "If Pedal pressed"
            n669 = Tick Count (ms)() -> (millisecond timer value=w1530:u32)
            n670 = Unbundle By Name(w1526) -> ("Last Trigger"=w1525:u32)
            n671 = Subtract(x=w1530, y=w1525) -> (x-y=w1529:u32)
            n672 = Greater Or Equal?(x=w1529, y=u32 2000) -> (x >= y?=w1527:bool)
            n673 = case shown="True" w1527 {
              tunnel: w1526 -> [w1531 w1532]
              tunnel: w1525 -> [_ _]
              tunnel: [w1531 w1533] -> w1524
              frame False {
              }
              frame True {
                n674 = Tick Count (ms)() -> (millisecond timer value=w1534:u32)
                n675 = Unbundle By Name(w1532) -> ("SysRunning?"=w1535:bool)
                n676 = case shown="True" w1535 {
                  frame False {
                    n677 = property on="StartButton" class="Bool (strict)"("Val(Sgnl)"=TRUE ("Value (Signaling)")) -> ()  [unwired: 2 in, 2 out]
                  }
                  frame True {
                    n678 = property on="StopButton" class="Bool (strict)"("Val(Sgnl)"=TRUE ("Value (Signaling)")) -> ()  [unwired: 2 in, 2 out]
                  }
                }
                n679 = Bundle By Name(cluster=w1532, "Last Trigger"=w1534) -> (w1533:T16)
              }
            }
          }
        }
        n680 = call <vilib>:"Add State(s) to Queue__JKI_lib_State_Machine.vi"("State(s) in (\"\")"=w1522) -> ("States Out"=w1521:string)  [unwired: 14 in]
      }
      frame "LabJack: ZeroV" {
        # "set bias to 0"
        # "Zero APD bias\n(You can make a copy of, or modify, this frame)"
        n681 = Unbundle By Name(w1553) -> ("LJ Pinout.Ch1 Bias"=w1558:string, "LJ Pinout.Ch2 Bias"=w1557:string, "LJ Pinout.Ch3 Bias"=w1556:string)
        n682 = call "V1FGV.vi"("Error In"=w1547, "action (write)"=enum16{"write", "read"}."write" ("action"), "V1 in"=0.0) -> ("Error Out"=w1546:errorcluster, "V1 out"=w1540:dbl)  [unwired: 7 in]
        n683 = Build Array(w1558, w1557, w1556) -> (w1555:string[])
        n684 = local write "Gain 1"(w1540) -> ()
        n685 = call "V2FGV.vi"("Error In"=w1546, "action(write)"=enum16{"write", "read"}."write" ("action"), "V2 in"=0.0) -> ("Error Out"=w1545:errorcluster, "V2 out"=w1539:dbl)  [unwired: 7 in]
        n686 = call "LabJack_FGV.vi"("Operation(Read)"=enum16{"Write", "Read"}."Read" ("Operation"), "error in (no error)"=w1547) -> ("error out"=w1559:errorcluster, "Read data"=w1560:i32)  [unwired: 8 in]
        n687 = local write "Gain 2"(w1539) -> ()
        n688 = call "V3FGV.vi"("Error In"=w1545, "action(write)"=enum16{"write", "read"}."write" ("action"), "V3 in"=0.0) -> ("Error Out"=w1542:errorcluster, "V3 out"=w1538:dbl)  [unwired: 7 in]
        n689 = call "LJM_eWriteNames.vi"("Handle In"=w1560, "aNames"=w1555, "aValuesIn"=dbl[] [0.0, 0.0, 0.0], "error in"=w1559) -> ("error out"=w1543:errorcluster)  [unwired: 9 in, 2 out]
        n690 = local write "Gain 3"(w1538) -> ()
        n691 = Merge Errors(w1542, w1543) -> (w1544:errorcluster)
        n692 = call <vilib>:"Add State(s) to Queue__JKI_lib_State_Machine.vi"("State(s) in (\"\")"=w1564) -> ("States Out"=w1563:string)  [unwired: 14 in]
      }
      frame "LabJack: Open" {
        # "Initialize LabJack T7\nEstablish connection and initialize pins"
        n693 = call "LJ_Open.vi"("error in"=w1573) -> ("error out"=w1570:errorcluster, "Success?"=w1571:bool, "Handle Out"=w1567:i32)  [unwired: 8 in]
        n694 = call "LabJack_FGV.vi"("Operation(Read)"=enum16{"Write", "Read"}."Write" ("Operation"), "error in (no error)"=w1570, "Write data"=w1567) -> ("error out"=w1566:errorcluster)  [unwired: 7 in, 1 out]
        n695 = Bundle By Name(cluster=w1568, "System Status.Labjack"=w1571) -> (w1572:T16)
        n696 = call <vilib>:"Add State(s) to Queue__JKI_lib_State_Machine.vi"("State(s) in (\"\")"=w1575) -> ("States Out"=w1574:string)  [unwired: 14 in]
      }
      frame "LabJack: SetDefaultSub" {
        w1595 = "_EF_ENABLE" ("string")
        # "1. Disable PWM\n2. Set all V to 0\n3. Set 355 relay to open\n4. Set LED to off"
        # "read once to set DIO to input"
        # "set all initila V to 0. Set footpedal to input. Set PWM to low. Set laser relay to open. Set LEDs to yellow."
        # "Set Labjack to correct input and output state and initial values"
        n697 = Unbundle By Name(w1592) -> ("LJ Pinout.355 PWM"=w1597:string, "LJ Pinout.AimingBeam PWM"=w1596:string, "LJ Pinout.Ch1 Bias"=w1604:string, "LJ Pinout.Ch2 Bias"=w1610:string, "LJ Pinout.Ch3 Bias"=w1609:string, "LJ Pinout.Laser Start/Stop"=w1608:string, "LJ Pinout.Red LED"=w1607:string, "LJ Pinout.Green LED"=w1606:string)
        n698 = call "V1FGV.vi"("Error In"=w1585, "action (write)"=enum16{"write", "read"}."write" ("action"), "V1 in"=0.0) -> ("Error Out"=w1586:errorcluster, "V1 out"=w1578:dbl)  [unwired: 7 in]
        n699 = call "LabJack_FGV.vi"("Operation(Read)"=enum16{"Write", "Read"}."Read" ("Operation"), "error in (no error)"=w1585) -> ("error out"=w1600:errorcluster, "Read data"=w1601:i32)  [unwired: 8 in]
        n700 = local write "Gain 1"(w1578) -> ()
        n701 = call "V2FGV.vi"("Error In"=w1586, "action(write)"=enum16{"write", "read"}."write" ("action"), "V2 in"=0.0) -> ("Error Out"=w1582:errorcluster, "V2 out"=w1577:dbl)  [unwired: 7 in]
        n702 = Concatenate Strings(w1597, w1595) -> (w1594:string)
        n703 = Concatenate Strings(w1596, w1595) -> (w1593:string)
        n704 = local write "Gain 2"(w1577) -> ()
        n705 = call "V3FGV.vi"("Error In"=w1582, "action(write)"=enum16{"write", "read"}."write" ("action"), "V3 in"=0.0) -> ("Error Out"=w1579:errorcluster, "V3 out"=w1576:dbl)  [unwired: 7 in]
        n706 = Build Array(w1594, w1593, w1604, w1610, w1609, w1608, w1607, w1606) -> (w1605:string[])
        n707 = Unbundle By Name(w1592) -> ("LJ Pinout.Foot Pedal"=w1591:string)
        n708 = local write "Gain 3"(w1576) -> ()
        n709 = call "LJM_eWriteNames.vi"("Handle In"=w1601, "aNames"=w1605, "aValuesIn"=dbl[] [0.0, 0.0, 0.0, 0.0, 0.0, 0.0, 0.0, 0.0], "error in"=w1600) -> ("Handle Out"=w1599:i32, "error out"=w1598:errorcluster)  [unwired: 9 in, 1 out]
        n710 = call "LJM_eReadName.vi"("Handle In"=w1599, "Name"=w1591, "error in"=w1598) -> ("error out"=w1581:errorcluster)  [unwired: 10 in, 2 out]
        n711 = Merge Errors(w1581, w1579) -> (w1580:errorcluster)
        n712 = call <vilib>:"Add State(s) to Queue__JKI_lib_State_Machine.vi"("State(s) in (\"\")"=w1613) -> ("States Out"=w1612:string)  [unwired: 14 in]
      }
      frame "LabJack: FootPedalConfig" {
        # "Setup footPedal\n(You can make a copy of, or modify, this frame)"
        n713 = call "LabJack_FGV.vi"("Operation(Read)"=enum16{"Write", "Read"}."Read" ("Operation"), "error in (no error)"=w1615) -> ("error out"=w1619:errorcluster, "Read data"=w1620:i32)  [unwired: 8 in]
        n714 = call "LJM_eWriteName.vi"("Handle In"=w1620, "Name"="DIO15", "Value"=1.0, "error in"=w1619) -> ("error out"=w1616:errorcluster)  [unwired: 10 in, 1 out]
        n715 = call <vilib>:"Add State(s) to Queue__JKI_lib_State_Machine.vi"("State(s) in (\"\")"=w1624) -> ("States Out"=w1623:string)  [unwired: 14 in]
      }
      frame "LabJack: SetDefaultAndClose" {
        # "Template Separator\n(You can make a copy of, or modify, this frame)"
        n716 = call <vilib>:"Add State(s) to Queue__JKI_lib_State_Machine.vi"("State(s) in Front (\"\")"="LabJack: SetDefaultSub\nLabJack: Close" ("State(s) in Front (\"\")"), "State(s) in (\"\")"=w1630) -> ("States Out"=w1629:string)  [unwired: 13 in]
      }
      frame "LabJack: Close" {
        # "Close LabJack Refnum"
        n717 = call "LabJack_FGV.vi"("Operation(Read)"=enum16{"Write", "Read"}."Read" ("Operation"), "error in (no error)"=w1636) -> ("error out"=w1631:errorcluster, "Read data"=w1632:i32)  [unwired: 8 in]
        n718 = Bundle By Name(cluster=w1634, "System Status.Labjack"=FALSE ("System Status.Gain Control")) -> (w1637:T16)
        n719 = call "LJM_Close.vi"("error in"=w1631, "Handle"=w1632) -> ("error out"=w1639:errorcluster)  [unwired: 9 in]
        n720 = call <vilib>:"Add State(s) to Queue__JKI_lib_State_Machine.vi"("State(s) in (\"\")"=w1641) -> ("States Out"=w1640:string)  [unwired: 14 in]
      }
      frame "LabJack: Interlock enable/disable" {
        w1650 = i8 0  # int8
        # "Interlock enable/disable\n(Usage: \"LabJack: Interlock enable/disable >> 1|0\")"
        n721 = Fract/Exp String To Number(string=w1651, default (0 dbl)=w1650) -> (number=w1647:i8)  [unwired: 2 in, 1 out]
        n722 = Unbundle By Name(w1649) -> ("LJ Pinout.Interlock"=w1648:string)
        n723 = call "LabJack_FGV.vi"("Operation(Read)"=enum16{"Write", "Read"}."Read" ("Operation")) -> ("Read data"=w1645:i32)  [unwired: 9 in, 1 out]
        n724 = call "LJM_eWriteName.vi"("Handle In"=w1645, "Name"=w1648, "Value"=w1647, "error in"=w1646) -> ("error out"=w1643:errorcluster)  [unwired: 10 in, 1 out]
        n725 = call <vilib>:"Add State(s) to Queue__JKI_lib_State_Machine.vi"("State(s) in (\"\")"=w1653) -> ("States Out"=w1652:string)  [unwired: 14 in]
      }
      frame "LabJack: 355_PWM_Config" {
        w1655 = 0.0 ("element")
        w1675 = "DIO_EF_CLOCK1_ENABLE"
        # "Config PWM frequency"
        n726 = Unbundle By Name(w1667) -> ("355 PWM setting.DIO_EF_CLOCK1_DIVISOR"=w1666:i16, "355 PWM setting.DIO_EF_CLOCK1_ROLL_VALUE"=w1665:i32, "355 PWM setting.DIO#_EF_INDEX"=w1662:i16, "355 PWM setting.DIO#_EF_OPTIONS"=w1661:i16, "355 PWM setting.DIO#_EF_CONFIG_A"=w1660:i32)
        n727 = Unbundle By Name(w1667) -> ("LJ Pinout.355 PWM"=w1674:string)
        n728 = Concatenate Strings(w1674, "_EF_ENABLE" ("string")) -> (w1670:string)
        n729 = Concatenate Strings(w1674, "_EF_INDEX") -> (w1673:string)
        n730 = Concatenate Strings(w1674, "_EF_OPTIONS") -> (w1672:string)
        n731 = Concatenate Strings(w1674, "_EF_CONFIG_A") -> (w1671:string)
        n732 = call "LabJack_FGV.vi"("Operation(Read)"=enum16{"Write", "Read"}."Read" ("Operation")) -> ("Read data"=w1668:i32)  [unwired: 9 in, 1 out]
        n733 = Build Array(w1655, w1655, w1666, w1665, 1.0 ("element"), 0.0 ("element"), w1662, w1661, w1660) -> (w1659:dbl[])
        n734 = Build Array("DIO_EF_CLOCK0_ENABLE", w1675, "DIO_EF_CLOCK1_DIVISOR", "DIO_EF_CLOCK1_ROLL_VALUE", w1675, w1670, w1673, w1672, w1671) -> (w1669:string[])
        n735 = call "LJM_eWriteNames.vi"("Handle In"=w1668, "aNames"=w1669, "aValuesIn"=w1659, "error in"=w1657) -> ("error out"=w1658:errorcluster)  [unwired: 9 in, 2 out]
        n736 = call <vilib>:"Add State(s) to Queue__JKI_lib_State_Machine.vi"("State(s) in (\"\")"=w1684) -> ("States Out"=w1683:string)  [unwired: 14 in]
      }
      frame "LabJack: AB_PWM_Config" {
        w1686 = 0.0 ("element")
        w1706 = "DIO_EF_CLOCK2_ENABLE"
        # "Config PWM frequency"
        n737 = Unbundle By Name(w1698) -> ("LJ Pinout.AimingBeam PWM"=w1705:string)
        n738 = Unbundle By Name(w1698) -> ("AB PWM setting.DIO_EF_CLOCK1_DIVISOR"=w1697:i16, "AB PWM setting.DIO_EF_CLOCK1_ROLL_VALUE"=w1696:i32, "AB PWM setting.DIO#_EF_INDEX"=w1693:i16, "AB PWM setting.DIO#_EF_OPTIONS"=w1692:i16, "AB PWM setting.DIO#_EF_CONFIG_A"=w1691:i32)
        n739 = Concatenate Strings(w1705, "_EF_ENABLE" ("string")) -> (w1701:string)
        n740 = Concatenate Strings(w1705, "_EF_INDEX") -> (w1704:string)
        n741 = Concatenate Strings(w1705, "_EF_OPTIONS") -> (w1703:string)
        n742 = Concatenate Strings(w1705, "_EF_CONFIG_A") -> (w1702:string)
        n743 = call "LabJack_FGV.vi"("Operation(Read)"=enum16{"Write", "Read"}."Read" ("Operation")) -> ("Read data"=w1699:i32)  [unwired: 9 in, 1 out]
        n744 = Build Array(w1686, w1686, w1697, w1696, 1.0 ("element"), 0.0 ("element"), w1693, w1692, w1691) -> (w1690:dbl[])
        n745 = Build Array("DIO_EF_CLOCK0_ENABLE", w1706, "DIO_EF_CLOCK2_DIVISOR", "DIO_EF_CLOCK2_ROLL_VALUE", w1706, w1701, w1704, w1703, w1702) -> (w1700:string[])
        n746 = call "LJM_eWriteNames.vi"("Handle In"=w1699, "aNames"=w1700, "aValuesIn"=w1690, "error in"=w1688) -> ("error out"=w1689:errorcluster)  [unwired: 9 in, 2 out]
        n747 = call <vilib>:"Add State(s) to Queue__JKI_lib_State_Machine.vi"("State(s) in (\"\")"=w1715) -> ("States Out"=w1714:string)  [unwired: 14 in]
      }
      frame "LabJack: 355_PWM_Start" {
        # "Template Separator\n(You can make a copy of, or modify, this frame)"
        n748 = Unbundle By Name(w1723) -> ("LJ Pinout.355 PWM"=w1722:string)
        n749 = call "LabJack_FGV.vi"("Operation(Read)"=enum16{"Write", "Read"}."Read" ("Operation"), "error in (no error)"=w1717) -> ("error out"=w1724:errorcluster, "Read data"=w1725:i32)  [unwired: 8 in]
        n750 = Concatenate Strings(w1722, "_EF_ENABLE" ("string")) -> (w1720:string)
        n751 = call "LJM_eWriteName.vi"("Handle In"=w1725, "Name"=w1720, "Value"=1.0, "error in"=w1724) -> ("error out"=w1718:errorcluster)  [unwired: 10 in, 1 out]
        n752 = call <vilib>:"Add State(s) to Queue__JKI_lib_State_Machine.vi"("State(s) in (\"\")"=w1728) -> ("States Out"=w1727:string)  [unwired: 14 in]
      }
      frame "LabJack: AB_PWM_Start" {
        # "Template Separator\n(You can make a copy of, or modify, this frame)"
        n753 = Unbundle By Name(w1736) -> ("LJ Pinout.AimingBeam PWM"=w1735:string)
        n754 = call "LabJack_FGV.vi"("Operation(Read)"=enum16{"Write", "Read"}."Read" ("Operation"), "error in (no error)"=w1730) -> ("error out"=w1737:errorcluster, "Read data"=w1738:i32)  [unwired: 8 in]
        n755 = Concatenate Strings(w1735, "_EF_ENABLE" ("string")) -> (w1733:string)
        n756 = call "LJM_eWriteName.vi"("Handle In"=w1738, "Name"=w1733, "Value"=1.0, "error in"=w1737) -> ("error out"=w1731:errorcluster)  [unwired: 10 in, 1 out]
        n757 = call <vilib>:"Add State(s) to Queue__JKI_lib_State_Machine.vi"("State(s) in (\"\")"=w1741) -> ("States Out"=w1740:string)  [unwired: 14 in]
      }
      frame "LabJack: 355_PWM_Stop" {
        # "Template Separator\n(You can make a copy of, or modify, this frame)"
        n758 = Unbundle By Name(w1747) -> ("LJ Pinout.355 PWM"=w1751:string)
        n759 = call "LabJack_FGV.vi"("Operation(Read)"=enum16{"Write", "Read"}."Read" ("Operation"), "error in (no error)"=w1745) -> ("error out"=w1752:errorcluster, "Read data"=w1743:i32)  [unwired: 8 in]
        n760 = Concatenate Strings(w1751, "_EF_ENABLE" ("string")) -> (w1749:string)
        n761 = call "LJM_eWriteName.vi"("Handle In"=w1743, "Name"=w1749, "Value"=0.0, "error in"=w1752) -> ("error out"=w1746:errorcluster)  [unwired: 10 in, 1 out]
        n762 = local write "355nm Laser toggle"(FALSE ("355nm Laser toggle")) -> ()
        n763 = call <vilib>:"Add State(s) to Queue__JKI_lib_State_Machine.vi"("State(s) in (\"\")"=w1755) -> ("States Out"=w1754:string)  [unwired: 14 in]
      }
      frame "LabJack: AB_PWM_Stop" {
        # "Template Separator\n(You can make a copy of, or modify, this frame)"
        n764 = Unbundle By Name(w1760) -> ("LJ Pinout.AimingBeam PWM"=w1764:string)
        n765 = call "LabJack_FGV.vi"("Operation(Read)"=enum16{"Write", "Read"}."Read" ("Operation"), "error in (no error)"=w1758) -> ("error out"=w1765:errorcluster, "Read data"=w1766:i32)  [unwired: 8 in]
        n766 = Concatenate Strings(w1764, "_EF_ENABLE" ("string")) -> (w1762:string)
        n767 = call "LJM_eWriteName.vi"("Handle In"=w1766, "Name"=w1762, "Value"=0.0, "error in"=w1765) -> ("error out"=w1759:errorcluster)  [unwired: 10 in, 1 out]
        n768 = local write "Aiming beam toggle"(FALSE ("Aiming beam toggle")) -> ()
        n769 = call <vilib>:"Add State(s) to Queue__JKI_lib_State_Machine.vi"("State(s) in (\"\")"=w1769) -> ("States Out"=w1768:string)  [unwired: 14 in]
      }
      frame "---------- LED ----------" {
        # "Template Separator\n(You can make a copy of, or modify, this frame)"
        n770 = call <vilib>:"Add State(s) to Queue__JKI_lib_State_Machine.vi"("State(s) in (\"\")"=w1774) -> ("States Out"=w1773:string)  [unwired: 14 in]
      }
      frame "LED: OpenVIRef" {
        w1780 = path "C:/Users/IntuitiveA/Desktop/V6 APD LV/SubVI/LEDBreath.vi"  # vi path
        # "Template Separator\n(You can make a copy of, or modify, this frame)"
        n771 = Open VI Reference(vi path=w1780, error in (no error)=w1775) -> (vi reference=w1777:refnum<vi>, error out=w1776:errorcluster)  [unwired: 4 in]
        n772 = Bundle By Name(cluster=w1778, "LED vi reference"=w1777) -> (w1779:T16)
        n773 = call <vilib>:"Add State(s) to Queue__JKI_lib_State_Machine.vi"("State(s) in (\"\")"=w1783) -> ("States Out"=w1782:string)  [unwired: 14 in]
      }
      frame "LED: CloseVIRef" {
        # "Template Separator\n(You can make a copy of, or modify, this frame)"
        n774 = Unbundle By Name(w1784) -> ("LED vi reference"=w1785:refnum<vi>)
        n775 = Close Reference(reference=w1785, error in (no error)=w1787) -> (error out=w1786:errorcluster)
        n776 = call <vilib>:"Add State(s) to Queue__JKI_lib_State_Machine.vi"("State(s) in (\"\")"=w1790) -> ("States Out"=w1789:string)  [unwired: 14 in]
      }
      frame "LED: Breath" {
        # "Breath system LED\n(LED: Breath >> True/False)"
        n777 = Unbundle By Name(w1795) -> ("LED vi reference"=w1794:refnum<vi>)
        n778 = case shown="\"False\", Default" w1791 {
          tunnel: w1794 -> [w1803 w1807]
          tunnel: [w1801 w1805] -> w1793
          tunnel: w1792 -> [w1802 w1804]
          frame "False", Default {
            n779 = invoke class="VI" method="Ctrl Val.Set"(reference=w1803, error in=w1802, "Control Name"="Stop", "Value"=TRUE) -> (error out=w1801:errorcluster)  [unwired: 1 in, 4 out]
          }
          frame "True" {
            n780 = invoke class="VI" method="Run VI"(reference=w1807, error in=w1804, "Wait until done"=FALSE ("Wait Until Done"), "Auto Dispose Ref"=FALSE ("Auto Dispose Reference")) -> (error out=w1805:errorcluster)  [unwired: 1 in, 4 out]
          }
        }
        n781 = call <vilib>:"Add State(s) to Queue__JKI_lib_State_Machine.vi"("State(s) in (\"\")"=w1798) -> ("States Out"=w1797:string)  [unwired: 14 in]
      }
      frame "LED: Off" {
        # "set LED to red"
        # "Template Separator\n(You can make a copy of, or modify, this frame)"
        n782 = Unbundle By Name(w1811) -> ("LJ Pinout.Red LED"=w1810:string, "LJ Pinout.Green LED"=w1809:string)
        n783 = call "LabJack_FGV.vi"("Operation(Read)"=enum16{"Write", "Read"}."Read" ("Operation"), "error in (no error)"=w1812) -> ("error out"=w1819:errorcluster, "Read data"=w1818:i32)  [unwired: 8 in]
        n784 = call "LJM_eWriteName.vi"("Handle In"=w1818, "Name"=w1810, "Value"=0.0, "error in"=w1819) -> ("Handle Out"=w1816:i32, "error out"=w1815:errorcluster)  [unwired: 10 in]
        n785 = call "LJM_eWriteName.vi"("Handle In"=w1816, "Name"=w1809, "Value"=0.0, "error in"=w1815) -> ("error out"=w1813:errorcluster)  [unwired: 10 in, 1 out]
        n786 = call <vilib>:"Add State(s) to Queue__JKI_lib_State_Machine.vi"("State(s) in (\"\")"=w1823) -> ("States Out"=w1822:string)  [unwired: 14 in]
      }
      frame "LED: Red" {
        # "set LED to red"
        # "Template Separator\n(You can make a copy of, or modify, this frame)"
        n787 = Unbundle By Name(w1826) -> ("LJ Pinout.Red LED"=w1825:string, "LJ Pinout.Green LED"=w1824:string)
        n788 = call "LabJack_FGV.vi"("Operation(Read)"=enum16{"Write", "Read"}."Read" ("Operation"), "error in (no error)"=w1827) -> ("error out"=w1834:errorcluster, "Read data"=w1833:i32)  [unwired: 8 in]
        n789 = call "LJM_eWriteName.vi"("Handle In"=w1833, "Name"=w1825, "Value"=9.0, "error in"=w1834) -> ("Handle Out"=w1831:i32, "error out"=w1830:errorcluster)  [unwired: 10 in]
        n790 = call "LJM_eWriteName.vi"("Handle In"=w1831, "Name"=w1824, "Value"=0.0, "error in"=w1830) -> ("error out"=w1828:errorcluster)  [unwired: 10 in, 1 out]
        n791 = call <vilib>:"Add State(s) to Queue__JKI_lib_State_Machine.vi"("State(s) in (\"\")"=w1838) -> ("States Out"=w1837:string)  [unwired: 14 in]
      }
      frame "LED: Green" {
        # "set LED to green"
        # "Template Separator\n(You can make a copy of, or modify, this frame)"
        n792 = Unbundle By Name(w1842) -> ("LJ Pinout.Red LED"=w1840:string, "LJ Pinout.Green LED"=w1841:string)
        n793 = call "LabJack_FGV.vi"("Operation(Read)"=enum16{"Write", "Read"}."Read" ("Operation"), "error in (no error)"=w1844) -> ("error out"=w1850:errorcluster, "Read data"=w1849:i32)  [unwired: 8 in]
        n794 = call "LJM_eWriteName.vi"("Handle In"=w1849, "Name"=w1840, "Value"=0.0, "error in"=w1850) -> ("Handle Out"=w1847:i32, "error out"=w1846:errorcluster)  [unwired: 10 in]
        n795 = call "LJM_eWriteName.vi"("Handle In"=w1847, "Name"=w1841, "Value"=9.0, "error in"=w1846) -> ("error out"=w1843:errorcluster)  [unwired: 10 in, 1 out]
        n796 = call <vilib>:"Add State(s) to Queue__JKI_lib_State_Machine.vi"("State(s) in (\"\")"=w1853) -> ("States Out"=w1852:string)  [unwired: 14 in]
      }
      frame "LED: Yellow" {
        # "set LED to yellow"
        # "set LED to yellow\n(You can make a copy of, or modify, this frame)"
        n797 = Unbundle By Name(w1857) -> ("LJ Pinout.Red LED"=w1855:string, "LJ Pinout.Green LED"=w1856:string)
        n798 = call "LabJack_FGV.vi"("Operation(Read)"=enum16{"Write", "Read"}."Read" ("Operation"), "error in (no error)"=w1859) -> ("error out"=w1865:errorcluster, "Read data"=w1864:i32)  [unwired: 8 in]
        n799 = call "LJM_eWriteName.vi"("Handle In"=w1864, "Name"=w1855, "Value"=9.0, "error in"=w1865) -> ("Handle Out"=w1862:i32, "error out"=w1861:errorcluster)  [unwired: 10 in]
        n800 = call "LJM_eWriteName.vi"("Handle In"=w1862, "Name"=w1856, "Value"=9.0, "error in"=w1861) -> ("error out"=w1858:errorcluster)  [unwired: 10 in, 1 out]
        n801 = call <vilib>:"Add State(s) to Queue__JKI_lib_State_Machine.vi"("State(s) in (\"\")"=w1868) -> ("States Out"=w1867:string)  [unwired: 14 in]
      }
      frame "---------- Queue ----------" {
        # "Template Separator\n(You can make a copy of, or modify, this frame)"
        n802 = call <vilib>:"Add State(s) to Queue__JKI_lib_State_Machine.vi"("State(s) in (\"\")"=w1873) -> ("States Out"=w1872:string)  [unwired: 14 in]
      }
      frame "Queue: Create" {
        # "Template Separator\n(You can make a copy of, or modify, this frame)"
        n803 = call <vilib>:"Add State(s) to Queue__JKI_lib_State_Machine.vi"("State(s) in (\"\")"=w1878) -> ("States Out"=w1877:string)  [unwired: 14 in]
      }
      frame "Queue: Flash" {
        # "Clear queue contnet\n(clear queue content by flash it)"
        n804 = Flush Queue(queue=w1882, error in (no error)=w1881) -> (error out=w1880:errorcluster)  [unwired: 2 out]
        n805 = Flush Queue(queue=w1883, error in (no error)=w1880) -> (error out=w1879:errorcluster)  [unwired: 2 out]
        n806 = call <vilib>:"Add State(s) to Queue__JKI_lib_State_Machine.vi"("State(s) in (\"\")"=w1887) -> ("States Out"=w1886:string)  [unwired: 14 in]
      }
      frame "Queue: Destory" {
        # "Destory Data Queue\nDistory data queue ref so the aquisition loop stop"
        n807 = Release Queue(queue=w1893, error in (no error)=w1889) -> (error out=w1896:errorcluster)  [unwired: 1 in, 2 out]
        n808 = Release Queue(queue=w1892, error in (no error)=w1889) -> (error out=w1895:errorcluster)  [unwired: 1 in, 2 out]
        n809 = Release Queue(queue=w1890, error in (no error)=w1889) -> (error out=w1888:errorcluster)  [unwired: 1 in, 2 out]
        n810 = Merge Errors(w1896, w1895, w1888) -> (w1894:errorcluster)
        n811 = call <vilib>:"Simple Error Handler.vi"("error in (no error)"=w1894) -> ()  [unwired: 4 in, 5 out]
        n812 = call <vilib>:"Add State(s) to Queue__JKI_lib_State_Machine.vi"("State(s) in (\"\")"=w1899) -> ("States Out"=w1898:string)  [unwired: 14 in]
      }
      frame "---------- Run ----------" {
        # "Template Separator\n(You can make a copy of, or modify, this frame)"
        n813 = call <vilib>:"Add State(s) to Queue__JKI_lib_State_Machine.vi"("State(s) in (\"\")"=w1904) -> ("States Out"=w1903:string)  [unwired: 14 in]
      }
      frame "Run: CaliIncrement" {
        # "Increment Calibration #\n(You can make a copy of, or modify, this frame)"
        n814 = Unbundle By Name(w1906) -> ("IDs.Cali ID"=w1908:i8)
        n815 = Increment(x=w1908) -> (x+1=w1905:i8)
        n816 = Bundle By Name(cluster=w1906, "IDs.Cali ID"=w1905) -> (w1907:T16)
        n817 = call <vilib>:"Add State(s) to Queue__JKI_lib_State_Machine.vi"("State(s) in (\"\")"=w1912) -> ("States Out"=w1911:string)  [unwired: 14 in]
      }
      frame "Run: BGIncrement" {
        # "Increment BG #\n(You can make a copy of, or modify, this frame)"
        n818 = Unbundle By Name(w1913) -> ("IDs.BG ID"=w1916:i8)
        n819 = Increment(x=w1916) -> (x+1=w1915:i8)
        n820 = Bundle By Name(cluster=w1913, "IDs.BG ID"=w1915) -> (w1914:T16)
        n821 = call <vilib>:"Add State(s) to Queue__JKI_lib_State_Machine.vi"("State(s) in (\"\")"=w1920) -> ("States Out"=w1919:string)  [unwired: 14 in]
      }
      frame "Run: Increment" {
        # "Increase Run# by 1"
        n822 = Unbundle By Name(w1923) -> ("IDs.RunID"=w1925:i8)
        n823 = Increment(x=w1925) -> (x+1=w1922:i8)
        n824 = Bundle By Name(cluster=w1923, "IDs.RunID"=w1922) -> (w1924:T16)
        n825 = call <vilib>:"Add State(s) to Queue__JKI_lib_State_Machine.vi"("State(s) in (\"\")"=w1928) -> ("States Out"=w1927:string)  [unwired: 14 in]
      }
      frame "Run: Decrement" {
        # "Increase Run# by 1"
        n826 = Unbundle By Name(w1931) -> ("IDs.RunID"=w1933:i8)
        n827 = Decrement(x=w1933) -> (x-1=w1930:i8)
        n828 = Bundle By Name(cluster=w1931, "IDs.RunID"=w1930) -> (w1932:T16)
        n829 = call <vilib>:"Add State(s) to Queue__JKI_lib_State_Machine.vi"("State(s) in (\"\")"=w1936) -> ("States Out"=w1935:string)  [unwired: 14 in]
      }
      frame "---------- SysConfig ----------" {
        # "Template Separator\n(You can make a copy of, or modify, this frame)"
        n830 = call <vilib>:"Add State(s) to Queue__JKI_lib_State_Machine.vi"("State(s) in (\"\")"=w1941) -> ("States Out"=w1940:string)  [unwired: 14 in]
      }
      frame "SysConfig: Load Sys Config" {
        # "Load System config"
        # "Load system configuration\n(Load both hardware and DAQ config)"
        n831 = call "LoadSysConfig.vi"("Error In"=w1944, "Enum"=enum16{"LastUse", "Default"}."LastUse") -> ("Error Out"=w1943:errorcluster, "SysConfigCluster"=w1946:T3)  [unwired: 8 in]
        "SysConfigCluster" <- w1946
        n832 = Bundle By Name(cluster=w1947, "SysConfigCluster"=w1946) -> (w1948:T16)
        n833 = call <vilib>:"Add State(s) to Queue__JKI_lib_State_Machine.vi"("State(s) in (\"\")"=w1950) -> ("States Out"=w1949:string)  [unwired: 14 in]
      }
      frame "SysConfig: Load Digitizer Setting" {
        w1957 = enum16{"Write", "Read"}."Write" ("Operation")
        # "Load DAQ config\nSave to FGV"
        # "Template Separator\n(You can make a copy of, or modify, this frame)"
        n834 = call <userlib>:"Current VIs Parent Directory__ogtk.vi"() -> ("Parent Directory (+ Relative)"=w1964:path)  [unwired: 5 in]
        n835 = Build Path(base path=w1964, name or relative path="SubVI\\DigitizerConfiguration\\V6_Scope_last_use.config") -> (appended path=w1965:path)
        n836 = call "ReadDigitizerConfig(SubVI).vi"("error in (no error)"=w1962, "appended path"=w1965) -> ("error out"=w1956:errorcluster, "FLImDAQ"=w1954:T5)  [unwired: 8 in]
        n837 = call "FLImDAQ_FGV.vi"(6:w1957, "error in (no error)"=w1956, "Write data"=w1954) -> ("error out"=w1960:errorcluster)  [unwired: 7 in, 1 out]
        n838 = Bundle By Name(cluster=w1952, "FLImDAQ"=w1954) -> (w1953:T16)
        n839 = Unbundle By Name(w1954) -> ("Digitizer 1"=w1958:refnum<k15>, "Digitizer 2"=w1959:refnum<k15>)
        n840 = call "Digitizer1_FGV.vi"("error in (no error)"=w1960, "Operation (Read)"=w1957, "Write data"=w1958) -> ("error out"=w1961:errorcluster)  [unwired: 7 in, 1 out]
        n841 = call "Digitizer2_FGV.vi"("error in (no error)"=w1961, "Operation (Read)"=w1957, "Write data"=w1959) -> ("error out"=w1955:errorcluster)  [unwired: 7 in, 1 out]
        n842 = call <vilib>:"Add State(s) to Queue__JKI_lib_State_Machine.vi"("State(s) in (\"\")"=w1967) -> ("States Out"=w1966:string)  [unwired: 14 in]
      }
      frame "SysConfig: Load LJ Pinout" {
        # "Template Separator\n(You can make a copy of, or modify, this frame)"
        n843 = call <userlib>:"Current VIs Parent Directory__ogtk.vi"() -> ("Parent Directory (+ Relative)"=w1981:path)  [unwired: 5 in]
        n844 = Build Path(base path=w1981, name or relative path="SubVI\\LabJack\\LJ_pin_setting.config") -> (appended path=w1979:path)
        n845 = call "ReadLabjackConfig(SubVI).vi"("error in (no error)"=w1977, "appended path"=w1979) -> ("error out"=w1978:errorcluster, "Utility"=w1975:T4)  [unwired: 8 in]
        n846 = Unbundle By Name(w1975) -> ("Ch1 Bias"=w1974:string, "Ch2 Bias"=w1973:string, "Ch3 Bias"=w1972:string, "Red LED"=w1969:string, "Green LED"=w1968:string)
        n847 = global write "GlobalVariables.vi" "LED Green pin"(w1968) -> ()
        n848 = global write "GlobalVariables.vi" "LED Red pin"(w1969) -> ()
        n849 = global write "GlobalVariables.vi" "Ch1 LJ pin"(w1974) -> ()
        n850 = global write "GlobalVariables.vi" "Ch2 LJ pin"(w1973) -> ()
        n851 = global write "GlobalVariables.vi" "Ch3 LJ pin"(w1972) -> ()
        n852 = Bundle By Name(cluster=w1970, "LJ Pinout"=w1975) -> (w1976:T16)
        n853 = call <vilib>:"Add State(s) to Queue__JKI_lib_State_Machine.vi"("State(s) in (\"\")"=w1983) -> ("States Out"=w1982:string)  [unwired: 14 in]
      }
      frame "SysConfig: Load 355 PWM" {
        # "Template Separator\n(You can make a copy of, or modify, this frame)"
        n854 = call <userlib>:"Current VIs Parent Directory__ogtk.vi"() -> ("Parent Directory (+ Relative)"=w2001:path)  [unwired: 5 in]
        n855 = Build Path(base path=w2001, name or relative path="SubVI\\LabJack\\PWM_setting_355.config") -> (appended path=w1999:path)
        n856 = call "ReadPWMConfig(SubVI).vi"("error in (no error)"=w1996, "appended path"=w1999) -> ("error out"=w1997:errorcluster, "PWM Setting"=w1995:T27)  [unwired: 8 in]
        n857 = Unbundle By Name(w1995) -> ("DIO_EF_CLOCK1_DIVISOR"=w1992:i16, "DIO_EF_CLOCK1_ROLL_VALUE"=w1991:i32)
        n858 = Multiply(x=w1992, y=w1991) -> (x*y=w1993:i32)
        n859 = Bundle By Name(cluster=w1998, "355 PWM setting"=w1995) -> (w1985:T16)
        n860 = Divide(x=80000000.0, y=w1993) -> (x/y=w1990:dbl)
        n861 = Number To Decimal String(number=w1990) -> (decimal integer string=w1989:string)  [unwired: 1 in]
        n862 = Concatenate Strings("355nm " ("string"), w1989, "Hz" ("string")) -> (w1987:string)
        n863 = property on="355nm Laser toggle" class="Bool (strict)"("Caption.Text"=w1987) -> ()  [unwired: 2 in, 2 out]
        n864 = call <vilib>:"Add State(s) to Queue__JKI_lib_State_Machine.vi"("State(s) in (\"\")"=w2003) -> ("States Out"=w2002:string)  [unwired: 14 in]
      }
      frame "SysConfig: Load AB PWM" {
        # "Template Separator\n(You can make a copy of, or modify, this frame)"
        n865 = call <userlib>:"Current VIs Parent Directory__ogtk.vi"() -> ("Parent Directory (+ Relative)"=w2022:path)  [unwired: 5 in]
        n866 = Build Path(base path=w2022, name or relative path="SubVI\\LabJack\\PWM_setting_AB.config") -> (appended path=w2020:path)
        n867 = call "ReadPWMConfig(SubVI).vi"("error in (no error)"=w2017, "appended path"=w2020) -> ("error out"=w2018:errorcluster, "PWM Setting"=w2016:T27)  [unwired: 8 in]
        n868 = Unbundle By Name(w2016) -> ("DIO_EF_CLOCK1_DIVISOR"=w2013:i16, "DIO_EF_CLOCK1_ROLL_VALUE"=w2012:i32)
        n869 = Multiply(x=w2013, y=w2012) -> (x*y=w2014:i32)
        n870 = Bundle By Name(cluster=w2006, "AB PWM setting"=w2016) -> (w2019:T16)
        n871 = Divide(x=80000000.0, y=w2014) -> (x/y=w2011:dbl)
        n872 = Number To Decimal String(number=w2011, width (-)=i16 2) -> (decimal integer string=w2010:string)
        n873 = Concatenate Strings("445nm " ("string"), w2010, "Hz " ("string")) -> (w2008:string)
        n874 = property on="Aiming beam toggle" class="Bool (strict)"("Caption.Text"=w2008) -> ()  [unwired: 2 in, 2 out]
        n875 = call <vilib>:"Add State(s) to Queue__JKI_lib_State_Machine.vi"("State(s) in (\"\")"=w2024) -> ("States Out"=w2023:string)  [unwired: 14 in]
      }
      frame "SysConfig: Load AB setting" {
        # "Template Separator\n(You can make a copy of, or modify, this frame)"
        n876 = call "readAimingBeamSetting.vi"("error in (no error)"=w2026) -> ("error out"=w2027:errorcluster, "Aiming Beam Setting"=w2028:T28)  [unwired: 9 in]
        n877 = Bundle By Name(cluster=w2029, "AB Cluster"=w2028) -> (w2030:T16)
        n878 = call <vilib>:"Add State(s) to Queue__JKI_lib_State_Machine.vi"("State(s) in (\"\")"=w2032) -> ("States Out"=w2031:string)  [unwired: 14 in]
      }
      frame "---------- SystemStatus ----------" {
        # "Template Separator\n(You can make a copy of, or modify, this frame)"
        n879 = call <vilib>:"Add State(s) to Queue__JKI_lib_State_Machine.vi"("State(s) in (\"\")"=w2037) -> ("States Out"=w2036:string)  [unwired: 14 in]
      }
      frame "SystemStatus: SlowSysStatusMacro" {
        # "store system check time"
        # "Template Separator\n(You can make a copy of, or modify, this frame)"
        n880 = Tick Count (ms)() -> (millisecond timer value=w2040:u32)
        n881 = Bundle By Name(cluster=w2038, "SlowTimer"=w2040) -> (w2039:T16)
        n882 = call <vilib>:"Add State(s) to Queue__JKI_lib_State_Machine.vi"("State(s) in Front (\"\")"="Digitizer: checkTemp\nTCP: CheckConnection" ("State(s) in Front (\"\")"), "State(s) in (\"\")"=w2045) -> ("States Out"=w2044:string)  [unwired: 13 in]
      }
      frame "SystemStatus: FastSysStatusMacro" {
        # "store system check time"
        # "Template Separator\n(You can make a copy of, or modify, this frame)"
        n883 = Tick Count (ms)() -> (millisecond timer value=w2048:u32)
        n884 = Bundle By Name(cluster=w2046, "FastTimer"=w2048) -> (w2047:T16)
        n885 = call <vilib>:"Add State(s) to Queue__JKI_lib_State_Machine.vi"("State(s) in Front (\"\")"="355 Laser: CheckPWMStatus\nAimingBeam: GetPWMStatus\n" ("State(s) in Front (\"\")"), "State(s) in (\"\")"=w2053) -> ("States Out"=w2052:string)  [unwired: 13 in]
      }
      frame "---------- TCP ----------" {
        # "Template Separator\n(You can make a copy of, or modify, this frame)"
        n886 = call <vilib>:"Add State(s) to Queue__JKI_lib_State_Machine.vi"("State(s) in (\"\")"=w2058) -> ("States Out"=w2057:string)  [unwired: 14 in]
      }
      frame "TCP: Initialize" {
        # "Initialize TCP connection to aimging beam computer\n(You can make a copy of, or modify, this frame)"
        n887 = call <vilib>:"TCP Listen.vi"("error in (no error)"=w2082, "timeout ms (wait forever: -1)"=1000, "port"=u16 2100, "service name"="RTLT") -> ("error out"=w2077:errorcluster, "connection ID"=w2078:refnum<k5>, "listener ID"=w2059:refnum<k5>)  [unwired: 3 in, 2 out]
        n888 = TCP Read(connection ID=w2078, bytes to read=512, error in (no error)=w2077, 7:T15."CRLF" ("mode (standard)"), 9:10000 ("timeout ms (25000)")) -> (connection ID out=w2067:refnum<k5>, data out=w2074:string, error out=w2068:errorcluster)
        n889 = Concatenate Strings("alive" ("string"), "\r\n") -> (w2071:string)
        n890 = Equal?(x=w2074, y=w2071) -> (x = y?=w2069:bool)
        n891 = case shown="True" w2069 {
          tunnel: w2068 -> [w2086 w2107]
          tunnel: w2067 -> [_ w2101]
          tunnel: [w2087 w2105] -> w2066
          tunnel: w2064 -> [w2093 _]
          tunnel: [w2089 0] -> w2063
          tunnel: [w2088 ""] -> w2061
          tunnel: [FALSE TRUE] -> w2060
          frame False {
            # "if unsuccessful and count <10, increament count \nand try again"
            n892 = Unbundle By Name(w2093) -> ("TCP attempt count"=w2090:i32)
            n893 = Less?(x=w2090, y=1) -> (x < y?=w2091:bool)
            n894 = case shown="True" w2091 {
              tunnel: w2090 -> [w2096 w2100]
              tunnel: [w2096 w2099] -> w2089
              tunnel: ["" "TCP: Initialize"] -> w2088
              tunnel: [errorcluster {"status"=TRUE, "code"=5001, "source"="TCP/IP"} ("error in (no error)") errorcluster {"status"=FALSE, "code"=5001, "source"=""} ("error in (no error)")] -> w2087
              tunnel: w2086 -> [_ _]
              frame False {
                # "send error and shut down"
              }
              frame True {
                # "try again until 10th"
                n895 = Increment(x=w2100) -> (x+1=w2099:i32)
              }
            }
          }
          frame True {
            # "if connection is successful\nwrite TCP FVG"
            n896 = call "TcpIDFGV.vi"("Error In"=w2107, "action"=enum16{"write", "read"}."write", "connection ID in"=w2101) -> ("Error Out"=w2105:errorcluster)  [unwired: 7 in, 1 out]
          }
        }
        n897 = Bundle By Name(cluster=w2064, "TCP attempt count"=w2063, "System Status.TCP/IP"=w2060, "listener ID"=w2059) -> (w2065:T16)
        n898 = global write "GlobalVariables.vi" "TCP connected?"(w2060) -> ()
        n899 = call <vilib>:"Add State(s) to Queue__JKI_lib_State_Machine.vi"("State(s) in Front (\"\")"=w2061, "State(s) in (\"\")"=w2084) -> ("States Out"=w2083:string)  [unwired: 13 in]
      }
      frame "TCP: SyncTime" {
        # "Template Separator\n(You can make a copy of, or modify, this frame)"
        n900 = call "TcpIDFGV.vi"("Error In"=w2112, "action"=enum16{"write", "read"}."read") -> ("Error Out"=w2111:errorcluster, "connection ID out"=w2109:refnum<k5>)  [unwired: 8 in]
        n901 = call <userlib>:"Tick Count (ms)__ogtk.vi"("error in (no error)"=w2111) -> ("error out"=w2110:errorcluster, "millisecond timer value"=w2108:u32)  [unwired: 9 in]
        n902 = while {
          tunnel: w2110 -> [w2136]
          tunnel: w2109 -> [w2135]
          tunnel: w2108 -> [w2124]
          stop <- w2119 stop-if-true
          n903 = Concatenate Strings("latencycheck" ("string"), "\r\n") -> (w2131:string)
          n904 = TCP Read(connection ID=w2135, bytes to read=512, error in (no error)=w2136, 7:T15."CRLF" ("mode (standard)"), 9:2000 ("timeout ms (25000)")) -> (connection ID out=w2128:refnum<k5>, data out=w2126:string, error out=w2118:errorcluster)
          n905 = Tick Count (ms)() -> (millisecond timer value=w2125:u32)
          n906 = Subtract(x=w2125, y=w2124) -> (x-y=w2123:u32)
          n907 = Equal?(x=w2126, y=w2131) -> (x = y?=w2127:bool)
          n908 = case shown="False" w2127 {
            tunnel: w2128 -> [_ w2149]
            tunnel: w2126 -> [w2141 _]
            tunnel: [w2137 FALSE] -> w2121
            tunnel: w2118 -> [_ w2143]
            frame False {
              n909 = Concatenate Strings("synctimer" ("string"), "\r\n") -> (w2138:string)
              n910 = Equal?(x=w2141, y=w2138) -> (x = y?=w2137:bool)
              "Sync Success?" <- w2137
            }
            frame True {
              n911 = Concatenate Strings("latencycheck:" ("string"), "\r\n") -> (w2148:string)
              n912 = TCP Write(connection ID=w2149, data in=w2148, error in (no error)=w2143, 9:1000 ("timeout ms (25000)")) -> (error out=w2142:errorcluster)  [unwired: 2 out]
              n913 = call <vilib>:"Clear Errors.vi"("error in (no error)"=w2142) -> ()  [unwired: 5 in, 2 out]
            }
          }
          n914 = Greater?(x=w2123, y=u32 10000 ("x-y")) -> (0:w2120:bool)
          n915 = Or(x=w2121, y=w2120) -> (x .or. y?=w2119:bool)
        }
        n916 = call <vilib>:"Add State(s) to Queue__JKI_lib_State_Machine.vi"("State(s) in (\"\")"=w2117) -> ("States Out"=w2116:string)  [unwired: 14 in]
      }
      frame "TCP: SendSettingMacro" {
        # "Template Separator\n(You can make a copy of, or modify, this frame)"
        n917 = Unbundle By Name(w2153) -> ("CaseID"=w2152:string, "System Status.TCP/IP"=w2151:bool)
        n918 = case shown="True" w2151 {
          tunnel: w2152 -> [_ _]
          tunnel: ["" "TCP: sendSubjectID\nTCP: sendScaleBarSetting\nTCP: sendScaleMaxMin\nTCP: sendDeconChannel\nTCP: sendANSI\nTCP: sendRadius\nTCP: send3Dsetting\nTCP: sendFirefly\nTCP: sendPenrero"] -> w2150
          frame False {
          }
          frame True {
          }
        }
        n919 = call <vilib>:"Add State(s) to Queue__JKI_lib_State_Machine.vi"("State(s) in Front (\"\")"=w2150, "State(s) in (\"\")"=w2157) -> ("States Out"=w2156:string)  [unwired: 13 in]
      }
      frame "TCP: sendRunNum" {
        # "Template Separator\n(You can make a copy of, or modify, this frame)"
        n920 = Unbundle By Name(w2163) -> ("IDs.RunID"=w2170:i8)
        n921 = Number To Decimal String(number=w2170, width (-)=i16 3) -> (decimal integer string=w2165:string)
        n922 = call "TcpIDFGV.vi"("Error In"=w2160, "action"=enum16{"write", "read"}."read") -> ("Error Out"=w2162:errorcluster, "connection ID out"=w2167:refnum<k5>)  [unwired: 8 in]
        n923 = Concatenate Strings("!run:", w2165) -> (w2164:string)
        n924 = call "TCP_WriteRead.vi"("error in (no error)"=w2162, "data in"=w2164, "connectin ID in"=w2167) -> ("error out"=w2161:errorcluster)  [unwired: 4 in, 2 out]
        n925 = call <vilib>:"Add State(s) to Queue__JKI_lib_State_Machine.vi"("State(s) in (\"\")"=w2173) -> ("States Out"=w2172:string)  [unwired: 14 in]
      }
      frame "TCP: sendVideoSource" {
        # "Send video source \n(You can make a copy of, or modify, this frame)"
        n926 = call "TcpIDFGV.vi"("Error In"=w2174, "action"=enum16{"write", "read"}."read") -> ("Error Out"=w2176:errorcluster, "connection ID out"=w2182:refnum<k5>)  [unwired: 8 in]
        n927 = case shown="\"FrameGrabber\"" "Video Source" {
          tunnel: [0 1] -> w2180
          frame "Camera", Default {
          }
          frame "FrameGrabber" {
          }
        }
        n928 = Number To Decimal String(number=w2180) -> (decimal integer string=w2178:string)  [unwired: 1 in]
        n929 = Concatenate Strings("!invivo:" ("data in"), w2178) -> (w2177:string)
        n930 = call "TCP_WriteRead.vi"("error in (no error)"=w2176, "data in"=w2177, "connectin ID in"=w2182) -> ("error out"=w2175:errorcluster)  [unwired: 4 in, 2 out]
        n931 = call <vilib>:"Add State(s) to Queue__JKI_lib_State_Machine.vi"("State(s) in (\"\")"=w2187) -> ("States Out"=w2186:string)  [unwired: 14 in]
      }
      frame "TCP: startRun" {
        # "Template Separator\n(You can make a copy of, or modify, this frame)"
        n932 = call "TcpIDFGV.vi"("Error In"=w2190, "action"=enum16{"write", "read"}."read") -> ("Error Out"=w2192:errorcluster, "connection ID out"=w2193:refnum<k5>)  [unwired: 8 in]
        n933 = call "TCP_WriteRead.vi"("error in (no error)"=w2192, "data in"="!acquire:1", "connectin ID in"=w2193) -> ("error out"=w2191:errorcluster)  [unwired: 4 in, 2 out]
        n934 = call <vilib>:"Add State(s) to Queue__JKI_lib_State_Machine.vi"("State(s) in (\"\")"=w2199) -> ("States Out"=w2198:string)  [unwired: 14 in]
      }
      frame "TCP: stopRun" {
        # "Template Separator\n(You can make a copy of, or modify, this frame)"
        n935 = call "TcpIDFGV.vi"("Error In"=w2200, "action"=enum16{"write", "read"}."read") -> ("Error Out"=w2202:errorcluster, "connection ID out"=w2204:refnum<k5>)  [unwired: 8 in]
        n936 = call "TCP_WriteRead.vi"("error in (no error)"=w2202, "data in"="!acquire:0", "connectin ID in"=w2204) -> ("error out"=w2201:errorcluster)  [unwired: 4 in, 2 out]
        n937 = call <vilib>:"Add State(s) to Queue__JKI_lib_State_Machine.vi"("State(s) in (\"\")"=w2209) -> ("States Out"=w2208:string)  [unwired: 14 in]
      }
      frame "TCP: SyncTimer" {
        # "Template Separator\n(You can make a copy of, or modify, this frame)"
        n938 = call "TcpIDFGV.vi"("Error In"=w2215, "action"=enum16{"write", "read"}."read") -> ("Error Out"=w2216:errorcluster, "connection ID out"=w2217:refnum<k5>)  [unwired: 8 in]
        n939 = while {
          tunnel: w2217 -> [w2236]
          shift-right: [w2231] -> w2211
          shift-left: w2216 -> [w2232]
          tunnel: [w2223] -> w2214
          i -> [w2228]
          stop <- w2226 stop-if-true
          n940 = TCP Read(connection ID=w2236, bytes to read=512, error in (no error)=w2232, 7:T15."CRLF" ("mode (standard)"), 9:1000 ("timeout ms (25000)")) -> (connection ID out=w2223:refnum<k5>, data out=w2230:string, error out=w2231:errorcluster)
          "syctimer data out" <- w2230
          n941 = Equal?(x="!synctimer:", y=w2230) -> (x = y?=w2225:bool)
          n942 = Greater?(x=w2228, y=10000) -> (0:w2224:bool)
          n943 = Or(x=w2225, y=w2224) -> (x .or. y?=w2226:bool)
        }
        n944 = TCP Write(connection ID=w2214, data in="!synctimer:", error in (no error)=w2211, 9:1000 ("timeout ms (25000)")) -> (error out=w2210:errorcluster)  [unwired: 2 out]
        n945 = call <vilib>:"Add State(s) to Queue__JKI_lib_State_Machine.vi"("State(s) in (\"\")"=w2222) -> ("States Out"=w2221:string)  [unwired: 14 in]
      }
      frame "TCP: CheckConnection" {
        # "Check TCP/IP connection statuse\n(If connection is lost, throw error)"
        n946 = Unbundle By Name(w2238) -> ("System Status.TCP/IP"=w2237:bool)
        n947 = case shown="True" w2237 {
          frame False {
          }
          frame True {
            # "If TCP/IP is true check, otherwise skip"
          }
        }
        n948 = call <vilib>:"Add State(s) to Queue__JKI_lib_State_Machine.vi"("State(s) in (\"\")"=w2242) -> ("States Out"=w2241:string)  [unwired: 14 in]
      }
      frame "TCP: Close" {
        # "Close TCP connection\n()"
        n949 = call "TcpIDFGV.vi"("Error In"=w2247, "action"=enum16{"write", "read"}."read") -> ("Error Out"=w2249:errorcluster, "connection ID out"=w2250:refnum<k5>)  [unwired: 8 in]
        n950 = TCP Close Connection(connection ID=w2250, error in (no error)=w2249) -> (error out=w2243:errorcluster)  [unwired: 1 in, 1 out]
        n951 = case shown="No Error" w2243 {
          tunnel: [w2255 w2256] -> w2245
          tunnel: w2244 -> [w2254 w2256]
          frame No Error {
            w2253 = FALSE ("System Status.TCP/IP")
            n952 = Bundle By Name(cluster=w2254, "System Status.TCP/IP"=w2253) -> (w2255:T16)
            n953 = global write "GlobalVariables.vi" "TCP connected?"(w2253) -> ()
          }
          frame Error {
          }
        }
        n954 = call <vilib>:"Add State(s) to Queue__JKI_lib_State_Machine.vi"("State(s) in (\"\")"=w2252) -> ("States Out"=w2251:string)  [unwired: 14 in]
      }
      frame "TCP: sendSubjectID" {
        # "Send subject ID"
        n955 = Unbundle By Name(w2264) -> ("CaseID"=w2263:string)
        n956 = Concatenate Strings("!subject:", w2263) -> (w2260:string)
        n957 = call "TcpIDFGV.vi"("Error In"=w2257, "action"=enum16{"write", "read"}."read") -> ("Error Out"=w2259:errorcluster, "connection ID out"=w2261:refnum<k5>)  [unwired: 8 in]
        n958 = call "TCP_WriteRead.vi"("error in (no error)"=w2259, "data in"=w2260, "connectin ID in"=w2261) -> ("error out"=w2258:errorcluster)  [unwired: 4 in, 2 out]
        n959 = call <vilib>:"Add State(s) to Queue__JKI_lib_State_Machine.vi"("State(s) in (\"\")"=w2268) -> ("States Out"=w2267:string)  [unwired: 14 in]
      }
      frame "TCP: sendScaleBarSetting" {
        # "Template Separator\n(You can make a copy of, or modify, this frame)"
        n960 = call "TcpIDFGV.vi"("Error In"=w2269, "action"=enum16{"write", "read"}."read") -> ("Error Out"=w2271:errorcluster, "connection ID out"=w2273:refnum<k5>)  [unwired: 8 in]
        n961 = call "TCP_WriteRead.vi"("error in (no error)"=w2271, "data in"="!autocolor:0", "connectin ID in"=w2273) -> ("error out"=w2270:errorcluster)  [unwired: 4 in, 2 out]
        n962 = call <vilib>:"Add State(s) to Queue__JKI_lib_State_Machine.vi"("State(s) in (\"\")"=w2278) -> ("States Out"=w2277:string)  [unwired: 14 in]
      }
      frame "TCP: sendScaleMaxMin" {
        # "Template Separator\n(You can make a copy of, or modify, this frame)"
        n963 = call "TcpIDFGV.vi"("Error In"=w2280, "action"=enum16{"write", "read"}."read") -> ("Error Out"=w2282:errorcluster, "connection ID out"=w2283:refnum<k5>)  [unwired: 8 in]
        n964 = call "TCP_WriteRead.vi"("error in (no error)"=w2282, "data in"="!color:3;6", "connectin ID in"=w2283) -> ("error out"=w2281:errorcluster)  [unwired: 4 in, 2 out]
        n965 = call <vilib>:"Add State(s) to Queue__JKI_lib_State_Machine.vi"("State(s) in (\"\")"=w2288) -> ("States Out"=w2287:string)  [unwired: 14 in]
      }
      frame "TCP: sendDeconChannel" {
        # "Send Decon channel\n(You can make a copy of, or modify, this frame)"
        n966 = local read "Radio Buttons"() -> (w2291:enum32{"No Selection", "Ch1", "Ch2", "Ch3"})
        n967 = Increment(x=w2291) -> (x+1=w2290:enum32{"No Selection", "Ch1", "Ch2", "Ch3"})
        n968 = Number To Decimal String(number=w2290) -> (decimal integer string=w2289:string)  [unwired: 1 in]
        n969 = call "TcpIDFGV.vi"("Error In"=w2292, "action"=enum16{"write", "read"}."read") -> ("Error Out"=w2294:errorcluster, "connection ID out"=w2297:refnum<k5>)  [unwired: 8 in]
        n970 = Concatenate Strings("!channel:", w2289) -> (w2295:string)
        n971 = call "TCP_WriteRead.vi"("error in (no error)"=w2294, "data in"=w2295, "connectin ID in"=w2297) -> ("error out"=w2293:errorcluster)  [unwired: 4 in, 2 out]
        n972 = call <vilib>:"Add State(s) to Queue__JKI_lib_State_Machine.vi"("State(s) in (\"\")"=w2302) -> ("States Out"=w2301:string)  [unwired: 14 in]
      }
      frame "TCP: sendANSI" {
        # "Template Separator\n(You can make a copy of, or modify, this frame)"
        n973 = call "TcpIDFGV.vi"("Error In"=w2303, "action"=enum16{"write", "read"}."read") -> ("Error Out"=w2306:errorcluster, "connection ID out"=w2307:refnum<k5>)  [unwired: 8 in]
        n974 = call "TCP_WriteRead.vi"("error in (no error)"=w2306, "data in"="!ansi:20", "connectin ID in"=w2307) -> ("error out"=w2304:errorcluster)  [unwired: 4 in, 2 out]
        n975 = call <vilib>:"Add State(s) to Queue__JKI_lib_State_Machine.vi"("State(s) in (\"\")"=w2312) -> ("States Out"=w2311:string)  [unwired: 14 in]
      }
      frame "TCP: sendRadius" {
        # "Template Separator\n(You can make a copy of, or modify, this frame)"
        n976 = call "TcpIDFGV.vi"("Error In"=w2314, "action"=enum16{"write", "read"}."read") -> ("Error Out"=w2316:errorcluster, "connection ID out"=w2317:refnum<k5>)  [unwired: 8 in]
        n977 = call "TCP_WriteRead.vi"("error in (no error)"=w2316, "data in"="!radius:1.0", "connectin ID in"=w2317) -> ("error out"=w2315:errorcluster)  [unwired: 4 in, 2 out]
        n978 = call <vilib>:"Add State(s) to Queue__JKI_lib_State_Machine.vi"("State(s) in (\"\")"=w2322) -> ("States Out"=w2321:string)  [unwired: 14 in]
      }
      frame "TCP: send3Dsetting" {
        # "Template Separator\n(You can make a copy of, or modify, this frame)"
        n979 = call "TcpIDFGV.vi"("Error In"=w2323, "action"=enum16{"write", "read"}."read") -> ("Error Out"=w2325:errorcluster, "connection ID out"=w2327:refnum<k5>)  [unwired: 8 in]
        n980 = call "TCP_WriteRead.vi"("error in (no error)"=w2325, "data in"="!3dset:0", "connectin ID in"=w2327) -> ("error out"=w2324:errorcluster)  [unwired: 4 in, 2 out]
        n981 = call <vilib>:"Add State(s) to Queue__JKI_lib_State_Machine.vi"("State(s) in (\"\")"=w2332) -> ("States Out"=w2331:string)  [unwired: 14 in]
      }
      frame "TCP: sendFirefly" {
        # "Template Separator\n(You can make a copy of, or modify, this frame)"
        n982 = call "TcpIDFGV.vi"("Error In"=w2333, "action"=enum16{"write", "read"}."read") -> ("Error Out"=w2335:errorcluster, "connection ID out"=w2337:refnum<k5>)  [unwired: 8 in]
        n983 = call "TCP_WriteRead.vi"("error in (no error)"=w2335, "data in"="!firefly:1", "connectin ID in"=w2337) -> ("error out"=w2334:errorcluster)  [unwired: 4 in, 2 out]
        n984 = call <vilib>:"Add State(s) to Queue__JKI_lib_State_Machine.vi"("State(s) in (\"\")"=w2342) -> ("States Out"=w2341:string)  [unwired: 14 in]
      }
      frame "TCP: sendPenrero" {
        # "Template Separator\n(You can make a copy of, or modify, this frame)"
        n985 = call "TcpIDFGV.vi"("Error In"=w2343, "action"=enum16{"write", "read"}."read") -> ("Error Out"=w2345:errorcluster, "connection ID out"=w2347:refnum<k5>)  [unwired: 8 in]
        n986 = call "TCP_WriteRead.vi"("error in (no error)"=w2345, "data in"="!pentero:0", "connectin ID in"=w2347) -> ("error out"=w2344:errorcluster)  [unwired: 4 in, 2 out]
        n987 = call <vilib>:"Add State(s) to Queue__JKI_lib_State_Machine.vi"("State(s) in (\"\")"=w2352) -> ("States Out"=w2351:string)  [unwired: 14 in]
      }
      frame "---------- UI ----------" {
        # "Do not put any code in this frame.\n(It is a separator no-op. You can make a copy of this frame to create a new UI frame)"
        n988 = call <vilib>:"Add State(s) to Queue__JKI_lib_State_Machine.vi"("State(s) in (\"\")"=w2357) -> ("States Out"=w2356:string)  [unwired: 14 in]
      }
      frame "UI: BGLoaded" {
        # "Do not put any code in this frame.\n(It is a separator no-op. You can make a copy of this frame to create a new UI frame)"
        n989 = property on="Background" class="Bool (strict)"("BoolText.Text"="Loaded!" ("Boolean Text.Text"), "Colors [4]"=cluster{u32, u32}[] [{15764023, 15764023}, {16711680, 16711680}]) -> ()  [unwired: 2 in, 2 out]
        n990 = call <vilib>:"Add State(s) to Queue__JKI_lib_State_Machine.vi"("State(s) in (\"\")"=w2364) -> ("States Out"=w2363:string)  [unwired: 14 in]
      }
      frame "UI: CaliAndiRFLoaded" {
        # "Do not put any code in this frame.\n(It is a separator no-op. You can make a copy of this frame to create a new UI frame)"
        n991 = property on="Cali&iRF alignment" class="Bool (strict)"("BoolText.Text"="Loaded!" ("Boolean Text.Text"), "Colors [4]"=cluster{u32, u32}[] [{15764023, 15764023}, {16711680, 16711680}]) -> ()  [unwired: 2 in, 2 out]
        n992 = call <vilib>:"Add State(s) to Queue__JKI_lib_State_Machine.vi"("State(s) in (\"\")"=w2371) -> ("States Out"=w2370:string)  [unwired: 14 in]
      }
      frame "UI: WFAutoScale" {
        # "Set graph auto scale.\n(UI: WFAutoScale >> T/F)"
        n993 = Equal?(x=w2372, y="F") -> (x = y?=w2373:bool)
        n994 = Equal?(x=w2372, y="T") -> (x = y?=w2375:bool)
        n995 = case shown="True" w2373 {
          frame False {
          }
          frame True {
            w2388 = 0.0 ("Y Scale.Range:Maximum")
            w2389 = 2.0 ("Y Scale.Range:Maximum")
            w2390 = u8 0 ("Y Scale.Scale Fit")
            n996 = property on="Channel 1" class="WFGraph (strict)"("YScale.ScaleFit"=w2390) -> (error out=w2387:errorcluster)  [unwired: 2 in, 1 out]
            n997 = property on="Channel 2" class="WFGraph (strict)"("YScale.ScaleFit"=w2390) -> (error out=w2386:errorcluster)  [unwired: 2 in, 1 out]
            n998 = property on="Channel 3" class="WFGraph (strict)"("YScale.ScaleFit"=w2390) -> (error out=w2385:errorcluster)  [unwired: 2 in, 1 out]
            n999 = property on="Channel 1" class="WFGraph (strict)"(error in=w2387, "YScale.Maximum"=w2389) -> (error out=w2384:errorcluster)  [unwired: 1 in, 1 out]
            n1000 = property on="Channel 2" class="WFGraph (strict)"(error in=w2386, "YScale.Maximum"=w2389) -> (error out=w2383:errorcluster)  [unwired: 1 in, 1 out]
            n1001 = property on="Channel 3" class="WFGraph (strict)"(error in=w2385, "YScale.Maximum"=w2389) -> (error out=w2382:errorcluster)  [unwired: 1 in, 1 out]
            n1002 = property on="Channel 1" class="WFGraph (strict)"(error in=w2384, "YScale.Minimum"=w2388) -> ()  [unwired: 1 in, 2 out]
            n1003 = property on="Channel 2" class="WFGraph (strict)"(error in=w2383, "YScale.Minimum"=w2388) -> ()  [unwired: 1 in, 2 out]
            n1004 = property on="Channel 3" class="WFGraph (strict)"(error in=w2382, "YScale.Minimum"=w2388) -> ()  [unwired: 1 in, 2 out]
          }
        }
        n1005 = case shown="True" w2375 {
          frame False {
          }
          frame True {
            w2391 = u8 2 ("Y Scale.Scale Fit")
            n1006 = property on="Channel 1" class="WFGraph (strict)"("YScale.ScaleFit"=w2391) -> ()  [unwired: 2 in, 2 out]
            n1007 = property on="Channel 2" class="WFGraph (strict)"("YScale.ScaleFit"=w2391) -> ()  [unwired: 2 in, 2 out]
            n1008 = property on="Channel 3" class="WFGraph (strict)"("YScale.ScaleFit"=w2391) -> ()  [unwired: 2 in, 2 out]
          }
        }
        n1009 = call <vilib>:"Add State(s) to Queue__JKI_lib_State_Machine.vi"("State(s) in (\"\")"=w2381) -> ("States Out"=w2380:string)  [unwired: 14 in]
      }
      frame "UI: Initialize" {
        w2392 = T29 {"Minimum"=0.0, "Maximum"=4.6, "Increment"=0.1} ("Data Entry Limits")
        w2394 = T10."Disabled and Grayed Out" ("Disabled")
        # "Disable all button on startup"
        # "Initialize the User Interface, here.\n(this is called automatically, by the Macro: Init)"
        n1010 = property on="Gain 1" class="DigNum (strict)"("DisabledEnum"=w2394) -> ()  [unwired: 2 in, 2 out]
        n1011 = property on="Gain 2" class="DigNum (strict)"("DisabledEnum"=w2394) -> ()  [unwired: 2 in, 2 out]
        n1012 = property on="StopButton" class="Bool (strict)"("DisabledEnum"=w2394) -> ()  [unwired: 2 in, 2 out]
        n1013 = property on="Sys Reconfig" class="Bool"("DisabledEnum"=w2394) -> ()  [unwired: 2 in, 2 out]
        n1014 = property on="StartButton" class="Bool (strict)"("DisabledEnum"=w2394) -> ()  [unwired: 2 in, 2 out]
        n1015 = property on="355nm Laser toggle" class="Bool (strict)"("DisabledEnum"=w2394) -> ()  [unwired: 2 in, 2 out]
        n1016 = property on="Aiming beam toggle" class="Bool (strict)"("DisabledEnum"=w2394) -> ()  [unwired: 2 in, 2 out]
        n1017 = property on="Background" class="Bool (strict)"("DisabledEnum"=w2394) -> ()  [unwired: 2 in, 2 out]
        n1018 = property on="Cali&iRF alignment" class="Bool (strict)"("DisabledEnum"=w2394) -> ()  [unwired: 2 in, 2 out]
        n1019 = property on="Gain 3" class="DigNum (strict)"("DisabledEnum"=w2394) -> ()  [unwired: 2 in, 2 out]
        n1020 = property on="Gain 1" class="DigNum (strict)"("Data Range"=w2392) -> ()  [unwired: 2 in, 2 out]
        n1021 = property on="Gain 2" class="DigNum (strict)"("Data Range"=w2392) -> ()  [unwired: 2 in, 2 out]
        n1022 = property on="Gain 3" class="DigNum (strict)"("Data Range"=w2392) -> ()  [unwired: 2 in, 2 out]
        n1023 = call <vilib>:"Add State(s) to Queue__JKI_lib_State_Machine.vi"("State(s) in Front (\"\")"="UI: CaliAndiRFNotReady" ("State(s) in Front (\"\")"), "State(s) in (\"\")"=w2399) -> ("States Out"=w2398:string)  [unwired: 13 in]
      }
      frame "UI: showDisclaimer" {
        # "Show disclamer window.\n(It is a separator no-op. You can make a copy of this frame to create a new UI frame)"
        n1024 = call <vilib>:"Application Directory.vi"() -> ("Application Directory"=w2412:path)
        n1025 = Build Path(base path=w2412, name or relative path="Disclamer.png") -> (appended path=w2410:path)
        n1026 = disable-structure shown="Disabled" {
          frame Disabled {
            n1027 = flat-sequence {
              frame #0 {
                n1028 = call "disclaimer.vi"() -> ()  [unwired: 12 in]
              }
              frame #1 {
                n1029 = Wait (ms)(milliseconds to wait=u32 250) -> ()  [unwired: 1 out]
              }
              frame #2 {
                n1030 = call "SoftwareNote.vi"() -> ()  [unwired: 12 in]
              }
            }
          }
          frame Enabled {
          }
        }
        n1031 = property on="Disclamer" class="Pict"() -> ("Draw Area Size"=w2408:T30)  [unwired: 2 in, 2 out]
        n1032 = call <vilib>:"Read PNG File.vi"("path to PNG file"=w2410) -> ("image data"=w2407:T31)  [unwired: 8 in, 2 out]
        n1033 = Unbundle By Name(w2407) -> ("Rectangle.right"=w2405:i16, "Rectangle.bottom"=w2403:i16)
        n1034 = Unbundle By Name(w2408) -> ("Width"=w2406:u32, "Height"=w2404:u32)
        n1035 = call <vilib>:"Draw Flattened Pixmap.vi"("image data"=w2407) -> ("new picture"=→"Disclamer":picture)  [unwired: 8 in]
        n1036 = Divide(x=w2406, y=w2405) -> (x/y=w2402:dbl)
        n1037 = Divide(x=w2404, y=w2403) -> (x/y=w2401:dbl)
        n1038 = Max & Min(x=w2402, y=w2401) -> (min(x,y)=w2400:dbl)  [unwired: 1 out]
        n1039 = property on="Disclamer" class="Pict"("ZoomFactor"=w2400) -> ()  [unwired: 2 in, 2 out]
        n1040 = call <vilib>:"Add State(s) to Queue__JKI_lib_State_Machine.vi"("State(s) in (\"\")"=w2417) -> ("States Out"=w2416:string)  [unwired: 14 in]
      }
      frame "UI: CaliAndiRFNotReady" {
        # "Do not put any code in this frame.\n(It is a separator no-op. You can make a copy of this frame to create a new UI frame)"
        n1041 = property on="Cali&iRF alignment" class="Bool (strict)"("BoolText.Text"="No Info" ("Boolean Text.Text"), "Colors [4]"=cluster{u32, u32}[] [{13816530, 13816530}, {16711680, 16711680}]) -> ()  [unwired: 2 in, 2 out]
        n1042 = call <vilib>:"Add State(s) to Queue__JKI_lib_State_Machine.vi"("State(s) in (\"\")"=w2425) -> ("States Out"=w2424:string)  [unwired: 14 in]
      }
      frame "UI: BGnotReady" {
        # "Do not put any code in this frame.\n(It is a separator no-op. You can make a copy of this frame to create a new UI frame)"
        n1043 = property on="Background" class="Bool (strict)"("BoolText.Text"="No Info" ("Boolean Text.Text"), "Colors [4]"=cluster{u32, u32}[] [{13816530, 13816530}, {16711680, 16711680}]) -> ()  [unwired: 2 in, 2 out]
        n1044 = call <vilib>:"Add State(s) to Queue__JKI_lib_State_Machine.vi"("State(s) in (\"\")"=w2432) -> ("States Out"=w2431:string)  [unwired: 14 in]
      }
      frame "UI: Reset" {
        w2434 = cluster{u32, u32}[] [{13816530, 13816530}, {13816530, 13816530}] ("Colors [4]")
        # "Do not put any code in this frame.\n(It is a separator no-op. You can make a copy of this frame to create a new UI frame)"
        n1045 = property on="Cali&iRF alignment" class="Bool (strict)"("BoolText.Text"="No Info" ("Boolean Text.Text"), "Colors [4]"=w2434) -> ()  [unwired: 2 in, 2 out]
        n1046 = property on="Background" class="Bool (strict)"("BoolText.Text"="No Info" ("Boolean Text.Text"), "Colors [4]"=w2434) -> ()  [unwired: 2 in, 2 out]
        n1047 = call <vilib>:"Add State(s) to Queue__JKI_lib_State_Machine.vi"("State(s) in (\"\")"=w2440) -> ("States Out"=w2439:string)  [unwired: 14 in]
      }
      frame "UI: SetButtonText" {
        # "Set button text of 355nm laser and aiming beam."
        n1048 = call <vilib>:"Add State(s) to Queue__JKI_lib_State_Machine.vi"("State(s) in (\"\")"=w2445) -> ("States Out"=w2444:string)  [unwired: 14 in]
      }
      frame "UI: DuringAquisition" {
        w2446 = T10."Disabled and Grayed Out" ("Disabled")
        # "Do not put any code in this frame.\n(It is a separator no-op. You can make a copy of this frame to create a new UI frame)"
        n1049 = property on="StopButton" class="Bool (strict)"("DisabledEnum"=T10."Enabled" ("Disabled")) -> ()  [unwired: 2 in, 2 out]
        n1050 = property on="StartButton" class="Bool (strict)"("DisabledEnum"=w2446) -> ()  [unwired: 2 in, 2 out]
        n1051 = property on="Sys Reconfig" class="Bool"("DisabledEnum"=w2446) -> ()  [unwired: 2 in, 2 out]
        n1052 = property on="355nm Laser toggle" class="Bool (strict)"("DisabledEnum"=w2446) -> ()  [unwired: 2 in, 2 out]
        n1053 = property on="Aiming beam toggle" class="Bool (strict)"("DisabledEnum"=w2446) -> ()  [unwired: 2 in, 2 out]
        n1054 = property on="Background" class="Bool (strict)"("DisabledEnum"=w2446) -> ()  [unwired: 2 in, 2 out]
        n1055 = property on="Cali&iRF alignment" class="Bool (strict)"("DisabledEnum"=w2446) -> ()  [unwired: 2 in, 2 out]
        n1056 = property on="Radio Buttons" class="RadioBtnsControl (strict)"("DisabledEnum"=w2446) -> ()  [unwired: 2 in, 2 out]
        n1057 = property on="Video Source" class="RadioBtnsControl (strict)"("DisabledEnum"=w2446) -> ()  [unwired: 2 in, 2 out]
        n1058 = property on="Quit" class="Bool"("DisabledEnum"=w2446) -> ()  [unwired: 2 in, 2 out]
        n1059 = call <vilib>:"Add State(s) to Queue__JKI_lib_State_Machine.vi"("State(s) in (\"\")"=w2452) -> ("States Out"=w2451:string)  [unwired: 14 in]
      }
      frame "UI: duringIRFAlign" {
        w2453 = T10."Disabled and Grayed Out" ("Disabled")
        # "Set UI to during iRF alignment\n(It is a separator no-op. You can make a copy of this frame to create a new UI frame)"
        n1060 = property on="StartButton" class="Bool (strict)"("DisabledEnum"=w2453) -> ()  [unwired: 2 in, 2 out]
        n1061 = property on="Sys Reconfig" class="Bool"("DisabledEnum"=w2453) -> ()  [unwired: 2 in, 2 out]
        n1062 = property on="355nm Laser toggle" class="Bool (strict)"("DisabledEnum"=w2453) -> ()  [unwired: 2 in, 2 out]
        n1063 = property on="Aiming beam toggle" class="Bool (strict)"("DisabledEnum"=w2453) -> ()  [unwired: 2 in, 2 out]
        n1064 = property on="Background" class="Bool (strict)"("DisabledEnum"=w2453) -> ()  [unwired: 2 in, 2 out]
        n1065 = property on="StopButton" class="Bool (strict)"("DisabledEnum"=w2453) -> ()  [unwired: 2 in, 2 out]
        n1066 = call <vilib>:"Add State(s) to Queue__JKI_lib_State_Machine.vi"("State(s) in (\"\")"=w2458) -> ("States Out"=w2457:string)  [unwired: 14 in]
      }
      frame "UI: duringBGAcquire" {
        w2459 = T10."Disabled and Grayed Out" ("Disabled")
        # "Do not put any code in this frame.\n(It is a separator no-op. You can make a copy of this frame to create a new UI frame)"
        n1067 = property on="StartButton" class="Bool (strict)"("DisabledEnum"=w2459) -> ()  [unwired: 2 in, 2 out]
        n1068 = property on="StopButton" class="Bool (strict)"("DisabledEnum"=w2459) -> ()  [unwired: 2 in, 2 out]
        n1069 = property on="Sys Reconfig" class="Bool"("DisabledEnum"=w2459) -> ()  [unwired: 2 in, 2 out]
        n1070 = property on="355nm Laser toggle" class="Bool (strict)"("DisabledEnum"=w2459) -> ()  [unwired: 2 in, 2 out]
        n1071 = property on="Aiming beam toggle" class="Bool (strict)"("DisabledEnum"=w2459) -> ()  [unwired: 2 in, 2 out]
        n1072 = property on="Cali&iRF alignment" class="Bool (strict)"("DisabledEnum"=w2459) -> ()  [unwired: 2 in, 2 out]
        n1073 = call <vilib>:"Add State(s) to Queue__JKI_lib_State_Machine.vi"("State(s) in (\"\")"=w2464) -> ("States Out"=w2463:string)  [unwired: 14 in]
      }
      frame "UI: ReadyForAquisition" {
        w2465 = T10."Enabled" ("Disabled")
        # "Do not put any code in this frame.\n(It is a separator no-op. You can make a copy of this frame to create a new UI frame)"
        n1074 = property on="StopButton" class="Bool (strict)"("DisabledEnum"=T10."Disabled and Grayed Out" ("Disabled")) -> ()  [unwired: 2 in, 2 out]
        n1075 = property on="StartButton" class="Bool (strict)"("DisabledEnum"=w2465) -> ()  [unwired: 2 in, 2 out]
        n1076 = property on="Sys Reconfig" class="Bool"("DisabledEnum"=w2465) -> ()  [unwired: 2 in, 2 out]
        n1077 = property on="355nm Laser toggle" class="Bool (strict)"("DisabledEnum"=w2465) -> ()  [unwired: 2 in, 2 out]
        n1078 = property on="Aiming beam toggle" class="Bool (strict)"("DisabledEnum"=w2465) -> ()  [unwired: 2 in, 2 out]
        n1079 = property on="Cali&iRF alignment" class="Bool (strict)"("DisabledEnum"=w2465) -> ()  [unwired: 2 in, 2 out]
        n1080 = property on="Video Source" class="RadioBtnsControl (strict)"("DisabledEnum"=w2465) -> ()  [unwired: 2 in, 2 out]
        n1081 = property on="Background" class="Bool (strict)"("DisabledEnum"=w2465) -> ()  [unwired: 2 in, 2 out]
        n1082 = property on="Quit" class="Bool"("DisabledEnum"=w2465) -> ()  [unwired: 2 in, 2 out]
        n1083 = property on="Radio Buttons" class="RadioBtnsControl (strict)"("DisabledEnum"=w2465) -> ()  [unwired: 2 in, 2 out]
        n1084 = call <vilib>:"Add State(s) to Queue__JKI_lib_State_Machine.vi"("State(s) in Front (\"\")"="LED: Green" ("State(s) in Front (\"\")"), "State(s) in (\"\")"=w2472) -> ("States Out"=w2471:string)  [unwired: 13 in]
      }
      frame "UI: Update" {
        # "Do not put any code in this frame.\n(It is a separator no-op. You can make a copy of this frame to create a new UI frame)"
        n1085 = Unbundle By Name(w2482) -> ("System Status"=→"System Hardware Connection Status":T1, "IDs.RunID"=→"Run #":i8, "CaseID"=→"Case #":string, "FLImDAQ"=→"FLImDAQ":T22, "SysRunning?"=→"Aquisition Status:":bool, "LJ Pinout"=→"LJ Pinout":T4, "IDs.BG ID"=→"BG #":i8, "IDs.Cali ID"=→"Calibration #":i8)
        n1086 = call <vilib>:"Add State(s) to Queue__JKI_lib_State_Machine.vi"("State(s) in (\"\")"=w2485) -> ("States Out"=w2484:string)  [unwired: 14 in]
      }
      frame "UI: Cursor Set" {
        # "Argument"
        # "Set and Unset Cursor Busy.\n(Usage: \"UI: Cursor Set >> Busy|Idle\")"
        n1087 = case shown="\"Idle\", Default" w2487 {
          tunnel: w2489 -> [w2494 w2496]
          tunnel: [w2493 w2495] -> w2488
          frame "Idle", Default {
            n1088 = call <vilib>:"Unset Busy.vi"("error in (no error)"=w2494) -> ("error out"=w2493:errorcluster)  [unwired: 10 in]
          }
          frame "Busy" {
            n1089 = call <vilib>:"Set Busy.vi"("error in (no error)"=w2496) -> ("error out"=w2495:errorcluster)  [unwired: 9 in, 1 out]
          }
        }
        n1090 = call <vilib>:"Add State(s) to Queue__JKI_lib_State_Machine.vi"("State(s) in (\"\")"=w2492) -> ("States Out"=w2491:string)  [unwired: 14 in]
      }
      frame "UI: Front Panel State" {
        # "Argument"
        # "Set Front Panel Open or Closed\n(Usage: \"UI: Front Panel State >> Open|Close\")"
        n1091 = Unbundle By Name(w2500) -> ("Core.Current VI Reference"=w2499:refnum<vi>)
        n1092 = case shown="\"Open\", \"Standard\", Default" w2498 {
          tunnel: w2502 -> [w2510 w2525 w2536 w2549 w2562]
          tunnel: [w2512 w2526 w2538 w2551 w2564] -> w2501
          tunnel: w2499 -> [w2511 w2523 w2537 w2550 w2563]
          frame "Open", "Standard", Default {
            w2505 = T12."Standard" ("State")
            n1093 = property class="VI"(reference=w2511, error in=w2510) -> (reference out=w2508:refnum<vi>, error out=w2509:errorcluster, "FP.State"=w2507:T12)
            n1094 = Not Equal?(x=w2507, y=w2505) -> (x != y?=w2506:bool)
            n1095 = case shown="True" w2506 {
              tunnel: [w2516 w2518] -> w2512
              tunnel: w2509 -> [w2515 w2518]
              tunnel: w2508 -> [w2514 _]
              tunnel: w2505 -> [w2513 _]
              frame True {
                n1096 = invoke class="VI" method="FP.Open"(reference=w2514, error in=w2515, "Activate"=TRUE, "State"=w2513) -> (error out=w2516:errorcluster)  [unwired: 1 in, 4 out]
              }
              frame False {
              }
            }
          }
          frame "Close", "Closed" {
            n1097 = property class="VI"(reference=w2523, error in=w2525) -> (reference out=w2522:refnum<vi>, error out=w2524:errorcluster, "FP.State"=w2520:T12)
            n1098 = Not Equal?(x=w2520, y=T12."Closed" ("Front Panel Window:State")) -> (x != y?=w2519:bool)
            n1099 = case shown="True" w2519 {
              tunnel: [w2527 w2530] -> w2526
              tunnel: w2524 -> [w2527 w2529]
              tunnel: w2522 -> [_ w2528]
              frame False {
              }
              frame True {
                n1100 = invoke class="VI" method="FP.Close"(reference=w2528, error in=w2529) -> (error out=w2530:errorcluster)  [unwired: 1 in, 2 out]
              }
            }
          }
          frame "Hidden", "Hide" {
            w2531 = T12."Hidden" ("State")
            n1101 = property class="VI"(reference=w2537, error in=w2536) -> (reference out=w2534:refnum<vi>, error out=w2535:errorcluster, "FP.State"=w2533:T12)
            n1102 = Not Equal?(x=w2533, y=w2531) -> (x != y?=w2532:bool)
            n1103 = case shown="True" w2532 {
              tunnel: [w2542 w2543] -> w2538
              tunnel: w2535 -> [w2541 w2543]
              tunnel: w2534 -> [w2540 _]
              tunnel: w2531 -> [w2539 _]
              frame True {
                n1104 = invoke class="VI" method="FP.Open"(reference=w2540, error in=w2541, "State"=w2539) -> (error out=w2542:errorcluster)  [unwired: 2 in, 4 out]
              }
              frame False {
              }
            }
          }
          frame "Minimize", "Minimized" {
            w2544 = T12."Minimized" ("State")
            n1105 = property class="VI"(reference=w2550, error in=w2549) -> (reference out=w2547:refnum<vi>, error out=w2548:errorcluster, "FP.State"=w2546:T12)
            n1106 = Not Equal?(x=w2546, y=w2544) -> (x != y?=w2545:bool)
            n1107 = case shown="True" w2545 {
              tunnel: [w2555 w2556] -> w2551
              tunnel: w2548 -> [w2554 w2556]
              tunnel: w2547 -> [w2553 _]
              tunnel: w2544 -> [w2552 _]
              frame True {
                n1108 = invoke class="VI" method="FP.Open"(reference=w2553, error in=w2554, "State"=w2552) -> (error out=w2555:errorcluster)  [unwired: 2 in, 4 out]
              }
              frame False {
              }
            }
          }
          frame "Maximize", "Maximized" {
            w2557 = T12."Maximized" ("State")
            n1109 = property class="VI"(reference=w2563, error in=w2562) -> (reference out=w2560:refnum<vi>, error out=w2561:errorcluster, "FP.State"=w2559:T12)
            n1110 = Not Equal?(x=w2559, y=w2557) -> (x != y?=w2558:bool)
            n1111 = case shown="True" w2558 {
              tunnel: [w2568 w2569] -> w2564
              tunnel: w2561 -> [w2567 w2569]
              tunnel: w2560 -> [w2566 _]
              tunnel: w2557 -> [w2565 _]
              frame True {
                n1112 = invoke class="VI" method="FP.Open"(reference=w2566, error in=w2567, "State"=w2565) -> (error out=w2568:errorcluster)  [unwired: 2 in, 4 out]
              }
              frame False {
              }
            }
          }
        }
        n1113 = call <vilib>:"Add State(s) to Queue__JKI_lib_State_Machine.vi"("State(s) in (\"\")"=w2504) -> ("States Out"=w2503:string)  [unwired: 14 in]
      }
      frame "---------- 355 Laser ----------" {
        # "Template Separator\n(You can make a copy of, or modify, this frame)"
        n1114 = call <vilib>:"Add State(s) to Queue__JKI_lib_State_Machine.vi"("State(s) in (\"\")"=w2574) -> ("States Out"=w2573:string)  [unwired: 14 in]
      }
      frame "355 Laser: Check Dewelling" {
        # "if time laser start time is less than 7.5s before, wait 250ms then check again."
        # "Template Separator\n(You can make a copy of, or modify, this frame)"
        n1115 = Unbundle By Name(w2582) -> ("Laser start tic"=w2579:u32)
        n1116 = Tick Count (ms)() -> (millisecond timer value=w2580:u32)
        n1117 = Subtract(x=w2580, y=w2579) -> (x-y=w2578:u32)
        n1118 = Greater?(x=w2578, y=u32 5000) -> (0:w2576:bool)
        n1119 = case shown="False" w2576 {
          tunnel: ["355 Laser: Check Dewelling" ""] -> w2575
          frame False {
            n1120 = Wait (ms)(milliseconds to wait=u32 250) -> ()  [unwired: 1 out]
          }
          frame True {
          }
        }
        n1121 = call <vilib>:"Add State(s) to Queue__JKI_lib_State_Machine.vi"("State(s) in Front (\"\")"=w2575, "State(s) in (\"\")"=w2585) -> ("States Out"=w2584:string)  [unwired: 13 in]
      }
      frame "355 Laser: Laser enable/disable" {
        # "Laser enable/disable\n(Usage: \"LabJack: Laser enable/disable >> 1|0\")"
        n1122 = Unbundle By Name(w2590) -> ("LJ Pinout.Laser Start/Stop"=w2598:string)
        n1123 = call "LabJack_FGV.vi"("Operation(Read)"=enum16{"Write", "Read"}."Read" ("Operation")) -> ("Read data"=w2600:i32)  [unwired: 9 in, 1 out]
        n1124 = call "LJM_eWriteName.vi"("Handle In"=w2600, "Name"=w2598, "Value"=1.0, "error in"=w2604) -> ("Handle Out"=w2599:i32, "error out"=w2597:errorcluster)  [unwired: 10 in]
        n1125 = call <userlib>:"Wait (ms)__ogtk.vi"("error in (no error)"=w2597, "milliseconds to wait"=u32 250) -> ("error out"=w2596:errorcluster)  [unwired: 8 in, 1 out]
        n1126 = call "LJM_eWriteName.vi"("Handle In"=w2599, "Name"=w2598, "Value"=0.0, "error in"=w2596) -> ("error out"=w2593:errorcluster)  [unwired: 10 in, 1 out]
        n1127 = call <userlib>:"Tick Count (ms)__ogtk.vi"("error in (no error)"=w2593) -> ("error out"=w2592:errorcluster, "millisecond timer value"=w2589:u32)  [unwired: 9 in]
        n1128 = Bundle By Name(cluster=w2590, "Laser start tic"=w2589) -> (w2591:T16)
        n1129 = call <vilib>:"Add State(s) to Queue__JKI_lib_State_Machine.vi"("State(s) in (\"\")"=w2606) -> ("States Out"=w2605:string)  [unwired: 14 in]
      }
      frame "355 Laser: Dewelling" {
        # "Wait some time (ms)\n(355 Laser: Dewelling >> #)"
        n1130 = Fract/Exp String To Number(string=w2610, default (0 dbl)=0) -> (number=w2608:i32)  [unwired: 2 in, 1 out]
        n1131 = Wait (ms)(milliseconds to wait=w2608) -> ()  [unwired: 1 out]
        n1132 = call <vilib>:"Add State(s) to Queue__JKI_lib_State_Machine.vi"("State(s) in (\"\")"=w2614) -> ("States Out"=w2613:string)  [unwired: 14 in]
      }
      frame "355 Laser: Init" {
        # "Initilize 355nm laser\n(Start laser, enable interlock)"
        n1133 = call <vilib>:"Add State(s) to Queue__JKI_lib_State_Machine.vi"("State(s) in Front (\"\")"="355 Laser: CheckControllerStatus", "State(s) in (\"\")"=w2620) -> ("States Out"=w2619:string)  [unwired: 13 in]
      }
      frame "355 Laser: Close" {
        # "Template Separator\n(You can make a copy of, or modify, this frame)"
        n1134 = call <vilib>:"Add State(s) to Queue__JKI_lib_State_Machine.vi"("State(s) in Front (\"\")"="355 Laser: Laser enable/disable\n355 Laser: Dewelling >>1000", "State(s) in (\"\")"=w2626) -> ("States Out"=w2625:string)  [unwired: 13 in]
      }
      frame "355 Laser: CheckControllerStatus" {
        # "if average < 1, laser on\nif average > 9, laser off\nif 1<average<9, interlock open, blink indicator"
        # "take 10 measuremt and look at average"
        # "Check 355 laser controller status\nBy probing Emisison Lamp negative terminal voltage"
        n1135 = Unbundle By Name(w2634) -> ("LJ Pinout.Laser Ready"=w2637:string)
        n1136 = call "LabJack_FGV.vi"("Operation(Read)"=enum16{"Write", "Read"}."Read" ("Operation")) -> ("Read data"=w2638:i32)  [unwired: 9 in, 1 out]
        n1137 = for {
          N: 10 -> [_]
          tunnel: w2638 -> [w2672]
          tunnel: w2637 -> [w2671]
          shift-right: [w2670] -> w2629
          shift-left: w2636 -> [w2669]
          tunnel: [w2667] -> w2627 mode=indexing
          n1138 = call "LJM_eReadName.vi"("Handle In"=w2672, "Name"=w2671, "error in"=w2669) -> ("Value"=w2667:dbl, "error out"=w2670:errorcluster)  [unwired: 10 in, 1 out]
          n1139 = Wait (ms)(milliseconds to wait=u32 50) -> ()  [unwired: 1 out]
        }
        n1140 = case shown="No Error" w2629 {
          selector: w2629 -> [w2646 w2665]
          tunnel: [w2648 FALSE] -> w2631
          tunnel: [w2647 w2665] -> w2630
          tunnel: [w2642 nan] -> w2628
          tunnel: w2627 -> [w2644 _]
          frame No Error {
            n1141 = call-poly <vilib>:"Mean.vi"("X"=w2644) -> ("mean"=w2642:dbl)  [unwired: 1 out]
            n1142 = Less?(x=w2642, y=2.0) -> (x < y?=w2643:bool)
            n1143 = case shown="False" w2643 {
              tunnel: [w2651 TRUE] -> w2648
              tunnel: w2642 -> [w2654 _]
              tunnel: w2646 -> [w2650 w2661]
              tunnel: [w2649 w2661] -> w2647
              frame False {
                n1144 = Greater?(x=w2654, y=9.0) -> (0:w2652:bool)
                n1145 = case shown="False" w2652 {
                  tunnel: [FALSE FALSE] -> w2651
                  tunnel: w2650 -> [_ w2658]
                  tunnel: [errorcluster {"status"=TRUE, "code"=5002, "source"="355 Laser"} ("error out") w2658] -> w2649
                  frame False {
                    n1146 = property on="355 Laser" class="Bool (strict)"("Blinking"=FALSE) -> ()  [unwired: 2 in, 2 out]
                  }
                  frame True {
                    n1147 = property on="355 Laser" class="Bool (strict)"("Blinking"=FALSE) -> ()  [unwired: 2 in, 2 out]
                  }
                }
              }
              frame True {
                n1148 = property on="355 Laser" class="Bool (strict)"("Blinking"=FALSE) -> ()  [unwired: 2 in, 2 out]
              }
            }
          }
          frame Error {
          }
        }
        "laser EM lamp V" <- w2628
        n1149 = Bundle By Name(cluster=w2634, "System Status.355 Laser"=w2631) -> (w2635:T16)
        n1150 = call <vilib>:"Add State(s) to Queue__JKI_lib_State_Machine.vi"("State(s) in (\"\")"=w2641) -> ("States Out"=w2640:string)  [unwired: 14 in]
      }
      frame "355 Laser: CheckPWMStatus" {
        # "Check 355 laser PWM status\n(Read LJ DIO#EF_ENABLE register to determine PWM status)"
        n1151 = Unbundle By Name(w2682) -> ("LJ Pinout.355 PWM"=w2681:string)
        n1152 = call "LabJack_FGV.vi"("Operation(Read)"=enum16{"Write", "Read"}."Read" ("Operation"), "error in (no error)"=w2675) -> ("error out"=w2678:errorcluster, "Read data"=w2679:i32)  [unwired: 8 in]
        n1153 = Concatenate Strings(w2681, "_EF_ENABLE" ("string")) -> (w2677:string)
        n1154 = call "LJM_eReadName.vi"("Handle In"=w2679, "Name"=w2677, "error in"=w2678) -> ("Value"=w2674:dbl, "error out"=w2676:errorcluster)  [unwired: 10 in, 1 out]
        n1155 = Greater Than 0?(x=w2674) -> (x > 0?=w2673:bool)
        n1156 = case shown="True" w2673 {
          frame False {
            # "PWM is off\nset color to dark green"
            n1157 = local write "355nm Laser toggle"(FALSE ("355nm Laser")) -> ()
          }
          frame True {
            # "PWM is on\nset color to light green"
            n1158 = local write "355nm Laser toggle"(TRUE ("355nm Laser")) -> ()
          }
        }
        n1159 = call <vilib>:"Add State(s) to Queue__JKI_lib_State_Machine.vi"("State(s) in (\"\")"=w2686) -> ("States Out"=w2685:string)  [unwired: 14 in]
      }
      frame "355 Laser: Start" {
        # "Template Separator\n(You can make a copy of, or modify, this frame)"
        n1160 = call <vilib>:"Add State(s) to Queue__JKI_lib_State_Machine.vi"("State(s) in Front (\"\")"="LabJack: 355_PWM_Start", "State(s) in (\"\")"=w2694) -> ("States Out"=w2693:string)  [unwired: 13 in]
      }
      frame "355 Laser: Stop" {
        # "Template Separator\n(You can make a copy of, or modify, this frame)"
        n1161 = call <vilib>:"Add State(s) to Queue__JKI_lib_State_Machine.vi"("State(s) in Front (\"\")"="LabJack: 355_PWM_Stop", "State(s) in (\"\")"=w2700) -> ("States Out"=w2699:string)  [unwired: 13 in]
      }
      frame "---------- Utility ----------" {
        # "Template Separator\n(You can make a copy of, or modify, this frame)"
        n1162 = call <vilib>:"Add State(s) to Queue__JKI_lib_State_Machine.vi"("State(s) in (\"\")"=w2705) -> ("States Out"=w2704:string)  [unwired: 14 in]
      }
      frame "Utility: RestoreDeConChan" {
        # "Template Separator\n(You can make a copy of, or modify, this frame)"
        n1163 = global read "GlobalVariables.vi" "DeconChan Temp"() -> (w2706:T32)
        n1164 = local write "Radio Buttons"(w2706) -> ()
        n1165 = call <vilib>:"Add State(s) to Queue__JKI_lib_State_Machine.vi"("State(s) in (\"\")"=w2711) -> ("States Out"=w2710:string)  [unwired: 14 in]
      }
      frame "Utility: SaveDeconChan" {
        # "Save Decon Channel to global temp\n(You can make a copy of, or modify, this frame)"
        n1166 = flat-sequence {
          frame #0 {
          }
          frame #1 {
            (unwired) enum32{"No Selection", "Ch1", "Ch2", "Ch3"}."No Selection" ("Radio Buttons")
          }
        }
        n1167 = flat-sequence {
          frame #0 {
            n1168 = local read "Radio Buttons"() -> (w2717:enum32{"No Selection", "Ch1", "Ch2", "Ch3"})
            n1169 = global write "GlobalVariables.vi" "DeconChan Temp"(w2717) -> ()
          }
          frame #1 {
            n1170 = local write "Radio Buttons"(enum32{"No Selection", "Ch1", "Ch2", "Ch3"}."No Selection" ("Radio Buttons")) -> ()
          }
        }
        n1171 = call <vilib>:"Add State(s) to Queue__JKI_lib_State_Machine.vi"("State(s) in (\"\")"=w2716) -> ("States Out"=w2715:string)  [unwired: 14 in]
      }
      frame "Utility: Dewelling" {
        # "Main loop dewell\n(Dewelling >> #)"
        n1172 = Fract/Exp String To Number(string=w2721, default (0 dbl)=0) -> (number=w2719:i32)  [unwired: 2 in, 1 out]
        n1173 = Wait (ms)(milliseconds to wait=w2719) -> ()  [unwired: 1 out]
        n1174 = call <vilib>:"Add State(s) to Queue__JKI_lib_State_Machine.vi"("State(s) in (\"\")"=w2726) -> ("States Out"=w2725:string)  [unwired: 14 in]
      }
      frame "Utility: SetAllChanManualGain" {
        # "Template Separator\n(You can make a copy of, or modify, this frame)"
        n1175 = property on="Auto gain ch1" class="Bool (strict)"("Val(Sgnl)"=FALSE ("Value (Signaling)")) -> ()  [unwired: 2 in, 2 out]
        n1176 = property on="Auto gain ch2" class="Bool (strict)"("Val(Sgnl)"=FALSE ("Value (Signaling)")) -> ()  [unwired: 2 in, 2 out]
        n1177 = property on="Auto gain ch3" class="Bool (strict)"("Val(Sgnl)"=FALSE ("Value (Signaling)")) -> ()  [unwired: 2 in, 2 out]
        n1178 = call <vilib>:"Add State(s) to Queue__JKI_lib_State_Machine.vi"("State(s) in (\"\")"=w2734) -> ("States Out"=w2733:string)  [unwired: 14 in]
      }
      frame "Utility: SetAllChanAutoGain" {
        # "Template Separator\n(You can make a copy of, or modify, this frame)"
        n1179 = property on="Auto gain ch1" class="Bool (strict)"("Val(Sgnl)"=TRUE ("Value (Signaling)")) -> ()  [unwired: 2 in, 2 out]
        n1180 = property on="Auto gain ch2" class="Bool (strict)"("Val(Sgnl)"=TRUE ("Value (Signaling)")) -> ()  [unwired: 2 in, 2 out]
        n1181 = property on="Auto gain ch3" class="Bool (strict)"("Val(Sgnl)"=TRUE ("Value (Signaling)")) -> ()  [unwired: 2 in, 2 out]
        n1182 = call <vilib>:"Add State(s) to Queue__JKI_lib_State_Machine.vi"("State(s) in (\"\")"=w2742) -> ("States Out"=w2741:string)  [unwired: 14 in]
      }
      frame "---------- SysLog ----------" {
        # "Template Separator\n(You can make a copy of, or modify, this frame)"
        n1183 = call <vilib>:"Add State(s) to Queue__JKI_lib_State_Machine.vi"("State(s) in (\"\")"=w2747) -> ("States Out"=w2746:string)  [unwired: 14 in]
      }
      frame "SysLog: OpenLogFile" {
        # "Template Separator\n(You can make a copy of, or modify, this frame)"
        n1184 = call <vilib>:"Add State(s) to Queue__JKI_lib_State_Machine.vi"("State(s) in (\"\")"=w2752) -> ("States Out"=w2751:string)  [unwired: 14 in]
      }
      frame "---------- Graph ----------" {
        # "Template Separator\n(You can make a copy of, or modify, this frame)"
        n1185 = call <vilib>:"Add State(s) to Queue__JKI_lib_State_Machine.vi"("State(s) in (\"\")"=w2757) -> ("States Out"=w2756:string)  [unwired: 14 in]
      }
      frame "Graph: AddCursors" {
        # "Add BG and DC cursor to all graphs\n(You can make a copy of, or modify, this frame)"
        n1186 = property on="Channel 2" class="WFGraph (strict)"() -> ("CrsrList"=w2761:T17)  [unwired: 2 in, 2 out]
        n1187 = property on="Channel 3" class="WFGraph (strict)"() -> ("CrsrList"=w2760:T17)  [unwired: 2 in, 2 out]
        n1188 = property on="Channel 1" class="WFGraph (strict)"() -> ("CrsrList"=w2765:T17)  [unwired: 2 in, 2 out]
        n1189 = for {
          tunnel: w2765 -> [w2778] mode=indexing
          tunnel: u32[] [200, 220, 10, 25] -> [w2774] mode=indexing
          tunnel: [w2777] -> w2763 mode=indexing
          tunnel: u32[] [6618880, 6618880, 16711680, 16711680] -> [w2773] mode=indexing
          tunnel: w2761 -> [w2776] mode=indexing
          tunnel: w2760 -> [w2775] mode=indexing
          tunnel: [w2772] -> w2759 mode=indexing
          tunnel: [w2771] -> w2758 mode=indexing
          n1190 = Bundle By Name(cluster=w2778, "Position.X"=w2774, "Color"=w2773) -> (w2777:T18)
          n1191 = Bundle By Name(cluster=w2776, "Position.X"=w2774, "Color"=w2773) -> (w2772:T18)
          n1192 = Bundle By Name(cluster=w2775, "Position.X"=w2774, "Color"=w2773) -> (w2771:T18)
        }
        n1193 = property on="Channel 1" class="WFGraph (strict)"("CrsrList"=w2763) -> ()  [unwired: 2 in, 2 out]
        n1194 = property on="Channel 2" class="WFGraph (strict)"("CrsrList"=w2759) -> ()  [unwired: 2 in, 2 out]
        n1195 = property on="Channel 3" class="WFGraph (strict)"("CrsrList"=w2758) -> ()  [unwired: 2 in, 2 out]
        n1196 = call <vilib>:"Add State(s) to Queue__JKI_lib_State_Machine.vi"("State(s) in (\"\")"=w2770) -> ("States Out"=w2769:string)  [unwired: 14 in]
      }
      frame "---------- Temp ----------" {
        # "Template Separator\n(You can make a copy of, or modify, this frame)"
        n1197 = call <vilib>:"Add State(s) to Queue__JKI_lib_State_Machine.vi"("State(s) in (\"\")"=w2783) -> ("States Out"=w2782:string)  [unwired: 14 in]
      }
    }
    n1198 = Not(x=w270) -> (.not. x?=w269:bool)
    n1199 = local write "ML?"(w269) -> ()
    "ML?" <- TRUE ("main loop running?")
  }
  n1200 = while {
    tunnel: w43 -> [w2796]
    tunnel: w32 -> [w2795]
    tunnel: [w2794] -> w41
    tunnel: w26 -> [w2793]
    tunnel: [w2792] -> w37
    tunnel: w8 -> [w2790]
    tunnel: w19 -> [w2789]
    tunnel: w3 -> [w2784]
    stop <- w2787 stop-if-true
    # "Data Aquisition Loop"
    n1201 = event shown="[1] <Start digitizer>: User Event" {
      selector: w2795 -> [_ _]
      dyn-events: [_ _] -> w2794
      timeout: 20 -> [_ _]
      tunnel: w2796 -> [w2802 w2807]
      tunnel: [w2797 _] -> w2787
      tunnel: w2793 -> [w2801 w2814]
      tunnel: [w2801 w2813] -> w2792
      tunnel: w2790 -> [_ w2811]
      tunnel: w2789 -> [w2800 w2806]
      tunnel: w2784 -> [_ w2803]
      event Timeout {
        # "use queue to stop data loop\nwhen queue ref is released, error will stop this loop"
        n1202 = event-data() -> ()  [unwired: 1 in, 3 out]
        n1203 = Get Queue Status(queue=w2800) -> (error out=w2798:errorcluster)  [unwired: 2 in, 7 out]
        n1204 = Get Queue Status(queue=w2802) -> (error out=w2799:errorcluster)  [unwired: 2 in, 7 out]
        n1205 = Merge Errors(w2799, w2798) -> (w2797:errorcluster)
      }
      event User Event {
        w2812 = enum16{"Write", "Read"}."Read" ("Operation")
        n1206 = event-data() -> ()  [unwired: 1 in, 4 out]
        n1207 = call "FLImDAQ_FGV.vi"() -> ("Read data"=w2809:T5)  [unwired: 10 in, 1 out]
        n1208 = Unbundle By Name(w2809) -> ("Waveform to Avg"=w2808:i16)
        n1209 = call "Digitizer1_FGV.vi"("Operation (Read)"=w2812) -> ("Read data"=w2804:refnum<k15>)  [unwired: 9 in, 1 out]
        n1210 = call "Digitizer2_FGV.vi"("Operation (Read)"=w2812) -> ("Read data"=w2810:refnum<k15>)  [unwired: 9 in, 1 out]
        n1211 = while {
          tunnel: w2814 -> [w2861]
          tunnel: [w2860] -> w2813
          tunnel: w2810 -> [w2854]
          tunnel: w2804 -> [w2853]
          tunnel: w2811 -> [w2851]
          shift-right: [w2840] -> _
          shift-left: u32 0 ("millisecond timer value") -> [w2839]
          tunnel: w2808 -> [w2836]
          tunnel: w2807 -> [w2833]
          tunnel: w2806 -> [w2831]
          tunnel: w2803 -> [w2818]
          i -> [w2835]
          stop <- w2826 stop-if-true
          w2823 = enum16{"write", "read"}."read" ("action")
          w2841 = 65536
          # "send data for processing"
          # "acquire data and send it to processing loop"
          n1212 = Tick Count (ms)() -> (millisecond timer value=w2840:u32)
          n1213 = Multiply(x=w2836, y=w2835) -> (x*y=w2815:i32)
          "Fetch Record #" <- w2815
          n1214 = Subtract(x=w2840, y=w2839) -> (x-y=→"Aquisition loop timing(ms)":u32)
          n1215 = property class="niScope"(reference=w2853, "Fetch Record Number"=w2815) -> (reference out=w2865:refnum<k15>, error out=w2864:errorcluster, "Records Done"=w2816:i32, "Vertical Range"=w2849:dbl, "Vertical Offset"=w2847:dbl)  [unwired: 1 in]
          n1216 = call-poly <instrlib>:"niScope Fetch (poly).vi"("timeout"=1.0, "error in"=w2864, "channels"="0,1", "instrument handle"=w2865) -> ("error out"=w2852:errorcluster, "wfm"=w2837:i16[][])  [unwired: 4 in, 2 out]
          "error out" <- w2852
          n1217 = property class="niScope"(reference=w2854, error in=w2852, "Fetch Record Number"=w2815) -> (reference out=w2858:refnum<k15>, error out=w2855:errorcluster, "Vertical Range"=w2843:dbl, "Vertical Offset"=w2842:dbl)
          n1218 = Divide(x=w2837, y=w2841) -> (x/y=w2850:dbl[][])
          n1219 = Subtract(x=w2816, y=w2815) -> (x-y=→"Record Backlog":i32)
          n1220 = Multiply(x=w2850, y=w2849) -> (x*y=w2848:dbl[][])
          n1221 = call "V1FGV.vi"("action (write)"=w2823) -> ("Error Out"=w2825:errorcluster, "V1 out"=w2822:dbl)  [unwired: 9 in]
          n1222 = call-poly <instrlib>:"niScope Fetch (poly).vi"("timeout"=1.0, "error in"=w2855, "channels"="0,1", "instrument handle"=w2858) -> ("error out"=w2829:errorcluster, "wfm"=w2844:i16[][])  [unwired: 4 in, 2 out]
          "error out 2" <- w2829
          n1223 = call "V2FGV.vi"("Error In"=w2825, "action(write)"=w2823) -> ("Error Out"=w2824:errorcluster, "V2 out"=w2821:dbl)  [unwired: 8 in]
          n1224 = Add(x=w2848, y=w2847) -> (x+y=w2832:dbl[][])
          n1225 = call "V3FGV.vi"("Error In"=w2824, "action(write)"=w2823) -> ("V3 out"=w2820:dbl)  [unwired: 8 in, 1 out]
          n1226 = Divide(x=w2844, y=w2841) -> (x/y=w2846:dbl[][])
          n1227 = Enqueue Element(queue=w2833, element=w2832) -> (error out=w2828:errorcluster)  [unwired: 2 in, 2 out]
          n1228 = Bundle("V1 out"=w2822, "V2 out"=w2821, "V3 out"=w2820) -> (w2819:T33)  [unwired: 1 in]
          n1229 = Multiply(x=w2846, y=w2843) -> (x*y=w2845:dbl[][])
          n1230 = Add(x=w2845, y=w2842) -> (x+y=w2830:dbl[][])
          n1231 = Enqueue Element(queue=w2818, element=w2819) -> (error out=w2817:errorcluster)  [unwired: 2 in, 2 out]
          n1232 = Enqueue Element(queue=w2831, element=w2830) -> (error out=w2827:errorcluster)  [unwired: 2 in, 2 out]
          n1233 = Bundle(w2835, w2832, w2830) -> (w2834:cluster{i32, dbl[][], dbl[][]})  [unwired: 1 in]
          n1234 = Merge Errors(w2817, w2827, w2828, w2829) -> (w2826:errorcluster)
          "aquisition loop Error Out" <- w2826
          n1235 = Send Notification(notification=w2834, notifier=w2861) -> (notifier out=w2860:refnum<notifier>)  [unwired: 1 in, 1 out]
          n1236 = case shown="Error .." w2826 {
            tunnel: w2851 -> [_ w2868]
            frame No Error {
            }
            frame Error {
              # "Send user event to signal aquisition has stoped"
              n1237 = Generate User Event(priority (normal)=usereventprio."high priority", user event=w2868, event data cluster=TRUE ("event data")) -> ()  [unwired: 1 in, 2 out]
            }
          }
        }
      }
    }
    n1238 = Unbundle By Name(w2787) -> ("status"=w2786:bool)
    n1239 = Not(x=w2786) -> (.not. x?=w2785:bool)
    n1240 = local write "Aq L?"(w2785) -> ()
    "Aq L?" <- TRUE ("Aq L?")
  }
  n1241 = Control Help Window(0:w1, 1:TRUE ("Show")) -> ()
  n1242 = Unregister For Events(event registration refnum=w17, error in=w28) -> (error out=w29:errorcluster)
  n1243 = Destroy User Event(user event=w8, error in=w29) -> ()  [unwired: 1 out]
  n1244 = Release Notifier(notifier=w37, error in (no error)=w36) -> (error out=w35:errorcluster)  [unwired: 1 in, 2 out]
  n1245 = Unregister For Events(event registration refnum=w41, error in=w39) -> (error out=w40:errorcluster)
  n1246 = Release Notifier(notifier=w22, error in (no error)=w20) -> (error out=w21:errorcluster)  [unwired: 1 in, 2 out]
  n1247 = Release Notifier(notifier=w13, error in (no error)=w7) -> (error out=w12:errorcluster)  [unwired: 1 in, 2 out]
  n1248 = call <vilib>:"Simple Error Handler.vi"("error in (no error)"=w35) -> ()  [unwired: 4 in, 5 out]
  n1249 = Destroy User Event(user event=w30, error in=w40) -> ()  [unwired: 1 out]
  n1250 = call <vilib>:"Simple Error Handler.vi"("error in (no error)"=w21) -> ()  [unwired: 4 in, 5 out]
  n1251 = call <vilib>:"Simple Error Handler.vi"("error in (no error)"=w12) -> ()  [unwired: 4 in, 5 out]
  n1252 = disable-structure shown="Disabled" {
    frame Disabled {
      n1253 = flat-sequence {
        tunnel: _ -> [w2869]
        tunnel: _ -> [w2874]
        frame #0 {
          n1254 = Two Button Dialog(message="Save data?", 1:"No" ("F button name (\"Cancel\")"), 2:"Yes" ("T button name (\"OK\")")) -> (T button?=w2870:bool)
          n1255 = case shown="True" w2870 {
            tunnel: w2874 -> [_ w2876]
            tunnel: w2869 -> [_ w2875]
            frame False {
            }
            frame True {
              n1256 = flat-sequence {
                tunnel: w2876 -> [w2877]
                tunnel: w2875 -> [w2879]
                frame #0 {
                  n1257 = call-poly <vilib>:"Write Delimited Spreadsheet.vi"("format (%.3f)"="%.6f", "2D data"=w2877) -> ()  [unwired: 12 in, 2 out]
                }
                frame #1 {
                  n1258 = call-poly <vilib>:"Write Delimited Spreadsheet.vi"("format (%.3f)"="%.6f", "1D data"=w2879, "delimiter (\\t)"="\r\n") -> ()  [unwired: 11 in, 2 out]
                }
              }
            }
          }
        }
      }
    }
    frame Enabled {
    }
  }
